vi "Cascade front panel.vi"() -> ()   [LabVIEW 2016]
uses:
  sdi_12/SDI-12/Sonde Vertical Graph.ctl
  controls/Vertical Chart.ctl
  sdi_12/Groundwater header.ctl
  controls/MCC DAQ Setup.ctl
  controls/Aux Sensor.ctl
  KPRO_2016 subvis/Control 2.ctl
  KPRO_2016 subvis/Graph Controls 2.ctl
  KPRO_2016 subvis/Ik control.ctl
  controls/MCC DAQ Readings.ctl
  controls/Kpro pressure measurement cluster.ctl
  controls/Kpro hydraulic measurement cluster.ctl
  activeXtest/activeXtest 2015 Folder/sonde cluster from excel.ctl
  sdi_12/Sonde Value Percent Tol.ctl
  activeXtest/activeXtest 2015 Folder/sample data row cluster.ctl
  activeXtest/activeXtest 2015 Folder/sonde cluster.ctl
  KPRO_2016 subvis/Sensor Physical Measurements.ctl
  KPRO_2016 subvis/SS Control 7.ctl
  controls/Action Control 1.ctl
  <extravilib>/ChannelInstances/One Element Stream-t'Action Control 1.ctl'/Instantiate.vi
  <extravilib>/ChannelInstances/One Element Stream-t'Action Control 1.ctl'/Endpoint.vi
  KPRO_lv2015/Kpro Globals.vi
  C/Program Files (x86)/National Instruments/LabVIEW 2016/user.lib/_OpenG.lib/file/file.llb/Strip Path - Traditional__ogtk.vi
  C/Program Files (x86)/National Instruments/LabVIEW 2016/user.lib/_OpenG.lib/file/file.llb/Build Path - Traditional__ogtk.vi
  <vilib>/Utility/file.llb/Write Delimited Spreadsheet (DBL).vi
  C/Program Files (x86)/National Instruments/LabVIEW 2016/user.lib/_OpenG.lib/file/file.llb/Strip Path Extension - Path__ogtk.vi
  C/Program Files (x86)/National Instruments/LabVIEW 2016/user.lib/_OpenG.lib/file/file.llb/Convert File Extension (String)__ogtk.vi
  <vilib>/Utility/file.llb/Write Delimited Spreadsheet (string).vi
  <vilib>/ULx/Create Channel.llb/ULx Create Channel (AI-Voltage-Basic).vi
  KPRO_lv2015/ad interface/Global_SIM_switch.vi
  C:/Program Files (x86)/National Instruments/LabVIEW 2016/vi.lib/ULx/ULx_LV.dll
  <vilib>/Utility/NIReport.llb/NI_report.lvclass
  <vilib>/Utility/config.llb/NI_LVConfig.lvlib
  <extravilib>/ChannelInstances/One Element Stream-t'Action Control 1.ctl'.lvlib
panel:
  out "Serial Number/MISC":string
  in  "Depth mode":bool caption="Use \nIncrement"
  in  "Sample Sheet Data Row Cluster 2":T1={"Head\nPressure"=0.0, "Depth"=0.0, "comment string"="", "Sonde Data Cluster"={"Cumulative\nVolume"=100.0, "Specific\nConductance"=2.0, "Dissolved\nOxygen"=3.0, "pH"=4.0, "ORP"=5.0, "Temp"=26.0, "Salinity"=7.0}} {"Sonde Data Cluster"."Salinity" format="%_3g"; "Sonde Data Cluster"."Temp" format="%_2g"; "Sonde Data Cluster"."ORP" format="%_4g"; "Sonde Data Cluster"."pH" format="%_4g"; "Sonde Data Cluster"."Dissolved\nOxygen" format="%_4g"; "Sonde Data Cluster"."Specific\nConductance" format="%_4g"; "Sonde Data Cluster"."Cumulative\nVolume" format="%#_4g"; "Depth" format="%#.3g"; "Head\nPressure" format="%#.4g"}
  in  "Sonde Parameters \nInitial Values":T3 {"Salinity Initial" format="%_2f"; "Temp Initial" format="%_2f"; "ORP  Initial" format="%_2f"; "pH Initial" format="%_2f"; "DO Initial" format="%_2f"; "SC Initial" format="%_2f"}
  in  "Sonde Parameters \nTolerance Limits":T4 {"Salinity %" format="%_2f%%"; "Temp %" format="%_2f%%"; "ORP %" format="%_2f%%"; "pH %" format="%_2f%%"; "DO %" format="%_2f%%"; "SC %" format="%_2f%%"}
  out "subarray":string[][](array[string])
  out "Initialization":i32
  in  "Increment Depth":bool
  in  "Finish Tests":bool
  in  "Start KPRO":bool
  in  "Record Continuous Samples":bool
  out "Current Time (s)":dbl
  in  "stop":bool
  in  "Write Data to Spreadsheet":bool
  in  "Sample Not Collected":bool
  in  "Record Single Sample":bool
  in  "Tab Control":T5(tab)
  out "KPRO Output File Path":path=path "C:/KPRO_2010/Output_files/Static Ik.txt"
  out "Output File Path":path=path "C:/KPRO_2010/Output_files/Static Ik.txt"
  in  "Slopes File Path":path=path "D:/Cascade/Data/Output Files/slopes.csv"
  out "12V Voltage Monitor":dbl format="%_3f"
  out "Found Quanta Sonde Com Port":refnum<visa-resource-name>
  in  "Temporary Data Files Directory":path=path "D:/Cascade/Data"
  in  "Data File Directory":path=path "D:/Cascade/Data/Excel Reports"
  out "Quanta Sonde found?":bool
  in  "template file path":path=path "D:/Cascade/templates/Groundwater Profiling Log_empty_labview_template.xlsx"
  in  "Config File Path":path=path "D:/Cascade/Data/config files/DAQ Setup Config.ini"
  in  "Read Configuration File?":bool
  out "H-4191 Adapter found":bool
  in  "Save Configuration File?":bool
  out "Sonde Communication Error Out":errorcluster
  in  "Search for Comm Ports?":bool=TRUE
  in  "USB Serial Port Manual Entry":refnum<visa-resource-name>="COM13"
  in  "Read String Pot":bool
  in  "Static IK path":path=path "D:/Cascade/Data/Output Files/Static Ik.csv"
  out "DTW path 2":path
  out "IKMGS appended path":path
  out "Sensor  Real Measurements":T6 {"9V Monitor" format="%#.3g"; "Aux 3" format="%#.3g"; "Aux 2" format="%#.3g"; "Aux 1" format="%#.3g"; "String Pot" format="%#.3g"; "Top String Pot" format="%#_4g"; "Downhole Pressure" format="%#_4g"; "Flow" format="%#_4g"; "Uphole Pressure" format="%#_4g"}
  in  "MCC USB-DAQ Setup":T7={"Device Name in InstaCal"="Dev0", "Omega Pressure Sensor"={"DAQ Channel"=2.0, "Output Voltage Range"=1, "Enabled"=TRUE, "Description"="Uphole Pressure"}, "McMillian 102 Flowmeter"={"DAQ Channel"=11.0, "Output Voltage Range"=0, "Enabled"=TRUE, "Description"="Flow"}, "DHT Pressure Sensor"={"DAQ Channel"=3.0, "Output Voltage Range"=1, "Enabled"=TRUE, "Description"="Downhole Pressure"}, "Top String Pot"={"DAQ Channel"=0.0, "Output Voltage Range"=0, "Enabled"=TRUE, "Description"="Top String Pot"}, "String Pot Signal"={"DAQ Channel"=1.0, "Output Voltage Range"=0, "Enabled"=TRUE, "Description"="String Pot"}, "Aux Sensor 1"={"DAQ Channel"=5.0, "Output Voltage Range"=1, "Enabled"=TRUE, "Description"="Aux 1"}, "Aux Sensor 2"={"DAQ Channel"=6.0, "Output Voltage Range"=1, "Enabled"=TRUE, "Description"="Aux 2"}, "Aux Sensor 3"={"DAQ Channel"=7.0, "Output Voltage Range"=1, "Enabled"=TRUE, "Description"="Aux 3"}, "Voltage Monitor"={"DAQ Channel"=8.0, "Output Voltage Range"=0, "Enabled"=TRUE, "Description"="9V Monitor"}} {"Voltage Monitor"."Output Voltage Range" items=["+/-10 V Range", "+/-5 V Range", "+/-2.5V Range", "+/-1.25 V Range", "+/-0.625 V Range", "+/-0.3125 V Range", "+/-0.1562V Range", "+/-0.078125 V Range"]; "Aux Sensor 3"."Output Voltage Range" items=["+/-10 V Range", "+/-5 V Range", "+/-2.5V Range", "+/-1.25 V Range", "+/-0.625 V Range", "+/-0.3125 V Range", "+/-0.1562V Range", "+/-0.078125 V Range"]; "Aux Sensor 2"."Output Voltage Range" items=["+/-10 V Range", "+/-5 V Range", "+/-2.5V Range", "+/-1.25 V Range", "+/-0.625 V Range", "+/-0.3125 V Range", "+/-0.1562V Range", "+/-0.078125 V Range"]; "Aux Sensor 1"."Output Voltage Range" items=["+/-10 V Range", "+/-5 V Range", "+/-2.5V Range", "+/-1.25 V Range", "+/-0.625 V Range", "+/-0.3125 V Range", "+/-0.1562V Range", "+/-0.078125 V Range"]; "String Pot Signal"."Output Voltage Range" items=["+/-10 V Range", "+/-5 V Range", "+/-2.5V Range", "+/-1.25 V Range", "+/-0.625 V Range", "+/-0.3125 V Range", "+/-0.1562V Range", "+/-0.078125 V Range"]; "Top String Pot"."Output Voltage Range" items=["+/-10 V Range", "+/-5 V Range", "+/-2.5V Range", "+/-1.25 V Range", "+/-0.625 V Range", "+/-0.3125 V Range", "+/-0.1562V Range", "+/-0.078125 V Range"]; "DHT Pressure Sensor"."Output Voltage Range" items=["+/-10 V Range", "+/-5 V Range", "+/-2.5V Range", "+/-1.25 V Range", "+/-0.625 V Range", "+/-0.3125 V Range", "+/-0.1562V Range", "+/-0.078125 V Range"]; "McMillian 102 Flowmeter"."Output Voltage Range" items=["+/-10 V Range", "+/-5 V Range", "+/-2.5V Range", "+/-1.25 V Range", "+/-0.625 V Range", "+/-0.3125 V Range", "+/-0.1562V Range", "+/-0.078125 V Range"]; "Omega Pressure Sensor"."Output Voltage Range" items=["+/-10 V Range", "+/-5 V Range", "+/-2.5V Range", "+/-1.25 V Range", "+/-0.625 V Range", "+/-0.3125 V Range", "+/-0.1562V Range", "+/-0.078125 V Range"]}
  out "Rate":dbl=1000.0 caption="Sample Rate (Hz)"
  out "Number \nof Channels":u16
  in  "Channel \nData Rate S/s":dbl=3720.0 format="%#_13g"
  out "Descriptions":string[](array[string])
  out "Raw Voltages":dbl[](array[numeric])
  out "9V Voltage Monitor":dbl format="%#_3g"
  in  "Record DAQ Raw Voltages":bool
  out "Sensor Voltage Cluster":T9 {"9V Monitor" format="%#.3g"; "Aux 3" format="%#_3g"; "Aux 2" format="%#.3g"; "Aux 1" format="%#.3g"; "String Pot" format="%#.3g"; "Top String Pot" format="%#_3g"; "Downhole Pressure" format="%#.3g"; "Flow" format="%#_3g"; "Uphole Pressure" format="%-#1.3g"}
  in  "Clear Groundwater Header Values":bool
  in  "Groundwater Header":T10
  out "Worksheet Names":string[](array[string])
  in  "Current Sheet":i32=1
  out "row max value":i32
  out "last occupied cell's name":string
  out "Current Sample Sheet":string="Sample 1"
  in  "Excel report file path":path=path "D:/Cascade/templates/Groundwater Profiling Log_empty_2.xlsx"
  out "Data Setup Indicator":string
  in  "Start Initialization":bool
  out "Sonde Data Array":T11[](array[typedef]) {"Salinity"."%" format="%_2f%%"; "Salinity"."Value" format="%_4g"; "Temperature"."%" format="%_2f%%"; "Temperature"."Value" format="%_4g"; "ORP"."%" format="%_2f%%"; "ORP"."Value" format="%_4g"; "pH"."%" format="%_2f%%"; "pH"."Value" format="%_4g"; "Dissolved Oxygen"."%" format="%_2f%%"; "Dissolved Oxygen"."Value" format="%_4g"; "Sp. Conductance"."%" format="%_2f%%"; "Sp. Conductance"."Value" format="%_4g"; "Cumulative\nVolume" format="%#_4g"}
  out "Table Label":string="Data from Sample Sheet %d from Excel File"
  out "Sonde Data Display":T13
  out "Temperature":cluster{"Y":dbl[], "Y":dbl[]}[](graph)
  in  "Record Reason":bool
  in  "Select Reasons to Record Data":u16(ring) items=["Per Client Request", "Timed Out", "Sample stopped flowing", "Equipment Issue"]
  out "Sonde Recording Failure Path":path
  out "SC  Reference\nCalibrate Response":bool
  out "DO  Reference\nCalibrate Response":bool
  in  "Salinity \nReference":dbl
  out "Salinity  Reference\nCalibrate Response":bool
  out "ORP  Reference\nCalibrate Response":bool
  in  "SC \nReference":dbl
  in  "DO \nReference":dbl
  in  "ORP Reference":dbl
  in  "pH Reference":dbl
  in  "pH Zero":dbl
  in  "Record  SC Calibration":bool
  in  "Record DO Calibration":bool
  in  "Record Salinity Calibration":bool
  in  "Record ORP Calibration":bool
  in  "Record pH Calibration Reference":bool
  in  "Record pH Calibration Zero":bool
  out "pH Zero \nCalibrate Response":bool
  out "pH  Reference\nCalibrate Response":bool
  out "KPRO Finish\nIndicator":bool
  out "Input Depths \nand Parameters Cluster":T15={"Flow"=0.21081600494384767, "Zeroed \nPressure"=74.74207969932556, "Ik"=0.003788962123473114, "Current Depth"=-100.6, "Feet of Stainless"=40, "Start Depth"=0.0, "Abs Start Depth"=0.0} {"Abs Start Depth" format="%.2f"; "Start Depth" format="%.2f"; "Current Depth" format="%.2f"; "Ik" format="%.2f"; "Zeroed \nPressure" format="%.2f"; "Flow" format="%.2f"}
  out "Zero Pressure\nIndicator":bool
  in  "Zero\nPressure":bool caption="Zero Pressure"
  in  "enable_IKMGS_file":bool
  in  "enable_slug_file":bool
  in  "enable_kpro_file":bool=TRUE
  in  "Simulate AD6B":bool
  out "KPRO Test\nIndicator":bool
  in  "Input Variables and Slopes":T16={"Total Volume"=0.0, "String Pot Slope"=1.6619999408721924, "Flow Slope"=39.040000915527344, "Up Hole Pressure Slope"=48.27000045776367, "Depth to Water Table"=-0.0, "Atmospheric Pressure"=32.22022530555725, "Reservoir Pressure"=-0.004827000045779073, "Height of Sample Box"=0.0, "DH Pressure Trans Slope"=42.0, "DH Pressure Offset"=0.0, "Up Hole  Pressure Offset"=0.0, "Aux 1 Slope"=1.0, "Aux 2 Slope"=1.0, "Aux 3 Slope"=1.0} {"Aux 3 Slope" format="%.2f"; "Aux 2 Slope" format="%.2f"; "Aux 1 Slope" format="%.2f"; "Up Hole  Pressure Offset" format="%.2f"; "DH Pressure Offset" format="%.2f"; "DH Pressure Trans Slope" format="%.2f"; "Height of Sample Box" format="%.2f"; "Reservoir Pressure" format="%.2f"; "Atmospheric Pressure" format="%.2f"; "Depth to Water Table" format="%.2f"; "Up Hole Pressure Slope" format="%.2f"; "Flow Slope" format="%.2f"; "String Pot Slope" format="%.2f"; "Total Volume" format="%.2f"}
  in  "Record DTW File":bool
  in  "Zero In-Line Pressure\n(F = leave as is)":bool=TRUE
  in  "Depth Cluster":T17
  out "Cumulative_data_ready":bool
  out "Cumulative_data_from_file":sgl[][](array[numeric]) format="%.2f"
  in  "KPRO test report header":string[](array[string])=["Time(msecs)", "Uncorrected Depth", "Corrected Depth", "Drive_Rate", "Flow", "Feet_of Stainless", "Up Hole Pressure", "IK", "Corrected Pressure", "Atm Pressure", "Depth to water", "Height of box", "Res_Pressure", "Secs_since_1_JAN_1904", "Depth jumps more than 1_foot", "Down hole Pressure"]
  out "Depth Rate\nft/min":dbl format="%#.2g"
  out "Ik":dbl=0.003788962123473114 caption="Real Time - Depth vs. lk" format="%.2f"
  out "Zeroed Pressure":dbl format="%.2f"
  in  "New Depth":dbl
  in  "Update Depth":bool
  in  "Select Entry for Log File":u16(ring) items=["Per Client Request", "Timed Out", "Sample stopped flowing", "Equipment Issue"]
  out "Large Depth IK Graph Cluster":T18={[0.003788962123473114, 0.0037174584307500765, 0.0037174584307500765, 0.0037174584307500765, 0.0037174584307500765, 0.003788962123473114], [-100.1, -100.2, -100.3, -100.4, -100.5, -100.6]}
  in  "Culmulative Graph Cluster":T19={"Cumulative - Depth vs. Ik"={[], []}, "Real Time - Depth vs. lk "={[0.003788962123473114, 0.0037174584307500765, 0.0037174584307500765, 0.0037174584307500765, 0.0037174584307500765, 0.003788962123473114], [-100.1, -100.2, -100.3, -100.4, -100.5, -100.6]}, "Cumulative - Depth vs. Drive Rate"={[], []}, "Real Time - Depth vs. Drive Rate"={[0.02036245163917736, 0.125, 0.16666666666666674, 0.16666666666666663, 0.16666666666666663, 0.16666666666666663], [-100.1, -100.2, -100.3, -100.4, -100.5, -100.6]}}
  out "Down hole Pressure":dbl format="%.2f"
  in  "Record Reason 2":bool
  in  "Corrected Pressure Cluster":T20
  out "Flow":dbl format="%#.2g"
  out "Current Depth":sgl=-100.6 format="%.2f"
  out "Current \nDepth (m)":sgl=-30.661383 format="%.2f"
  out "Large Depth IK Graph":dbl(graph)
  out "DAQ Error":errorcluster
  out "Initialization Finished":bool=TRUE
  out "Stop":bool
  out "error out":errorcluster
  in  "error in (no error)":errorcluster
  out "producer loop":i32
  out "consumer loop":i32
  out "Active Channel Array":string[](array[string])
  out "delimited string":string
  out "Voltage Range":dbl[](array[numeric])
  out "Stop 2":bool
  # "ft. water"
  # "mL/min."
  # "ft. water"
  # "ft."
  # "ft."
  # "Instructions for Sonde Calibration:\n1.  Use the Record Single Point to Record the Data prior to start of\ncalibration procedure to record the initial points to the excel worksheet.\n2.  pH Calibration is a 2 step process:  A pH standard between 6.8 and 7.2 is treated as the “zero”\nand all other values are treated as the “slope”. First calibrate “zero”, then  add a second to calibrate “slope”. \n3.  Specific Conductance:  Wait for the specific conductance readings to stabilize in the calibration solution, which may\nrequire one or two minutes."
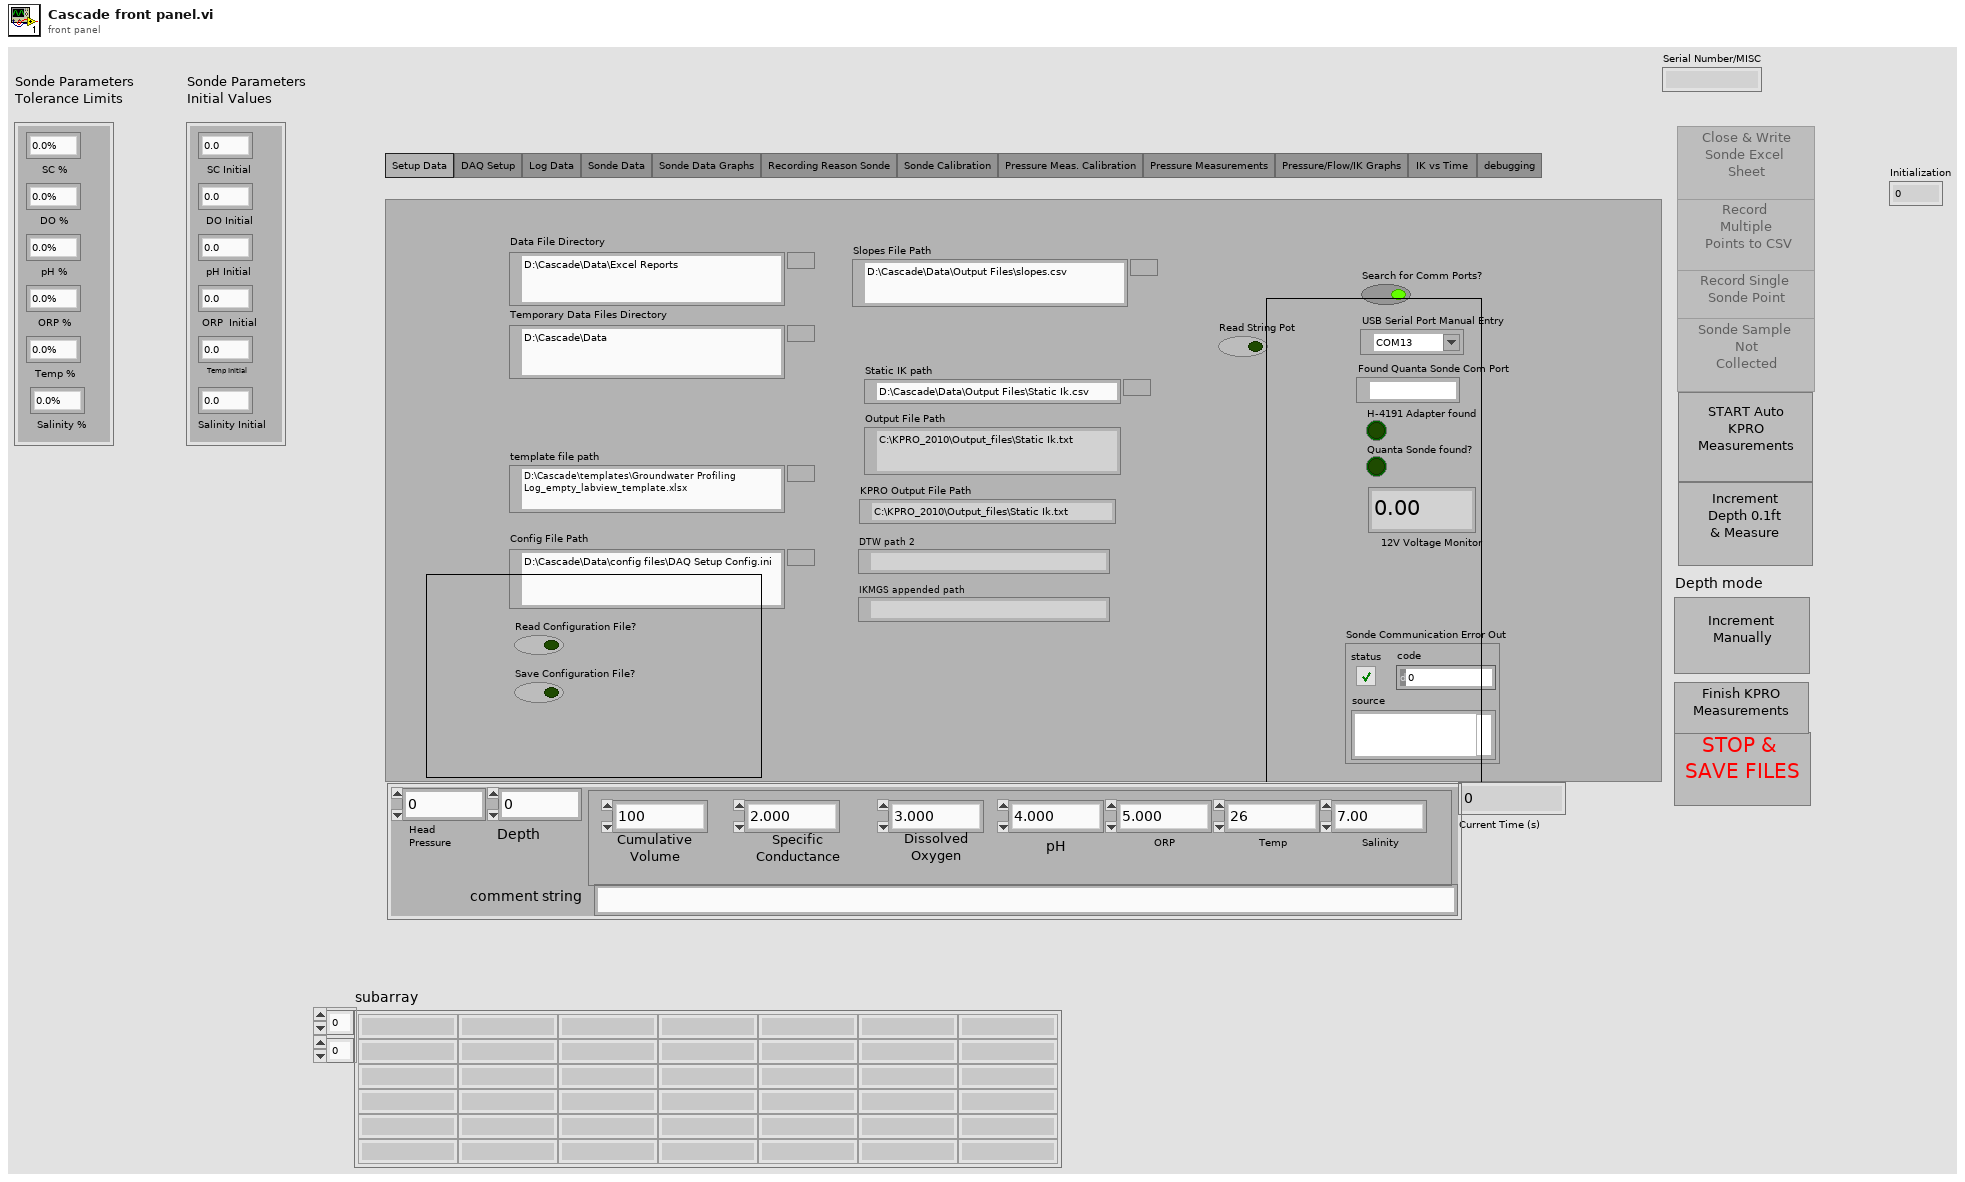
[diagram p1: front panel]
types:
  T1 = typedef "sample data row cluster.ctl" = cluster{"Head\nPressure":dbl, "Depth":dbl, "comment string":string, "Sonde Data Cluster":T2}
  T2 = typedef "sonde cluster.ctl" = cluster{"Cumulative\nVolume":dbl, "Specific\nConductance":dbl, "Dissolved\nOxygen":dbl, "pH":dbl, "ORP":dbl, "Temp":dbl, "Salinity":dbl}
  T3 = cluster{"SC Initial ":dbl, "DO Initial ":dbl, "pH Initial  ":dbl, "ORP  Initial":dbl, "Temp Initial":dbl, "Salinity Initial ":dbl}
  T4 = cluster{"SC %":dbl, "DO %":dbl, "pH % ":dbl, "ORP % ":dbl, "Temp % ":dbl, "Salinity %":dbl}
  T5 = enum32{"Setup Data", "DAQ Setup", "Log Data", "Sonde Data", "Sonde Data Graphs", "Recording Reason Sonde", "Sonde Calibration", "Pressure Meas. Calibration", "Pressure Measurements", "Pressure/Flow/IK Graphs", "IK vs Time ", "debugging"}
  T6 = typedef "Sensor Physical Measurements.ctl" = cluster{"Uphole Pressure":dbl, "Flow":dbl, "Downhole Pressure":dbl, "Top String Pot":dbl, "String Pot":dbl, "Aux 1":dbl, "Aux 2":dbl, "Aux 3":dbl, "9V Monitor":dbl}
  T7 = typedef "MCC DAQ Setup.ctl" = cluster{"Device Name in InstaCal":string, "Omega Pressure Sensor":T8, "McMillian 102 Flowmeter":T8, "DHT Pressure Sensor":T8, "Top String Pot":T8, "String Pot Signal":T8, "Aux Sensor 1":T8, "Aux Sensor 2":T8, "Aux Sensor 3":T8, "Voltage Monitor":T8}
  T8 = typedef "Aux Sensor.ctl" = cluster{"DAQ Channel":dbl, "Output Voltage Range":u16, "Enabled":bool, "Description":string}
  T9 = typedef "MCC DAQ Readings.ctl" = cluster{"Uphole Pressure":dbl, "Flow":dbl, "Downhole Pressure":dbl, "Top String Pot":dbl, "String Pot":dbl, "Aux 1":dbl, "Aux 2":dbl, "Aux 3":dbl, "9V Monitor":dbl}
  T10 = typedef "Groundwater header.ctl" = cluster{"Location":string, "Date Finished":string, "CTS":string, "sampler":string, "Kpro box Serial ":string, "Sonde Serial":string, "Drilling Contractor":string, "Ave Depth to Water":string, "Gas/Peri Pump":string, "Atmospheric Pressure":string, "KPRO N2 Pressure":string, "Gas Drive N2 Pressure":string, "Profile ID":string}
  T11 = typedef "sonde cluster from excel.ctl" = cluster{"Head":dbl, "Depth":dbl, "Time":string, "Cumulative\nVolume":dbl, "Sp. Conductance":T12, "Dissolved Oxygen":T12, "pH":T12, "ORP":T12, "Temperature":T12, "Salinity":T12, "Final Tol.":bool, "Final":bool}
  T12 = typedef "Sonde Value Percent Tol.ctl" = cluster{"Value":dbl, "%":dbl, "Tol.":bool}
  T13 = typedef "Sonde Vertical Graph.ctl" = cluster{"pH":T14, "Conductance":T14, "Salinity":T14, "DO % Saturation":T14, "DO mg/L":T14, "ORP":T14}
  T14 = typedef "Vertical Chart.ctl" = cluster{"Y":dbl[], "Y":dbl[]}[]
  T15 = typedef "SS Control 7.ctl" = cluster{"Flow":dbl, "Zeroed \nPressure":dbl, "Ik":dbl, "Current Depth":sgl, "Feet of Stainless":i32, "Start Depth":sgl, "Abs Start Depth":sgl}
  T16 = typedef "Control 2.ctl" = cluster{"Total Volume":dbl, "String Pot Slope":dbl, "Flow Slope":dbl, "Up Hole Pressure Slope":dbl, "Depth to Water Table":dbl, "Atmospheric Pressure":dbl, "Reservoir Pressure":dbl, "Height of Sample Box":dbl, "DH Pressure Trans Slope":dbl, "DH Pressure Offset":dbl, "Up Hole  Pressure Offset":dbl, "Aux 1 Slope":dbl, "Aux 2 Slope":dbl, "Aux 3 Slope":dbl}
  T17 = typedef "Kpro hydraulic measurement cluster.ctl" = cluster{"Absolute Depth In":dbl, "Current Absolute Depth":dbl, "First Absolute Depth":dbl, "Previous Relative Depth":dbl, "Current Relative Depth":dbl, "First Relative Depth":dbl, "Last Filed Depth":dbl, "Total Volume In":dbl, "Total Volume Out":dbl, "Current Measurement Time":dbl, "Previous Measurement Time":dbl}
  T18 = typedef "Ik control.ctl" = cluster{dbl[], dbl[]}
  T19 = typedef "Graph Controls 2.ctl" = cluster{"Cumulative - Depth vs. Ik":cluster{dbl[], dbl[]}, "Real Time - Depth vs. lk ":cluster{dbl[], dbl[]}, "Cumulative - Depth vs. Drive Rate":cluster{dbl[], dbl[]}, "Real Time - Depth vs. Drive Rate":cluster{dbl[], dbl[]}}
  T20 = typedef "Kpro pressure measurement cluster.ctl" = cluster{"Up hole Corrected Pressure":dbl, "Down hole Corrected Pressure":dbl}
  T21 = typedef "NI_LVConfig.lvlib/Config Data RefNum.ctl" = refnum<k1>
  T22 = enum8{"Enabled", "Disabled", "Disabled and Grayed Out"}
  T23 = typedef "Action Control 1.ctl" = enum16{"TimeOut", "Continuous  Sonde Data", "Init", "Exit", "Acq. Single Sonde Point", "Write Sonde Sample Sheet", "Acq. DAQ data", "Sample Not Collected", "Record Reason", "pH Calibration Zero", "pH Calibration Standard", "ORP Calibration Standard", "Salinity Calibration Standard", "DO Calibration Standard", "SC Calibration Standard", "Increment Depth Manually", "Start KPRO Measurements", "Finish KPRO Measurements", "Update Depth", "IK vs Time"}
  T24 = typedef "One Element Stream-t'Action Control 1.ctl'.lvlib/)Channel.ctl" = refnum<queue>
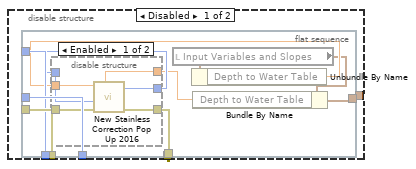
[diagram p15: hidden frame]
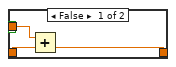
[diagram p18: hidden frame]
diagram:
  # "For calibrate command (XC) on SDI-12 address ‘a’, P is pH, C is specific conductance, S is\nsalinity or TDS, % is DO %Saturation, O is DO mg/L, R is ORP, D is depth, B is\nbarometric pressure, and t is TDS scale factor."
  n1 = flat-sequence {
    tunnel: [w22] -> w5
    tunnel: [w54] -> w9
    tunnel: w5 -> [w54]
    tunnel: [w50] -> w3
    tunnel: [w59] -> w16
    tunnel: w9 -> [w68]
    tunnel: [w68] -> w6
    tunnel: w16 -> [w94]
    tunnel: [w99] -> w14
    tunnel: [w101] -> w13
    tunnel: [w103] -> w10
    tunnel: [w96] -> w11
    tunnel: [w102] -> w12
    tunnel: [w100] -> _
    tunnel: [w95] -> w15
    tunnel: [w97] -> w2
    tunnel: [w98] -> w1
    frame #0 {
      n2 = invoke on="error out" class="Clust (strict)" method="Reinit To Default"(error in="error in (no error)") -> (error out=w20:errorcluster)  [unwired: 2 in, 2 out]
      n3 = flat-sequence {
        tunnel: [w26] -> w22
        tunnel: w20 -> [w25]
        frame #0 {
          n4 = case shown="True" "Read Configuration File?" {
            selector: "Read Configuration File?" -> [_ w33]
            tunnel: [w27 w38] -> w26
            tunnel: w25 -> [w27 w35]
            tunnel: "Config File Path" -> [_ w34]
            frame False {
            }
            frame True {
              n5 = call <vilib>:"Check if File or Folder Exists.vi"("error in (no error)"=w35, "path"=w34) -> ("error out"=w30:errorcluster, "file or folder exists?"=w31:bool, "dup path"=w29:path)  [unwired: 7 in]
              n6 = And(x=w33, y=w31) -> (x .and. y?=w32:bool)
              n7 = control-ref of="This VI"() -> (w36:refnum<vi>)
              n8 = case shown="True" w32 {
                selector: w32 -> [w39 _]
                tunnel: w29 -> [_ w44]
                tunnel: w30 -> [w40 w48]
                tunnel: [w40 w41] -> w37
                tunnel: w36 -> [_ w49]
                frame False {
                  n9 = local write "Read Configuration File?"(w39) -> ()
                }
                frame True {
                  n10 = call <vilib>:"Open Config Data.vi"("error in (no error)"=w48, "create file if necessary (T)"=FALSE, "configuration file path"=w44) -> ("error out"=w46:errorcluster, "refnum"=w47:T21)  [unwired: 6 in, 1 out]
                  n11 = call "Read Panel from INI__ogtk.vi"("error in (no error)"=w46, "VI ref"=w49, "refnum"=w47) -> ("error out"=w42:errorcluster, "refnum out"=w43:T21)  [unwired: 7 in]
                  n12 = call <vilib>:"Close Config Data.vi"("error in (no error)"=w42, "refnum"=w43) -> ("error out"=w41:errorcluster)  [unwired: 8 in, 1 out]
                }
              }
              n13 = call <vilib>:"Clear Errors.vi"("error in (no error)"=w37) -> ("error out"=w28:errorcluster)  [unwired: 5 in, 1 out]
              n14 = Merge Errors(w28) -> (w38:errorcluster)
            }
          }
        }
      }
    }
    frame #1 {
      n15 = Get Date/Time In Seconds() -> (seconds since 1Jan1904=w50:timestamp)
      n16 = local write "Current Sheet"(1 ("Current Sheet")) -> ()
      n17 = Get Date/Time In Seconds() -> (seconds since 1Jan1904=w51:timestamp)
      n18 = Subtract(x=w50, y=w51) -> (x-y=w52:dbl)
      n19 = To Double Precision Float(number=w52) -> (double precision float=→"Current Time (s)":dbl)
    }
    frame #2 {
      w79 = T22."Disabled and Grayed Out" ("Disabled")
      n20 = invoke on="Current Sheet" class="DigNum (strict)" method="Reinit To Default"() -> (error out=w72:errorcluster)  [unwired: 3 in, 2 out]
      n21 = local write "Initialization Finished"(FALSE ("Initialization Finished")) -> ()
      n22 = invoke on="Sample Not Collected" class="Bool" method="Reinit To Default"(error in=w72) -> (error out=w76:errorcluster)  [unwired: 2 in, 2 out]
      n23 = control-ref of="Sonde Data Display"() -> ()  [unwired: 1 out]
      n24 = invoke on="Record Continuous Samples" class="Bool" method="Reinit To Default"(error in=w76) -> (error out=w75:errorcluster)  [unwired: 2 in, 2 out]
      n25 = property on="Record Continuous Samples" class="Bool"("DisabledEnum"=w79) -> (error out=w80:errorcluster)  [unwired: 2 in, 1 out]
      n26 = call "search for Quanta Sonde devices.vi"("VISA resource name"="USB Serial Port Manual Entry", "Search for Comm Ports?"="Search for Comm Ports?", "error in (no error)"=w68) -> ("12V monitor"=→"12V Voltage Monitor":dbl, "Com Port with Quanta Sonde devices"=w85:refnum<visa-resource-name>[], "Number of Quanta Sonde devices"=w84:i32, "Serial Number/MISC"=w57:string, "Number of Quanta Sonde devices > 0?"=→"Quanta Sonde found?":bool, "H-4191 Adapter found"=→"H-4191 Adapter found":bool, "Error Out"=w65:errorcluster)  [unwired: 4 in, 2 out]
      "Sonde Communication Error Out" <- w65
      "Serial Number/MISC" <- w57
      n27 = case shown="1" w84 {
        tunnel: w85 -> [_ w92]
        tunnel: [refnum<visa-resource-name> refnum ("RS232 Port Out") w90] -> w83
        frame 0, Default {
        }
        frame 1 {
          n28 = Index Array(array=w92, index=0) -> (element=w90:refnum<visa-resource-name>)
        }
      }
      "Found Quanta Sonde Com Port" <- w83
      n29 = invoke on="Write Data to Spreadsheet" class="Bool" method="Reinit To Default"(error in=w75) -> (error out=w74:errorcluster)  [unwired: 2 in, 2 out]
      n30 = local read "Groundwater Header"() -> (w56:T10)
      n31 = Bundle By Name(cluster=w56, "Sonde Serial"=w57) -> (w58:T10)
      n32 = property on="Record Single Sample" class="Bool"(error in=w80, "DisabledEnum"=w79) -> (error out=w81:errorcluster)  [unwired: 1 in, 1 out]
      n33 = invoke on="Record Single Sample" class="Bool" method="Reinit To Default"(error in=w74) -> (error out=w73:errorcluster)  [unwired: 2 in, 2 out]
      n34 = local write "Groundwater Header"(w58) -> ()
      n35 = call <vilib>:"Clear Errors.vi"("error in (no error)"=w65) -> ("error out"=w64:errorcluster)  [unwired: 5 in, 1 out]
      n36 = invoke on="stop" class="Bool" method="Reinit To Default"(error in=w73) -> (error out=w78:errorcluster)  [unwired: 2 in, 2 out]
      n37 = flat-sequence {
        tunnel: [w88] -> w60
        tunnel: w61 -> [w88]
        frame #0 {
          n38 = local write "Tab Control"(T5."Log Data" ("Tab Control")) -> ()
        }
      }
      n39 = invoke on="Stop" class="Bool (strict)" method="Reinit To Default"() -> (error out=w67:errorcluster)  [unwired: 3 in, 2 out]
      n40 = property on="Write Data to Spreadsheet" class="Bool"(error in=w78, "DisabledEnum"=w79) -> (error out=w70:errorcluster)  [unwired: 1 in, 1 out]
      n41 = property on="Sample Not Collected" class="Bool"(error in=w81, "DisabledEnum"=w79) -> (error out=w77:errorcluster)  [unwired: 1 in, 1 out]
      n42 = invoke on="Stop 2" class="Bool (strict)" method="Reinit To Default"(error in=w67) -> (error out=w66:errorcluster)  [unwired: 2 in, 2 out]
      n43 = Merge Errors(w64, w66, w70, w77) -> (w61:errorcluster)
      n44 = invoke on="Data Setup Indicator" class="Str" method="Reinit To Default"(error in=w60) -> (error out=w59:errorcluster)  [unwired: 2 in, 2 out]
      n45 = invoke on="Cumulative_data_from_file" class="Arr (strict)" method="Reinit To Default"() -> ()  [unwired: 3 in, 3 out]
    }
    frame #3 {
      n46 = while {
        tunnel: w94 -> [w109]
        tunnel: [w106] -> w93
        tunnel: [w108] -> _
        i -> [w108]
        stop <- w111 stop-if-true
        n47 = Quotient & Remainder(x=w108, y=1000) -> (floor(x/y)=w104:i32)  [unwired: 1 out]
        n48 = call "Wait (ms)__ogtk.vi"("error in (no error)"=w109, "milliseconds to wait"=u32 100) -> ("error out"=w106:errorcluster)  [unwired: 8 in, 1 out]
        n49 = event shown="[2] \"Clear Groundwater Header Values\": Value Change" {
          selector: _ -> [_ _ _]
          dyn-events: _ -> [_ _ _]
          timeout: 100 -> [_ _ _]
          tunnel: [FALSE w119 _] -> w111
          event Timeout {
            n50 = event-data() -> ()  [unwired: 1 in, 3 out]
          }
          event "Start Initialization": Value Change {
            n51 = event-data() -> ()  [unwired: 1 in, 3 out]
            n52 = case shown="True" "Start Initialization" {
              tunnel: [FALSE ("Stop") TRUE ("Stop")] -> w119
              frame False {
              }
              frame True {
                n53 = invoke on="Start Initialization" class="Bool" method="Reinit To Default"() -> ()  [unwired: 3 in, 3 out]
                n54 = invoke on="Data Setup Indicator" class="Str" method="Reinit To Default"() -> ()  [unwired: 3 in, 3 out]
              }
            }
          }
          event "Clear Groundwater Header Values": Value Change {
            n55 = event-data() -> ()  [unwired: 1 in, 6 out]
            n56 = case shown="True" "Clear Groundwater Header Values" {
              frame False {
              }
              frame True {
                n57 = invoke on="Groundwater Header" class="Clust (strict)" method="Reinit To Default"() -> (error out=w123:errorcluster)  [unwired: 3 in, 2 out]
                n58 = flat-sequence {
                  tunnel: w123 -> [_]
                  frame #0 {
                    n59 = local read "Serial Number/MISC"() -> (w125:string)
                    n60 = local read "Groundwater Header"() -> (w124:T10)
                    n61 = Bundle By Name(cluster=w124, "Sonde Serial"=w125) -> (w126:T10)
                    n62 = local write "Groundwater Header"(w126) -> ()
                  }
                }
              }
            }
          }
        }
        n63 = case shown="0" w104 {
          tunnel: w106 -> [w114 w116]
          frame 1, Default {
            n64 = property on="Data Setup Indicator" class="Str"(error in=w114, "Text.TextColor"=u32 0) -> ()  [unwired: 1 in, 2 out]
          }
          frame 0 {
            n65 = property on="Data Setup Indicator" class="Str"(error in=w116, "Text.TextColor"=u32 16716800) -> ()  [unwired: 1 in, 2 out]
          }
        }
        "Data Setup Indicator" <- "Hit the Start Key after Data Entry of Log Parameters and File Names." ("Data Setup Indicator")
      }
      n66 = flat-sequence {
        tunnel: w93 -> [w145]
        tunnel: [w138] -> w103
        tunnel: [w137] -> w102
        tunnel: [w135] -> w101
        tunnel: [w134] -> w100
        tunnel: [w133] -> w99
        tunnel: [w132] -> w95
        tunnel: [w127] -> w96
        frame #0 {
          n67 = call "get sample header columns.vi"("report file path"=path "D:/Cascade/templates/Fields for Excel sheets.xlsx", "error in (no error)"=w145) -> ("Column of Volume"=w127:i32, "Columns"=w137:i32[], "data"=w144:string[][], "error out"=w146:errorcluster)  [unwired: 4 in, 6 out]
          "row max value" <- w127
          n68 = call "format into Sonde Data Array.vi"("data"=w144) -> ()  [unwired: 10 in, 1 out]
          n69 = call "close excel file if open.vi"("error in (no error)"=w146, "report file path in"="Excel report file path") -> ("error out"=w139:errorcluster, "report file path out"=w131:path)  [unwired: 8 in]
          n70 = call "copy excel template.vi"("error in (no error)"=w139, "report file path in"=w131, "template file path in"="template file path") -> ("error out"=w140:errorcluster, "report file path out"=w142:path)  [unwired: 6 in, 1 out]
          n71 = call "open excel get worksheet names.vi"("error in (no error)"=w140, "milliseconds to wait"=u32 5, "report file path"=w142) -> ("error out"=w128:errorcluster, "Number of Sample Sheets"=w138:i32, "NI_report out"=w129:refnum<class "NI_report.lvclass">, "Worksheet Names"=w135:string[])  [unwired: 3 in, 2 out]
          "Worksheet Names" <- w135
          n72 = flat-sequence {
            tunnel: w135 -> [w164]
            tunnel: [w162] -> w134
            tunnel: [w160] -> w133
            tunnel: [w158] -> w132
            tunnel: w129 -> [w157]
            tunnel: w128 -> [w156]
            frame #0 {
              w163 = "Sample 1" ("Worksheet Name in")
              n73 = local write "Current Sample Sheet"(w163) -> ()
              n74 = call "find and open select worksheet.vi"("Worksheet Names"=w164, "error in (no error)"=w156, "milliseconds to wait"=u32 100, "Worksheet Name in"=w163, "NI_report in"=w157) -> ("error out"=w159:errorcluster, "Select Worksheet Index"=w162:i32, "NI_report out"=w161:refnum<class "NI_report.lvclass">)  [unwired: 4 in]
              n75 = local read "Current Sample Sheet"() -> (w149:string)
              n76 = call "get sample sheet data cells.vi"("error in (no error)"=w159, "NI_report in"=w161) -> ("error out"=w152:errorcluster, "data"=w153:string[][], "NI_report out"=w160:refnum<class "NI_report.lvclass">, "left edge output cluster"=w151:cluster{"row":i32, "column":i32})  [unwired: 5 in, 1 out]
              n77 = call "find last occupied cell.vi"("data"=w153, "Active Sheet"=w149, "Header Rows to remove"=3, "sub array start"=w151, "error in (no error)"=w152) -> ("row max value"=w150:i32, "start of last occupied row"=w148:string, "error out"=w158:errorcluster)  [unwired: 4 in, 4 out]
              n78 = Array Subset(array=w153, index (col)=2 ("index")) -> (→"subarray":string[][])  [unwired: 3 in]
              n79 = local write "last occupied cell's name"(w148) -> ()
              n80 = local write "row max value"(w150) -> ()
            }
          }
        }
      }
      n81 = flat-sequence {
        tunnel: [w168] -> w98
        tunnel: [w168] -> w97
        tunnel: [w173] -> _
        tunnel: w95 -> [w172]
        frame #0 {
          n82 = Unbundle By Name("Input Variables and Slopes") -> ("Depth to Water Table"=w178:dbl)
          n83 = local read "Input Depths \nand Parameters Cluster"() -> (w170:T15)
          n84 = Unbundle By Name(w170) -> ("Feet of Stainless"=w168:i32)
          n85 = Bundle By Name(cluster="Input Variables and Slopes", "Depth to Water Table"=w178) -> (w175:T16)
          n86 = Bundle By Name(cluster=w170, "Feet of Stainless"=w168) -> (w169:T15)
          n87 = local write "Input Depths \nand Parameters Cluster"(w169) -> ()
          n88 = call <vilib>:"Check if File or Folder Exists.vi"("error in (no error)"=w172, "path"="Slopes File Path") -> ("error out"=w171:errorcluster, "dup path"=w176:path)  [unwired: 7 in, 1 out]
          n89 = case shown="True" TRUE {
            tunnel: w176 -> [_ w189]
            tunnel: w175 -> [w182 w188]
            tunnel: [w182 w187] -> w174
            tunnel: w171 -> [w181 w183]
            tunnel: [w181 w183] -> w173
            frame False {
              n90 = local write "Data Setup Indicator"("Slope file not found." ("Data Setup Indicator")) -> ()
            }
            frame True {
              n91 = call "Get_SLOPE_data_from_file 2016.vi"("Slopes File Path"=w189) -> ("Last_Pressure_Slope"=w184:dbl, "Last_Flow_Slope"=w185:dbl, "Last_String_Pot_Slope"=w186:dbl)  [unwired: 7 in, 1 out]
              n92 = Bundle By Name(cluster=w188, "String Pot Slope"=w186, "Flow Slope"=w185, "Up Hole Pressure Slope"=w184) -> (w187:T16)
            }
          }
          n93 = local write "Input Variables and Slopes"(w174) -> ()
        }
      }
      n94 = flat-sequence {
        tunnel: w95 -> [_]
        frame #0 {
          n95 = local write "KPRO Finish\nIndicator"(FALSE ("KPRO Finish\nIndicator")) -> ()
        }
      }
    }
  }
  n96 = flat-sequence {
    tunnel: [w193] -> w19
    tunnel: w15 -> [w192]
    tunnel: [w191] -> w4
    frame #0 {
      w190 = Action_Control_1."Init"  # Event
      n97 = while {
        shift-right: [w201] -> w193
        shift-left: w192 -> [w201]
        shift-right: [w196] -> _
        shift-left: w190 -> [w194]
        tunnel: [w202] -> w191
        i -> [w200]
        stop <- w198 stop-if-true
        # "User Interface Producer Loop"
        n98 = First Call?() -> (First Call?: T/F=w195:bool)
        n99 = case shown="False" w195 {
          tunnel: w201 -> [w207 _]
          tunnel: [w205 FALSE ("Boolean")] -> w198
          tunnel: [w204 w379] -> w196
          tunnel: w194 -> [_ w379]
          frame False {
            w203 = Action_Control_1."TimeOut"  # Event
            n100 = event shown="[10] \"Record Single Sample\": Value Change" {
              selector: _ -> [_ _ _ _ _ _ _ _ _ _ _ _ _ _ _ _ _]
              dyn-events: _ -> [_ _ _ _ _ _ _ _ _ _ _ _ _ _ _ _ _]
              timeout: 100 -> [_ _ _ _ _ _ _ _ _ _ _ _ _ _ _ _ _]
              tunnel: [w208 w214 w220 w233 w245 w257 w269 w281 w293 w305 w318 w329 w339 w347 w355 w362 w371] -> w204
              tunnel: [FALSE w213 w221 w234 w246 w258 w270 w282 w294 w306 w317 w328 w340 w348 w356 w363 w372] -> w205
              tunnel: w207 -> [_ w211 w223 w236 w248 w260 w272 w284 w296 w308 _ w325 _ _ _ _ _]
              tunnel: [_ w211 w222 w235 w247 w259 w271 w283 w295 w307 _ _ _ _ _ _ _] -> _
              tunnel: w203 -> [w208 w210 w219 w232 w244 w256 w268 w280 w292 w304 w315 w323 w337 w345 w354 w361 w370]
              event Timeout {
                n101 = event-data() -> ()  [unwired: 1 in, 3 out]
              }
              event "stop": Value Change {
                n102 = event-data() -> ()  [unwired: 1 in, 6 out]
                n103 = case shown="False" "stop" {
                  tunnel: [w215 w217] -> w214
                  tunnel: [FALSE TRUE] -> w213
                  tunnel: w210 -> [w215 _]
                  frame False {
                  }
                  frame True {
                    w217 = Action_Control_1."Exit"  # Event
                  }
                }
              }
              event "Record DAQ Raw Voltages": Value Change {
                n104 = event-data() -> ()  [unwired: 1 in, 6 out]
                n105 = case shown="False" "Record DAQ Raw Voltages" {
                  tunnel: [w225 w228] -> w220
                  tunnel: [FALSE FALSE ("Boolean")] -> w221
                  tunnel: [w226 w229] -> w222
                  tunnel: w223 -> [w226 w229]
                  tunnel: w219 -> [w225 _]
                  frame False {
                  }
                  frame True {
                    w228 = Action_Control_1."Acq. DAQ data"  # Event
                  }
                }
              }
              event "Record pH Calibration Zero": Value Change {
                n106 = event-data() -> ()  [unwired: 1 in, 6 out]
                n107 = case shown="True" "Record pH Calibration Zero" {
                  tunnel: [w237 w240] -> w233
                  tunnel: [FALSE FALSE ("Boolean")] -> w234
                  tunnel: [w238 w241] -> w235
                  tunnel: w236 -> [w238 w241]
                  tunnel: w232 -> [w237 _]
                  frame False {
                  }
                  frame True {
                    w240 = Action_Control_1."pH Calibration Zero"  # Event
                  }
                }
              }
              event "Record pH Calibration Reference": Value Change {
                n108 = event-data() -> ()  [unwired: 1 in, 6 out]
                n109 = case shown="True" "Record pH Calibration Reference" {
                  tunnel: [w249 w252] -> w245
                  tunnel: [FALSE FALSE ("Boolean")] -> w246
                  tunnel: [w250 w253] -> w247
                  tunnel: w248 -> [w250 w253]
                  tunnel: w244 -> [w249 _]
                  frame False {
                  }
                  frame True {
                    w252 = Action_Control_1."pH Calibration Standard"  # Event
                  }
                }
              }
              event "Record ORP Calibration": Value Change {
                n110 = event-data() -> ()  [unwired: 1 in, 6 out]
                n111 = case shown="True" "Record ORP Calibration" {
                  tunnel: [w261 w264] -> w257
                  tunnel: [FALSE FALSE ("Boolean")] -> w258
                  tunnel: [w262 w265] -> w259
                  tunnel: w260 -> [w262 w265]
                  tunnel: w256 -> [w261 _]
                  frame False {
                  }
                  frame True {
                    w264 = Action_Control_1."ORP Calibration Standard"  # Event
                  }
                }
              }
              event "Record Salinity Calibration": Value Change {
                n112 = event-data() -> ()  [unwired: 1 in, 6 out]
                n113 = case shown="True" "Record Salinity Calibration" {
                  tunnel: [w273 w276] -> w269
                  tunnel: [FALSE FALSE ("Boolean")] -> w270
                  tunnel: [w274 w277] -> w271
                  tunnel: w272 -> [w274 w277]
                  tunnel: w268 -> [w273 _]
                  frame False {
                  }
                  frame True {
                    w276 = Action_Control_1."Salinity Calibration Standard"  # Event
                  }
                }
              }
              event "Record DO Calibration": Value Change {
                n114 = event-data() -> ()  [unwired: 1 in, 6 out]
                n115 = case shown="True" "Record DO Calibration" {
                  tunnel: [w285 w288] -> w281
                  tunnel: [FALSE FALSE ("Boolean")] -> w282
                  tunnel: [w286 w289] -> w283
                  tunnel: w284 -> [w286 w289]
                  tunnel: w280 -> [w285 _]
                  frame False {
                  }
                  frame True {
                    w288 = Action_Control_1."DO Calibration Standard"  # Event
                  }
                }
              }
              event "Record  SC Calibration": Value Change {
                n116 = event-data() -> ()  [unwired: 1 in, 6 out]
                n117 = case shown="True" "Record  SC Calibration" {
                  tunnel: [w297 w300] -> w293
                  tunnel: [FALSE FALSE ("Boolean")] -> w294
                  tunnel: [w298 w301] -> w295
                  tunnel: w296 -> [w298 w301]
                  tunnel: w292 -> [w297 _]
                  frame False {
                  }
                  frame True {
                    w300 = Action_Control_1."SC Calibration Standard"  # Event
                  }
                }
              }
              event "Increment Depth": Value Change {
                n118 = event-data() -> ()  [unwired: 1 in, 6 out]
                n119 = case shown="True" "Increment Depth" {
                  tunnel: [w309 w312] -> w305
                  tunnel: [FALSE FALSE ("Boolean")] -> w306
                  tunnel: [w310 w313] -> w307
                  tunnel: w308 -> [w310 w313]
                  tunnel: w304 -> [w309 _]
                  frame False {
                  }
                  frame True {
                    w312 = Action_Control_1."Increment Depth Manually"  # Event
                  }
                }
              }
              event "Record Single Sample": Value Change {
                n120 = event-data() -> ("NewVal"=w316:bool)  [unwired: 1 in, 5 out]
                n121 = case shown="False" w316 {
                  tunnel: [w319 w321] -> w318
                  tunnel: [FALSE FALSE] -> w317
                  tunnel: w315 -> [w319 _]
                  frame False {
                  }
                  frame True {
                    w321 = Action_Control_1."Acq. Single Sonde Point"  # Event
                  }
                }
              }
              event "Write Data to Spreadsheet": Value Change {
                n122 = event-data() -> ("OldVal"=w327:bool, "NewVal"=w330:bool)  [unwired: 1 in, 4 out]
                n123 = Not(x=w327) -> (.not. x?=w326:bool)
                n124 = And(x=w326, y=w330) -> (x .and. y?=w324:bool)
                n125 = case shown="True" w324 {
                  tunnel: [w331 w334] -> w329
                  tunnel: [FALSE FALSE ("Boolean")] -> w328
                  tunnel: [w332 w335] -> _
                  tunnel: w325 -> [w332 w335]
                  tunnel: w323 -> [w331 _]
                  frame False {
                  }
                  frame True {
                    w334 = Action_Control_1."Write Sonde Sample Sheet"  # Event
                  }
                }
              }
              event "Sample Not Collected": Value Change {
                n126 = event-data() -> ("NewVal"=w338:bool)  [unwired: 1 in, 5 out]
                n127 = case shown="True" w338 {
                  tunnel: [FALSE FALSE] -> w340
                  tunnel: [w341 w343] -> w339
                  tunnel: w337 -> [_ w343]
                  frame True {
                    w341 = Action_Control_1."Sample Not Collected"  # Event
                  }
                  frame False {
                  }
                }
              }
              event "Record Reason": Value Change {
                n128 = event-data() -> ("NewVal"=w346:bool)  [unwired: 1 in, 5 out]
                n129 = case shown="True" w346 {
                  tunnel: [FALSE FALSE] -> w348
                  tunnel: [w349 w351] -> w347
                  tunnel: w345 -> [_ w351]
                  frame True {
                    w349 = Action_Control_1."Record Reason"  # Event
                  }
                  frame False {
                  }
                }
              }
              event "Start KPRO": Value Change {
                n130 = event-data() -> ()  [unwired: 1 in, 6 out]
                n131 = case shown="True" "Start KPRO" {
                  tunnel: [FALSE FALSE] -> w356
                  tunnel: [w357 w359] -> w355
                  tunnel: w354 -> [_ w359]
                  frame True {
                    w357 = Action_Control_1."Start KPRO Measurements"  # Event
                  }
                  frame False {
                  }
                }
              }
              event "Update Depth": Value Change {
                n132 = event-data() -> ()  [unwired: 1 in, 6 out]
                n133 = case shown="False" "Update Depth" {
                  tunnel: [FALSE FALSE] -> w363
                  tunnel: [w365 w367] -> w362
                  tunnel: w361 -> [_ w367]
                  frame True {
                    w365 = Action_Control_1."Update Depth"  # Event
                  }
                  frame False {
                  }
                }
              }
              event "Finish Tests": Value Change {
                n134 = event-data() -> ()  [unwired: 1 in, 6 out]
                n135 = case shown="True" "Finish Tests" {
                  tunnel: [FALSE FALSE] -> w372
                  tunnel: [w374 w376] -> w371
                  tunnel: w370 -> [_ w376]
                  frame True {
                    w374 = Action_Control_1."Finish KPRO Measurements"  # Event
                    "KPRO Finish\nIndicator" <- TRUE ("KPRO Finish\nIndicator")
                  }
                  frame False {
                  }
                }
              }
            }
          }
          frame True {
          }
        }
        "Stop" <- w198
        n136 = local read "Stop"() -> (w199:bool)
        n137 = Or(x=w199, y=w198) -> ()  [unwired: 1 out]
        n138 = call <extravilib>:"Write With Abort.vi"("abort"=FALSE, "last element? (F)"=w198, "element"=w196) -> ("channel"=w202:T24)  [unwired: 6 in, 2 out]
        "producer loop" <- w200
      }
    }
  }
  n139 = flat-sequence {
    tunnel: [w402] -> w18
    tunnel: w15 -> [w401]
    tunnel: w14 -> [w400]
    tunnel: w13 -> [w398]
    tunnel: w12 -> [w396]
    tunnel: w11 -> [w395]
    tunnel: w10 -> [w393]
    tunnel: w7 -> [w392]
    tunnel: w6 -> [w391]
    tunnel: w4 -> [w390]
    tunnel: w3 -> [w388]
    tunnel: w2 -> [w387]
    tunnel: w1 -> [w386]
    frame #0 {
      w380 = T3 {"SC Initial "=0.0, "DO Initial "=0.0, "pH Initial  "=0.0, "ORP  Initial"=0.0, "Temp Initial"=0.0, "Salinity Initial "=0.0}  # Sonde Parameters  Initial Values
      w381 = FALSE  # Read String Pot
      w382 = T15 {"Flow"=0.21081600494384767, "Zeroed \nPressure"=74.74207969932556, "Ik"=0.003788962123473114, "Current Depth"=-100.6, "Feet of Stainless"=40, "Start Depth"=0.0, "Abs Start Depth"=0.0}  # Input Depths  and Parameters Cluster
      w383 = T17 {"Absolute Depth In"=0.0, "Current Absolute Depth"=0.0, "First Absolute Depth"=0.0, "Previous Relative Depth"=0.0, "Current Relative Depth"=0.0, "First Relative Depth"=0.0, "Last Filed Depth"=0.0, "Total Volume In"=0.0, "Total Volume Out"=0.0, "Current Measurement Time"=0.0, "Previous Measurement Time"=0.0}  # Depth Cluster
      w384 = dbl[][] []  # Cumulative Data From File
      n140 = while {
        tunnel: w401 -> [w450]
        tunnel: [w451] -> w402
        tunnel: w390 -> [w424]
        tunnel: w400 -> [w449]
        shift-right: [w437] -> _
        shift-left: "Current Sheet" -> [w443]
        tunnel: w398 -> [w439]
        tunnel: w396 -> [w447]
        tunnel: w395 -> [w446]
        shift-right: [w438] -> _
        shift-left: 0 ("row index") -> [w445]
        tunnel: [w444] -> _
        shift-right: [w442] -> _
        shift-left: cluster{"row":i32, "column":i32} {"row"=0, "column"=0} ("start of last occupied row") -> [w441]
        tunnel: w393 -> [w436]
        shift-right: [w430] -> _
        shift-left: dbl[] [] ("Time Array") -> [w431]
        shift-right: [w429] -> _
        shift-left: w384 -> [w428]
        tunnel: w392 -> [w427]
        tunnel: [w426] -> _
        tunnel: w391 -> [w410]
        shift-right: [w422] -> _
        shift-left: refnum<k24>[] [] -> [w409]
        tunnel: w388 -> [w420]
        shift-right: [w403] -> _
        shift-left: w387 -> [w405]
        shift-right: [w419] -> _
        shift-left: w386 -> [w419]
        shift-right: [w416] -> _
        shift-left: w381 -> [w415]
        shift-right: [w414] -> _
        shift-left: w383 -> [w413]
        shift-right: [w412] -> _
        shift-left: w382 -> [w411]
        shift-right: [w406] -> _
        shift-left: w380 -> [_]
        i -> [w407]
        stop <- w425 stop-if-true
        # "Consumer Data Handling Loop"
        n141 = flat-sequence {
          frame #0 {
            n142 = call "boolean debounce 2016.vi"() -> ()  [unwired: 1 in, 1 out]
          }
        }
        n143 = call <extravilib>:"Read With Abort.vi"("abort"=FALSE, "channel"=w424) -> ("last element?"=w423:bool, "element"=w433:T23)  [unwired: 5 in, 3 out]
        n144 = call "Wait (ms)__ogtk.vi"("error in (no error)"=w450, "milliseconds to wait"=u32 50) -> ("error out"=w435:errorcluster)  [unwired: 8 in, 1 out]
        n145 = feedback-in #1(w433) -> ()
        n146 = feedback #1() -> (w432:T23)  [unwired: 1 in]
        n147 = call "open select sample sheet.vi"("Number of Sample Sheets"=w436, "error in (no error)"=w435, "Worksheet Names"=w439, "Active Sample Sheet"=w443, "NI_report in"=w449) -> ("error out"=w418:errorcluster, "Current Sample Sheet"=w421:string, "NI_report out"=w448:refnum<class "NI_report.lvclass">)  [unwired: 3 in, 1 out]
        n148 = flat-sequence {
          tunnel: w421 -> [w472]
          tunnel: w420 -> [w467]
          tunnel: w418 -> [w466]
          tunnel: [w464] -> w417
          frame #0 {
            n149 = Get Date/Time In Seconds() -> (seconds since 1Jan1904=w468:timestamp)
            n150 = Subtract(x=w468, y=w467) -> (x-y=w469:dbl)
            n151 = local write "Current Time (s)"(w469) -> ()
            n152 = Scan From String(format string="Sample %d", input string=w472, error in=w466) -> (error out=w465:errorcluster, output 1=w470:i32)  [unwired: 2 in, 2 out]
            n153 = Format Into String(format string="Data from Sample Sheet %d from Excel File", error in=w465, w470) -> (resulting string=→"Table Label":string, error out=w464:errorcluster)  [unwired: 1 in]
            "Current Sample Sheet" <- w472
          }
        }
        n154 = disable-structure shown="Enabled" {
          disable-tunnel: w410 -> [w455 _]
          disable-tunnel: w409 -> [w454 w463]
          disable-tunnel: [w453 w463] -> w408
          disable-tunnel: w407 -> [w452 _]
          frame Enabled {
            n155 = case shown="1, Default" w452 {
              tunnel: w454 -> [w456 w462]
              tunnel: w455 -> [_ w461]
              tunnel: [w456 w459] -> w453
              frame 0 {
              }
              frame 1, Default {
                n156 = local read "Descriptions"() -> (w460:string[])
                n157 = call "Measure DAQ Voltages.vi"("error in (no error)"=w461, "Descriptions"=w460, "Array in"=w462) -> ("Raw Voltages"=w458:dbl[], "Array out"=w459:refnum<k24>[], "Sensor Cluster"=w457:T9)  [unwired: 6 in]
                n158 = local write "Sensor Voltage Cluster"(w457) -> ()
                n159 = local write "Raw Voltages"(w458) -> ()
              }
            }
          }
          frame Disabled {
          }
        }
        n160 = case shown="\"Record Reason\"" w433 {
          selector: w433 -> [_ _ _ _ _ _ _ _ _ _ _ _ _ _ _ _ w1774 _ _ _]
          tunnel: w417 -> [w495 w597 w628 w645 w662 w796 w978 w992 w1032 w1065 w1162 w1262 w1363 w1464 w1565 w1665 w1783 w1826 w2201 w2215]
          tunnel: [w495 w597 w628 w645 w657 w791 w978 w992 w1031 w1063 w1160 w1260 w1361 w1462 w1563 w1663 w1754 w1826 w2201 w2225] -> w451
          tunnel: w423 -> [_ _ _ _ _ _ _ _ _ _ _ _ _ _ _ _ _ _ _ _]
          tunnel: w448 -> [w494 w596 w627 w644 w680 w816 w977 w991 w1024 w1080 w1180 w1280 w1381 w1482 w1583 w1683 w1784 w1833 w2200 w2216]
          tunnel: [w493 w595 w626 w643 w679 w815 w976 w990 w1023 w1061 w1157 w1257 w1358 w1459 w1560 w1660 w1759 w1832 w2199 w2230] -> w438
          tunnel: w447 -> [_ _ _ _ _ _ _ _ _ w1075 w1175 w1275 w1376 w1477 w1578 w1678 _ _ _ _]
          tunnel: w446 -> [_ _ _ _ _ _ _ _ _ w1074 w1174 w1274 w1375 w1476 w1577 w1677 _ _ _ _]
          tunnel: w445 -> [w493 w595 w626 w643 w679 w815 w976 w990 w1023 w1039 w1158 w1258 w1359 w1460 w1561 w1661 w1747 w1832 w2199 w2230]
          tunnel: [w494 w596 w627 w644 w680 w816 w977 w991 w1024 w1066 w1163 w1263 w1364 w1465 w1566 w1666 w1779 w1833 w2200 w2231] -> w444
          tunnel: w443 -> [w492 w594 w625 w642 w666 w800 w975 w989 w1022 w1036 w1171 w1271 w1372 w1473 w1574 w1674 w1776 w1831 w2198 w2229]
          tunnel: [w492 w594 w625 w642 w666 w800 w975 w989 w1022 w1036 w1171 w1271 w1372 w1473 w1574 w1674 w1775 w1831 w2198 w2229] -> w437
          tunnel: [w491 w593 w624 w641 w678 w814 w974 w988 w1021 w1062 w1159 w1259 w1360 w1461 w1562 w1662 w1770 w1830 w2197 w2228] -> w442
          tunnel: w441 -> [w491 w593 w624 w641 w678 w814 w974 w988 w1021 _ _ _ _ _ _ _ w1771 w1830 w2197 w2228]
          tunnel: w439 -> [_ _ _ _ _ _ _ _ _ _ _ _ _ _ _ _ w1778 _ _ _]
          tunnel: w436 -> [_ _ _ _ _ _ _ _ _ _ _ _ _ _ _ _ w1777 _ _ _]
          tunnel: w432 -> [_ _ _ _ _ _ _ _ _ _ _ _ _ _ _ _ w1773 _ _ _]
          tunnel: w431 -> [w490 w592 w623 w640 w677 w813 w973 w987 w1020 w1060 w1156 w1256 w1357 w1458 w1559 w1659 w1758 w1829 w2196 w2227]
          tunnel: [w490 w592 w623 w640 w677 w813 w973 w987 w1020 w1059 w1155 w1255 w1356 w1457 w1558 w1658 w1758 w1829 w2196 w2227] -> w430
          tunnel: [w476 w582 w622 w639 w664 w798 w972 w986 w1019 w1058 w1154 w1254 w1355 w1456 w1557 w1657 w1757 w1818 w2195 w2226] -> w429
          tunnel: w428 -> [w476 w582 w622 w639 w671 w805 w972 w986 w1019 w1057 w1153 w1253 w1354 w1455 w1556 w1656 w1757 w1819 w2195 w2226]
          tunnel: w427 -> [_ _ _ _ _ _ _ _ _ w1056 w1152 w1252 w1353 w1454 w1555 w1655 _ _ _ _]
          tunnel: w408 -> [w484 w591 w621 w638 w674 w810 w971 w985 w1018 w1054 w1150 w1250 w1351 w1452 w1553 w1653 w1756 _ w2193 w2220]
          tunnel: [w489 w590 w620 w637 w651 w790 w970 w984 w1017 w1055 w1151 w1251 w1352 w1453 w1554 w1654 w1755 w1825 _ w2221] -> w426
          tunnel: w410 -> [w489 w590 w620 w637 w652 w790 w970 w984 w1017 w1055 w1151 w1251 w1352 w1453 w1554 w1654 w1755 w1827 w2192 w2224]
          tunnel: [_ _ _ _ _ _ _ _ _ _ _ _ _ _ _ _ _ FALSE ("aborted?") FALSE ("aborted?") w2223] -> w425
          tunnel: [w480 w591 w621 w638 w674 w810 w971 w985 w1018 w1054 w1150 w1250 w1351 w1452 w1553 w1653 w1756 w1816 w2191 w2220] -> w422
          tunnel: [w488 w589 w619 w636 w676 w812 w969 w983 w1016 w1052 w1148 w1248 w1349 w1450 w1551 w1651 w1753 "Read String Pot" w2190 w2219] -> w416
          tunnel: w415 -> [w488 w589 w619 w636 w676 w812 w969 w983 w1016 w1052 w1148 w1248 w1349 w1450 w1551 w1651 w1753 _ w2190 w2219]
          tunnel: [w478 w584 w614 w632 w668 w802 w968 w982 w1015 w1051 w1147 w1247 w1348 w1449 w1550 w1650 w1752 w1822 w2189 w2218] -> w414
          tunnel: w413 -> [w478 w585 w615 w632 w669 w803 w968 w982 w1015 w1051 w1147 w1247 w1348 w1449 w1550 w1650 w1752 _ w2189 w2218]
          tunnel: [w487 w588 w618 w635 w675 w811 w967 w981 w1014 w1050 w1146 w1246 w1347 w1448 w1549 w1649 w1751 w1821 w2188 w2217] -> w412
          tunnel: w411 -> [w487 w588 w618 w635 w675 w811 w967 w981 w1014 w1050 w1146 w1246 w1347 w1448 w1549 w1649 w1751 _ w2188 w2217]
          tunnel: [w486 w587 w617 w634 w663 w797 w966 w980 w1013 w1044 w1145 w1245 w1346 w1447 w1548 w1648 w1750 w1812 w2187 w2212] -> w406
          tunnel: "Sonde Parameters \nInitial Values" -> [w486 w587 w617 w634 w663 w797 w966 w980 w1013 w1043 w1145 w1245 w1346 w1447 w1548 w1648 w1750 w1812 w2187 w2212]
          tunnel: w405 -> [w485 w586 w616 w633 w661 w795 w965 w979 w1012 w1042 w1144 w1244 w1345 w1446 w1547 w1647 w1749 w1811 w2186 w2211]
          tunnel: [w485 w586 w616 w633 w660 w794 w965 w979 w1012 w1042 w1144 w1244 w1345 w1446 w1547 w1647 w1749 w1811 w2186 w2211] -> w403
          frame "TimeOut", Default {
            n161 = flat-sequence {
              tunnel: [w568] -> _
              tunnel: [w573] -> w475
              tunnel: [w581] -> _
              tunnel: [w580] -> _
              tunnel: w484 -> [w579]
              tunnel: [w578] -> _
              frame #0 {
                n162 = local read "Input Variables and Slopes"() -> (w570:T16)
                n163 = local read "Input Variables and Slopes"() -> (w575:T16)
                n164 = local read "Zero In-Line Pressure\n(F = leave as is)"() -> (w574:bool)
                n165 = Unbundle By Name(w575) -> ("DH Pressure Trans Slope"=w581:dbl, "DH Pressure Offset"=w580:dbl)
                n166 = local read "Sensor Voltage Cluster"() -> (w576:T9)
                n167 = local read "Descriptions"() -> (w577:string[])
                n168 = local read "Sensor  Real Measurements"() -> (w572:T6)
                n169 = global read "Kpro Globals.vi" "Current Depth"() -> (w568:sgl)
                n170 = call "DHT Pressure 2016.vi"("Sensor Cluster"=w576, "DHT Pressure Offset"=w580, "Array in"=w579, "DHT Pressure \nSlope"=w581, "Descriptions"=w577, "Zero Pressure\n(F = leave as is)"=w574) -> ("Array out"=w578:refnum<k24>[], "DHT Pressure"=w573:dbl, "Sensor Cluster 2"=w569:T9)  [unwired: 7 in]
                n171 = local write "Sensor Voltage Cluster"(w569) -> ()
                n172 = call "convert sensor voltage to real measurements.vi"("Input Variables and Slopes"=w570, "Sensor  Real Measurements in"=w572, "Sensor Cluster"=w569) -> ("Sensor  Real Measurements out"=w571:T9)  [unwired: 8 in]
                n173 = local write "Sensor  Real Measurements"(w571) -> ()
                n174 = local write "Down hole Pressure"(w573) -> ()
                n175 = Add(x=w573, y=w568) -> ()  [unwired: 1 out]
              }
            }
            n176 = flat-sequence {
              tunnel: w484 -> [w561]
              tunnel: [w557] -> w483
              tunnel: [w556] -> w482
              frame #0 {
                n177 = local read "Input Variables and Slopes"() -> (w564:T16)
                n178 = Unbundle By Name(w564) -> ("Up Hole Pressure Slope"=w563:dbl, "Up Hole  Pressure Offset"=w560:dbl)
                n179 = local write "Input Variables and Slopes"(w564) -> ()
                n180 = local read "Sensor Voltage Cluster"() -> (w566:T9)
                n181 = local read "Descriptions"() -> (w557:string[])
                n182 = local read "Corrected Pressure Cluster"() -> (w559:T20)
                n183 = call "up hole Pressure 2016.vi"("Sensor Cluster"=w566, "Pressure Offset"=w560, "Array in"=w561, "Pressure \nSlope"=w563, "Descriptions"=w557, "Zero Pressure\n(F = leave as is)"=TRUE) -> ("Array out"=w556:refnum<k24>[], "Uphole Pressure"=w565:dbl, "Sensor Cluster 2"=w562:T9)  [unwired: 7 in]
                n184 = Bundle By Name(cluster=w559, "Up hole Corrected Pressure"=w565) -> (w558:T20)
                n185 = local write "Sensor Voltage Cluster"(w562) -> ()
                n186 = local write "Corrected Pressure Cluster"(w558) -> ()
              }
            }
            n187 = flat-sequence {
              tunnel: w483 -> [w549]
              tunnel: w482 -> [w552]
              tunnel: [w548] -> w479
              tunnel: [w549] -> w481
              tunnel: [w545] -> w477
              tunnel: [w547] -> w480
              frame #0 {
                w553 = 0.0  # Offset
                n188 = local read "Input Variables and Slopes"() -> (w551:T16)
                n189 = local read "Input Depths \nand Parameters Cluster"() -> (w544:T15)
                n190 = Unbundle By Name(w551) -> ("Flow Slope"=w550:dbl)
                n191 = local read "Input Depths \nand Parameters Cluster"() -> (w555:T15)
                n192 = Unbundle By Name(w544) -> ("Feet of Stainless"=w543:i32)
                n193 = call "Flow 2016.vi"("Descriptions"=w549, "Array in"=w552, "Flow Slope"=w550, "Offset"=w553) -> ("Sensor Cluster"=w548:T9, "Flow (ml/min)"=w545:dbl, "Array out"=w547:refnum<k24>[])  [unwired: 4 in]
                n194 = local write "Sensor Voltage Cluster"(w548) -> ()
                n195 = call "pressure and IK2 2016.vi"("Ft. of SS"=w543, "flow"=w545) -> ("IK"=→"Large Depth IK Graph":dbl)  [unwired: 1 in, 1 out]
                n196 = Bundle By Name(cluster=w555, "Flow"=w545) -> (w554:T15)
                n197 = local write "Input Depths \nand Parameters Cluster"(w554) -> ()
              }
            }
            n198 = flat-sequence {
              tunnel: w481 -> [w531]
              tunnel: w476 -> [w501]
              tunnel: w479 -> [w530]
              tunnel: w478 -> [w507]
              tunnel: [w529] -> _
              tunnel: w477 -> [w528]
              tunnel: w480 -> [w519]
              tunnel: [w518] -> _
              tunnel: [w496] -> _
              tunnel: [w510] -> _
              tunnel: w475 -> [w498]
              frame #0 {
                n199 = Unbundle By Name(w507) -> ("Current Relative Depth"=w506:dbl)
                n200 = local read "Input Depths \nand Parameters Cluster"() -> (w523:T15)
                n201 = local read "Culmulative Graph Cluster"() -> (w517:T19)
                n202 = local read "Depth mode"() -> (w504:bool)
                n203 = local read "Input Variables and Slopes"() -> (w527:T16)
                n204 = local read "KPRO Finish\nIndicator"() -> (w500:bool)
                n205 = local read "KPRO Output File Path"() -> (w510:path)
                n206 = Unbundle By Name(w523) -> ("Feet of Stainless"=w525:i32, "Zeroed \nPressure"=w524:dbl)
                n207 = Unbundle By Name(w527) -> ("String Pot Slope"=w526:dbl)
                n208 = call "Kpro Read String Pot 2016.vi"("Read String Pot"=w504, "Feet of\nStainless to be\nUsed (Count) in"=w525, "Corrected Array in"=w501, "Flow"=w528, "Manual Depth In"=w506, "Finished In"=w500, "Depth Cluster in"=w507, "String Pot \nSlope in"=w526, "Sensor Cluster In in"=w530, "Descriptions"=w531, "Zeroed Pressure in"=w524, "Array in"=w519, "Downhole Pressure Sensor"=w498) -> ("Sensor Cluster 2"=w520:T9, "IK"=w497:dbl, "Array out"=w518:refnum<k24>[], "Generate Array Calc IK"=w503:bool, "Feet of\nStainless to be\nUsed (Count) out"=w521:i32, "Depth Cluster out"=w529:T17, "Corrected Array out"=w508:dbl[][])  [unwired: 6 in, 2 out]
                n209 = local write "Ik"(w497) -> ()
                n210 = local write "Sensor Voltage Cluster"(w520) -> ()
                n211 = Unbundle By Name(w529) -> ("Current Absolute Depth"=w505:dbl)
                n212 = And(x=w503, y=w504) -> (x .and. y?=w502:bool)
                n213 = Bundle By Name(cluster=w523, "Feet of Stainless"=w521) -> (w522:T15)
                n214 = local write "Input Depths \nand Parameters Cluster"(w522) -> ()
                n215 = flat-sequence {
                  tunnel: w505 -> [w536]
                  frame #0 {
                    n216 = global write "Kpro Globals.vi" "Current Depth"(w536) -> ()
                    n217 = local write "Current Depth"(w536) -> ()
                    n218 = Divide(x=w536, y=3.281) -> (x/y=w537:dbl)
                    n219 = local read "Sample Sheet Data Row Cluster 2"() -> (w541:T1)
                    n220 = local read "Corrected Pressure Cluster"() -> (w539:T20)
                    n221 = Unbundle By Name(w539) -> ("Up hole Corrected Pressure"=w538:dbl)
                    n222 = Bundle By Name(cluster=w541, "Depth"=w536, "Head\nPressure"=w538) -> (w540:T1)
                    n223 = local write "Sample Sheet Data Row Cluster 2"(w540) -> ()
                    n224 = local write "Current \nDepth (m)"(w537) -> ()
                  }
                }
                n225 = case shown="True" w502 {
                  tunnel: w501 -> [w532 w535]
                  tunnel: w508 -> [_ w533]
                  tunnel: [w532 w534] -> w496
                  frame False {
                  }
                  frame True {
                    n226 = Build Array (concatenate)(w535, w533) -> (w534:dbl[][])
                  }
                }
                n227 = call "Array to Plot 2016.vi"("Input Cumulative Array"=w496, "Input Real Time Array"=w508) -> ("Cumulative - Depth vs.Drive Rate"=w513:cluster{dbl[], dbl[]}, "Cumulative - Depth vs. Ik"=w515:cluster{dbl[], dbl[]}, "Real Time - Depth vs. Drive Rate"=w514:cluster{dbl[], dbl[]}, "Real Time - Depth vs. Ik"=w499:cluster{dbl[], dbl[]})  [unwired: 2 in, 2 out]
                n228 = Bundle By Name(cluster=w517, "Cumulative - Depth vs. Ik"=w515, "Real Time - Depth vs. lk"=w499, "Cumulative - Depth vs. Drive Rate"=w514, "Real Time - Depth vs. Drive Rate"=w513) -> (w516:T19)
                n229 = local write "Large Depth IK Graph Cluster"(w499) -> ()
                n230 = local write "Culmulative Graph Cluster"(w516) -> ()
                n231 = local read "Input Depths \nand Parameters Cluster"() -> (w512:T15)
                n232 = local write "Cumulative_data_from_file"(w496) -> ()
                n233 = Unbundle By Name(w512) -> ("Flow"=→"Flow":dbl, "Zeroed \nPressure"=→"Zeroed Pressure":dbl)
              }
            }
          }
          frame "Finish KPRO Measurements" {
            n234 = flat-sequence {
              tunnel: w585 -> [w613]
              tunnel: [w611] -> w583
              tunnel: [w607] -> w584
              tunnel: w582 -> [w604]
              frame #0 {
                n235 = local read "Input Depths \nand Parameters Cluster"() -> (w610:T15)
                n236 = Unbundle By Name(w610) -> ("Feet of Stainless"=w612:i32)
                n237 = local read "KPRO Output File Path"() -> (w605:path)
                n238 = call "Finished Collection Write File.vi"("Cluster in"=w613, "Corrected Array in"=w604, "Feet of\nStainless to be\nUsed (Count) in"=w612, "Output KPRO"=w605) -> ("Corrected Array out"=w611:dbl[][], "Depth to \nbe Used \n(Feet)"=w606:sgl, "Feet of\nStainless to be\nUsed (Count) out"=w608:i32)  [unwired: 5 in]
                n239 = Bundle By Name(cluster=w613, "Absolute Depth In"=w606) -> (w607:T17)
                n240 = Bundle By Name(cluster=w610, "Feet of Stainless"=w608) -> (w609:T15)
                n241 = local write "Input Depths \nand Parameters Cluster"(w609) -> ()
              }
            }
            n242 = flat-sequence {
              tunnel: w583 -> [w602]
              frame #0 {
                n243 = control-ref of="KPRO Output File Path"() -> (w600:refnum<vi>)
                n244 = call "write KPRO file.vi"("Corrected Array in"=w602, "Generate Array Calc IK"=TRUE, "Path in"=w600) -> ("paths ok"=w599:bool, "appended path"=w598:path)  [unwired: 7 in]
                n245 = case shown="True" w599 {
                  tunnel: w598 -> [_ w603]
                  frame False {
                  }
                  frame True {
                    n246 = local write "KPRO Output File Path"(w603) -> ()
                  }
                }
              }
            }
          }
          frame "Update Depth" {
            n247 = flat-sequence {
              tunnel: w615 -> [w631]
              tunnel: [w630] -> w614
              frame #0 {
                n248 = Bundle By Name(cluster=w631, "Current Absolute Depth"="New Depth") -> (w630:T17)
                n249 = local write "Current Depth"("New Depth") -> ()
                n250 = local write "Depth Cluster"(w630) -> ()
              }
            }
          }
          frame "IK vs Time" {
          }
          frame "Start KPRO Measurements" {
            n251 = flat-sequence {
              tunnel: w674 -> [w707]
              tunnel: [w706] -> w673
              tunnel: w659 -> [w705]
              tunnel: w658 -> [w704]
              tunnel: [w703] -> w657
              tunnel: [w693] -> w656
              frame #0 {
                n252 = control-ref of="Input Variables and Slopes"() -> (w699:refnum<vi>)
                n253 = control-ref of="Sensor Voltage Cluster"() -> (w697:refnum<vi>)
                n254 = control-ref of="Zero In-Line Pressure\n(F = leave as is)"() -> (w696:refnum<vi>)
                n255 = control-ref of="Output File Path"() -> (w700:refnum<vi>)
                n256 = control-ref of="Descriptions"() -> (w698:refnum<vi>)
                n257 = call "measure down hole pressure and save to csv file.vi"("Path in"=w700, "reference 3"=w698, "reference in"=w699, "reference 4"=w697, "reference 5"=w696, "Record DTW File"="Record DTW File", "error in (no error)"=w704, "Array in"=w707, "Input Variables and Slopes"=w705) -> ("DTW path 2"=→"DTW path 2":path, "Array out"=w706:refnum<k24>[], "In-Line Pressure"=w693:dbl, "error out"=w703:errorcluster)  [unwired: 3 in]
                "Down hole Pressure" <- w693
                n258 = local read "Corrected Pressure Cluster"() -> (w695:T20)
                n259 = Bundle By Name(cluster=w695, "Down hole Corrected Pressure"=w693) -> (w694:T20)
                n260 = local write "Corrected Pressure Cluster"(w694) -> ()
                n261 = property on="Large Depth IK Graph" class="WFChart (strict)"("History Data"=dbl[] []) -> ()  [unwired: 2 in, 2 out]
              }
            }
            n262 = flat-sequence {
              tunnel: w662 -> [w715]
              tunnel: [w714] -> w658
              tunnel: w661 -> [w713]
              tunnel: [w712] -> w660
              tunnel: [w708] -> w659
              frame #0 {
                n263 = local read "Input Variables and Slopes"() -> (w710:T16)
                n264 = Unbundle By Name(w710) -> ("Depth to Water Table"=w711:dbl)
                n265 = disable-structure shown="Enabled" {
                  disable-tunnel: w711 -> [w721 w722]
                  disable-tunnel: [w720 w722] -> w709
                  disable-tunnel: w715 -> [w719 w724]
                  disable-tunnel: [w718 w724] -> w714
                  disable-tunnel: w713 -> [w717 w723]
                  disable-tunnel: [w716 w723] -> w712
                  frame Enabled {
                    n266 = call "New Stainless Correction Pop Up 2016.vi"("error in (no error)"=w719, "New Feet\n of Stainless\n(Count)"=w717, "Depth to \nWater Table\nInput"=w721) -> ("error in (no error) 2"=w718:errorcluster, "Feet of\nStainless to be\nUsed (Count)"=w716:i32, "Depth to \nWater Table\nOutput"=w720:dbl)  [unwired: 6 in]
                  }
                  frame Disabled {
                  }
                }
                n267 = Bundle By Name(cluster=w710, "Depth to Water Table"=w709) -> (w708:T16)
              }
            }
            n268 = flat-sequence {
              tunnel: w673 -> [w782]
              tunnel: [w778] -> w655
              tunnel: [w777] -> w654
              frame #0 {
                n269 = local read "Input Variables and Slopes"() -> (w785:T16)
                n270 = Unbundle By Name(w785) -> ("Up Hole Pressure Slope"=w784:dbl, "Up Hole  Pressure Offset"=w781:dbl)
                n271 = local write "Input Variables and Slopes"(w785) -> ()
                n272 = local read "Sensor Voltage Cluster"() -> (w787:T9)
                n273 = local read "Descriptions"() -> (w778:string[])
                n274 = local read "Corrected Pressure Cluster"() -> (w780:T20)
                n275 = call "up hole Pressure 2016.vi"("Sensor Cluster"=w787, "Pressure Offset"=w781, "Array in"=w782, "Pressure \nSlope"=w784, "Descriptions"=w778, "Zero Pressure\n(F = leave as is)"=TRUE) -> ("Array out"=w777:refnum<k24>[], "Uphole Pressure"=w786:dbl, "Sensor Cluster 2"=w783:T9)  [unwired: 7 in]
                n276 = Bundle By Name(cluster=w780, "Up hole Corrected Pressure"=w786) -> (w779:T20)
                n277 = local write "Sensor Voltage Cluster"(w783) -> ()
                n278 = local write "Corrected Pressure Cluster"(w779) -> ()
              }
            }
            n279 = local read "Input Variables and Slopes"() -> (w650:T16)
            n280 = Unbundle By Name(w650) -> ("String Pot Slope"=w649:dbl)
            n281 = call "depth read from string pot 2016.vi"("Descriptions"=w655, "error in (no error)"=w652, "String Pot \nSlope"=w649, "Array in"=w654) -> ("Array out"=w653:refnum<k24>[], "Depth"=w647:dbl, "error out"=w651:errorcluster)  [unwired: 12 in, 1 out]
            n282 = flat-sequence {
              tunnel: w647 -> [w682]
              tunnel: [w681] -> w646
              frame #0 {
                w683 = 15  # Filter Size
                # "Functional Global in \nBoxcar Integrator\nInitialize filter array to \ncurrent string pot value"
                n283 = call "Boxcar filter2016.vi"("Initialize"=TRUE, "Filter Size"=w683, "Filter Input"=w682) -> ("Filter Output"=w681:dbl)
              }
            }
            n284 = flat-sequence {
              tunnel: [w685] -> w648
              frame #0 {
                n285 = Tick Count (ms)() -> (millisecond timer value=w687:u32)
                n286 = Divide(x=w687, y=u32 1000) -> (x/y=w685:dbl)
              }
            }
            n287 = flat-sequence {
              tunnel: [w689] -> _
              tunnel: w646 -> [w690]
              tunnel: w648 -> [w688]
              frame #0 {
                n288 = local read "Depth Cluster"() -> (w691:T17)
                n289 = Bundle By Name(cluster=w691, "Previous Relative Depth"=w690, "Current Relative Depth"=w690, "First Relative Depth"=w690, "Current Measurement Time"=w688, "Previous Measurement Time"=w688) -> (w689:T17)
                n290 = local write "Depth Cluster"(w689) -> ()
              }
            }
            n291 = flat-sequence {
              tunnel: w655 -> [w770]
              tunnel: w653 -> [w773]
              tunnel: [w768] -> w670
              tunnel: [w770] -> w672
              tunnel: [w769] -> w667
              tunnel: [w767] -> w665
              frame #0 {
                w774 = 0.0  # Offset
                n292 = local read "Input Variables and Slopes"() -> (w772:T16)
                n293 = Unbundle By Name(w772) -> ("Flow Slope"=w771:dbl)
                n294 = local read "Input Depths \nand Parameters Cluster"() -> (w776:T15)
                n295 = call "Flow 2016.vi"("Descriptions"=w770, "Array in"=w773, "Flow Slope"=w771, "Offset"=w774) -> ("Sensor Cluster"=w768:T9, "Flow (ml/min)"=w769:dbl, "Array out"=w767:refnum<k24>[])  [unwired: 4 in]
                n296 = local write "Sensor Voltage Cluster"(w768) -> ()
                n297 = Bundle By Name(cluster=w776, "Flow"=w769) -> (w775:T15)
                n298 = local write "Input Depths \nand Parameters Cluster"(w775) -> ()
              }
            }
            n299 = flat-sequence {
              tunnel: w672 -> [w756]
              tunnel: w671 -> [w731]
              tunnel: w670 -> [w755]
              tunnel: w669 -> [w754]
              tunnel: [w753] -> w668
              tunnel: w667 -> [w752]
              tunnel: w665 -> [w744]
              tunnel: [w743] -> _
              tunnel: [w735] -> w664
              tunnel: w656 -> [w729]
              frame #0 {
                n300 = local read "Culmulative Graph Cluster"() -> (w742:T19)
                n301 = local read "Input Depths \nand Parameters Cluster"() -> (w748:T15)
                n302 = local read "Input Variables and Slopes"() -> (w751:T16)
                n303 = local read "KPRO Finish\nIndicator"() -> (w730:bool)
                n304 = local read "Depth mode"() -> (w733:bool)
                n305 = Not(x=w733) -> ()  [unwired: 1 out]
                n306 = Unbundle By Name(w748) -> ("Feet of Stainless"=w732:i32, "Zeroed \nPressure"=w749:dbl)
                n307 = Unbundle By Name(w751) -> ("String Pot Slope"=w750:dbl)
                n308 = call "Kpro Read String Pot 2016.vi"("Read String Pot"=w733, "Feet of\nStainless to be\nUsed (Count) in"=w732, "Corrected Array in"=w731, "Flow"=w752, "Finished In"=w730, "Depth Cluster in"=w754, "String Pot \nSlope in"=w750, "Sensor Cluster In in"=w755, "Descriptions"=w756, "Zeroed Pressure in"=w749, "Array in"=w744, "Downhole Pressure Sensor"=w729) -> ("Sensor Cluster 2"=w745:T9, "Array out"=w743:refnum<k24>[], "Generate Array Calc IK"=w734:bool, "Feet of\nStainless to be\nUsed (Count) out"=w746:i32, "Depth Cluster out"=w753:T17, "Corrected Array out"=w736:dbl[][])  [unwired: 7 in, 3 out]
                n309 = local write "Sensor Voltage Cluster"(w745) -> ()
                n310 = Unbundle By Name(w753) -> ("Current Absolute Depth"=w739:dbl)
                n311 = Bundle By Name(cluster=w748, "Feet of Stainless"=w746) -> (w747:T15)
                n312 = call "Array to Plot 2016.vi"("Input Cumulative Array"=w736) -> ("Cumulative - Depth vs.Drive Rate"=w737:cluster{dbl[], dbl[]}, "Cumulative - Depth vs. Ik"=w740:cluster{dbl[], dbl[]}, "Real Time - Depth vs. Drive Rate"=w738:cluster{dbl[], dbl[]}, "Real Time - Depth vs. Ik"=w725:cluster{dbl[], dbl[]})  [unwired: 3 in, 2 out]
                n313 = Bundle By Name(cluster=w742, "Cumulative - Depth vs. Ik"=w740, "Real Time - Depth vs. lk"=w725, "Cumulative - Depth vs. Drive Rate"=w738, "Real Time - Depth vs. Drive Rate"=w737) -> (w741:T19)
                n314 = local write "Culmulative Graph Cluster"(w741) -> ()
                n315 = local write "Large Depth IK Graph Cluster"(w725) -> ()
                n316 = local write "Input Depths \nand Parameters Cluster"(w747) -> ()
                n317 = flat-sequence {
                  tunnel: w739 -> [w760]
                  frame #0 {
                    n318 = global write "Kpro Globals.vi" "Current Depth"(w760) -> ()
                    n319 = local write "Current Depth"(w760) -> ()
                    n320 = Divide(x=w760, y=3.281) -> (x/y=w761:dbl)
                    n321 = local read "Sample Sheet Data Row Cluster 2"() -> (w765:T1)
                    n322 = local read "Corrected Pressure Cluster"() -> (w763:T20)
                    n323 = Unbundle By Name(w763) -> ("Up hole Corrected Pressure"=w762:dbl)
                    n324 = Bundle By Name(cluster=w765, "Depth"=w760, "Head\nPressure"=w762) -> (w764:T1)
                    n325 = local write "Sample Sheet Data Row Cluster 2"(w764) -> ()
                    n326 = local write "Current \nDepth (m)"(w761) -> ()
                  }
                }
                n327 = case shown="False" w734 {
                  tunnel: w736 -> [w758 w759]
                  tunnel: [w758 w759] -> w735
                  frame False {
                  }
                  frame True {
                  }
                }
                n328 = control-ref of="KPRO Output File Path"() -> (w728:refnum<vi>)
                n329 = call "write KPRO file.vi"("Corrected Array in"=w736, "Generate Array Calc IK"=w734, "Path in"=w728) -> ("paths ok"=w726:bool, "appended path"=w727:path)  [unwired: 7 in]
                n330 = case shown="True" w726 {
                  tunnel: w727 -> [_ w757]
                  frame False {
                  }
                  frame True {
                    "IKMGS appended path" <- w757
                  }
                }
              }
            }
          }
          frame "Increment Depth Manually" {
            n331 = disable-structure shown="Enabled" {
              disable-tunnel: w796 -> [w821 w839]
              disable-tunnel: w795 -> [w820 _]
              disable-tunnel: [w819 _] -> w794
              disable-tunnel: [w818 w840] -> w793
              disable-tunnel: [w817 w839] -> w792
              frame Disabled {
                n332 = flat-sequence {
                  tunnel: w821 -> [w829]
                  tunnel: [w828] -> w817
                  tunnel: w820 -> [w827]
                  tunnel: [w826] -> w819
                  tunnel: [w822] -> w818
                  frame #0 {
                    n333 = local read "Input Variables and Slopes"() -> (w824:T16)
                    n334 = Unbundle By Name(w824) -> ("Depth to Water Table"=w825:dbl)
                    n335 = disable-structure shown="Enabled" {
                      disable-tunnel: w825 -> [w835 w836]
                      disable-tunnel: [w834 w836] -> w823
                      disable-tunnel: w829 -> [w833 w838]
                      disable-tunnel: [w832 w838] -> w828
                      disable-tunnel: w827 -> [w831 w837]
                      disable-tunnel: [w830 w837] -> w826
                      frame Enabled {
                        n336 = call "New Stainless Correction Pop Up 2016.vi"("error in (no error)"=w833, "New Feet\n of Stainless\n(Count)"=w831, "Depth to \nWater Table\nInput"=w835) -> ("error in (no error) 2"=w832:errorcluster, "Feet of\nStainless to be\nUsed (Count)"=w830:i32, "Depth to \nWater Table\nOutput"=w834:dbl)  [unwired: 6 in]
                      }
                      frame Disabled {
                      }
                    }
                    n337 = Bundle By Name(cluster=w824, "Depth to Water Table"=w823) -> (w822:T16)
                  }
                }
              }
              frame Enabled {
                n338 = local read "Input Variables and Slopes"() -> (w840:T16)
              }
            }
            n339 = flat-sequence {
              tunnel: w810 -> [w928]
              tunnel: [w927] -> w809
              tunnel: w793 -> [w926]
              tunnel: w792 -> [w925]
              tunnel: [w924] -> w791
              tunnel: [w920] -> w789
              frame #0 {
                n340 = flat-sequence {
                  tunnel: [w945] -> w933
                  tunnel: [w934] -> w932
                  tunnel: [w944] -> w931
                  tunnel: [w943] -> w930
                  tunnel: [w942] -> w929
                  tunnel: w928 -> [w941]
                  tunnel: [w940] -> w927
                  tunnel: w926 -> [w936]
                  tunnel: [w934] -> w920
                  frame #0 {
                    n341 = local read "Zero In-Line Pressure\n(F = leave as is)"() -> (w935:bool)
                    n342 = Unbundle By Name(w936) -> ("DH Pressure Trans Slope"=w943:dbl, "DH Pressure Offset"=w942:dbl)
                    n343 = local read "Sensor Voltage Cluster"() -> (w938:T9)
                    n344 = local write "Input Variables and Slopes"(w936) -> ()
                    n345 = local read "Descriptions"() -> (w939:string[])
                    n346 = global read "Kpro Globals.vi" "Current Depth"() -> (w945:sgl)
                    n347 = call "DHT Pressure 2016.vi"("Sensor Cluster"=w938, "DHT Pressure Offset"=w942, "Array in"=w941, "DHT Pressure \nSlope"=w943, "Descriptions"=w939, "Zero Pressure\n(F = leave as is)"=w935) -> ("Array out"=w940:refnum<k24>[], "DHT Pressure"=w944:dbl, "Sensor Cluster 2"=w937:T9)  [unwired: 7 in]
                    n348 = local write "Sensor Voltage Cluster"(w937) -> ()
                    n349 = Add(x=w944, y=w945) -> (x+y=w934:dbl)
                    n350 = local write "Down hole Pressure"(w934) -> ()
                  }
                }
                n351 = local read "Record DTW File"() -> (w923:bool)
                n352 = case shown="True" w923 {
                  selector: w923 -> [w947 _]
                  tunnel: [w947 FALSE ("Boolean")] -> _
                  tunnel: w932 -> [_ w959]
                  tunnel: w933 -> [_ w960]
                  tunnel: w929 -> [_ w957]
                  tunnel: w931 -> [_ w958]
                  tunnel: w930 -> [_ w956]
                  tunnel: w925 -> [w946 w951]
                  tunnel: [w946 w950] -> w924
                  frame False {
                  }
                  frame True {
                    n353 = Build Array(w960, w959, w958, w957, w956) -> (w963:dbl[])
                    n354 = local read "Output File Path"() -> (w955:path)
                    n355 = call-poly "Strip Path__ogtk.vi"("path"=w955) -> ("stripped path"=w954:path)  [unwired: 1 out]
                    n356 = call-poly "Strip Path__ogtk.vi"("path"=path "DTW.csv") -> ("name"=w952:string)  [unwired: 1 out]
                    n357 = call-poly "Build Path__ogtk.vi"("name or relative path"=w952, "base path"=w954) -> ("appended path"=w948:path)
                    n358 = local write "DTW path 2"(w948) -> ()
                    n359 = call-poly <vilib>:"Write Delimited Spreadsheet.vi"("file path (dialog if empty)"=w948, "1D data"=w963, "append to file? (new file:F)"=TRUE, "error in (no error)"=w951, "delimiter (\\t)"="," ("delimiter (\\t)")) -> ("error out"=w950:errorcluster)  [unwired: 9 in, 1 out]
                  }
                }
                n360 = local read "Corrected Pressure Cluster"() -> (w921:T20)
                n361 = Bundle By Name(cluster=w921, "Down hole Corrected Pressure"=w920) -> (w922:T20)
                n362 = local write "Corrected Pressure Cluster"(w922) -> ()
              }
            }
            n363 = flat-sequence {
              tunnel: w809 -> [w913]
              tunnel: [w909] -> w808
              tunnel: [w908] -> w807
              frame #0 {
                n364 = local read "Input Variables and Slopes"() -> (w916:T16)
                n365 = Unbundle By Name(w916) -> ("Up Hole Pressure Slope"=w915:dbl, "Up Hole  Pressure Offset"=w912:dbl)
                n366 = local write "Input Variables and Slopes"(w916) -> ()
                n367 = local read "Sensor Voltage Cluster"() -> (w918:T9)
                n368 = local read "Descriptions"() -> (w909:string[])
                n369 = local read "Corrected Pressure Cluster"() -> (w911:T20)
                n370 = call "up hole Pressure 2016.vi"("Sensor Cluster"=w918, "Pressure Offset"=w912, "Array in"=w913, "Pressure \nSlope"=w915, "Descriptions"=w909, "Zero Pressure\n(F = leave as is)"=TRUE) -> ("Array out"=w908:refnum<k24>[], "Uphole Pressure"=w917:dbl, "Sensor Cluster 2"=w914:T9)  [unwired: 7 in]
                n371 = Bundle By Name(cluster=w911, "Up hole Corrected Pressure"=w917) -> (w910:T20)
                n372 = local write "Sensor Voltage Cluster"(w914) -> ()
                n373 = local write "Corrected Pressure Cluster"(w910) -> ()
              }
            }
            n374 = flat-sequence {
              tunnel: w808 -> [w901]
              tunnel: w807 -> [w904]
              tunnel: [w899] -> w804
              tunnel: [w901] -> w806
              tunnel: [w900] -> w801
              tunnel: [w898] -> w799
              frame #0 {
                w905 = 0.0  # Offset
                n375 = local read "Input Variables and Slopes"() -> (w903:T16)
                n376 = Unbundle By Name(w903) -> ("Flow Slope"=w902:dbl)
                n377 = local read "Input Depths \nand Parameters Cluster"() -> (w907:T15)
                n378 = call "Flow 2016.vi"("Descriptions"=w901, "Array in"=w904, "Flow Slope"=w902, "Offset"=w905) -> ("Sensor Cluster"=w899:T9, "Flow (ml/min)"=w900:dbl, "Array out"=w898:refnum<k24>[])  [unwired: 4 in]
                n379 = local write "Sensor Voltage Cluster"(w899) -> ()
                n380 = Bundle By Name(cluster=w907, "Flow"=w900) -> (w906:T15)
                n381 = local write "Input Depths \nand Parameters Cluster"(w906) -> ()
              }
            }
            n382 = flat-sequence {
              tunnel: w806 -> [w883]
              tunnel: w805 -> [w859]
              tunnel: w804 -> [w882]
              tunnel: w803 -> [w857]
              tunnel: [w881] -> w802
              tunnel: w801 -> [w880]
              tunnel: w799 -> [w871]
              tunnel: [w870] -> _
              tunnel: [w845] -> w798
              tunnel: w790 -> [w862]
              tunnel: w789 -> [w853]
              frame #0 {
                n383 = Unbundle By Name(w857) -> ("Current Relative Depth"=w854:dbl)
                n384 = local read "Input Depths \nand Parameters Cluster"() -> (w856:T15)
                n385 = Unbundle By Name(w856) -> ("Start Depth"=w855:sgl)
                n386 = global read "Kpro Globals.vi" "increment_amount"() -> (w860:dbl)
                n387 = local read "Culmulative Graph Cluster"() -> (w869:T19)
                n388 = local read "Input Depths \nand Parameters Cluster"() -> (w875:T15)
                n389 = Equal?(x=w854, y=w855) -> (x = y?=w846:bool)
                n390 = First Call?() -> (First Call?: T/F=w848:bool)
                n391 = And(x=w846, y=w848) -> (x .and. y?=w847:bool)
                n392 = local read "Input Variables and Slopes"() -> (w879:T16)
                n393 = local read "KPRO Finish\nIndicator"() -> (w858:bool)
                n394 = local read "Depth mode"() -> (w863:bool)
                n395 = case shown="True" w847 {
                  tunnel: w854 -> [w887 w888]
                  tunnel: [w886 w888] -> w861
                  tunnel: w860 -> [w885 _]
                  frame False {
                    n396 = Add(x=w885, y=w887) -> (x+y=w886:dbl)
                  }
                  frame True {
                  }
                }
                n397 = Unbundle By Name(w875) -> ("Feet of Stainless"=w877:i32, "Zeroed \nPressure"=w876:dbl)
                n398 = Unbundle By Name(w879) -> ("String Pot Slope"=w878:dbl)
                n399 = call "Kpro Read String Pot 2016.vi"("Read String Pot"=w863, "Feet of\nStainless to be\nUsed (Count) in"=w877, "Corrected Array in"=w859, "Flow"=w880, "Manual Depth In"=w861, "Finished In"=w858, "Depth Cluster in"=w857, "error in (no error)"=w862, "String Pot \nSlope in"=w878, "Sensor Cluster In in"=w882, "Descriptions"=w883, "Zeroed Pressure in"=w876, "Array in"=w871, "Downhole Pressure Sensor"=w853) -> ("Sensor Cluster 2"=w872:T9, "IK"=w842:dbl, "Array out"=w870:refnum<k24>[], "Generate Array Calc IK"=w851:bool, "Depth Rate"=→"Depth Rate\nft/min":dbl, "Feet of\nStainless to be\nUsed (Count) out"=w873:i32, "Depth Cluster out"=w881:T17, "Corrected Array out"=w852:dbl[][])  [unwired: 5 in, 1 out]
                n400 = local write "Sensor Voltage Cluster"(w872) -> ()
                n401 = Unbundle By Name(w881) -> ("Current Absolute Depth"=w866:dbl)
                n402 = Bundle By Name(cluster=w875, "Feet of Stainless"=w873) -> (w874:T15)
                n403 = call "Array to Plot 2016.vi"("Input Real Time Array"=w852) -> ("Cumulative - Depth vs.Drive Rate"=w864:cluster{dbl[], dbl[]}, "Cumulative - Depth vs. Ik"=w867:cluster{dbl[], dbl[]}, "Real Time - Depth vs. Drive Rate"=w865:cluster{dbl[], dbl[]}, "Real Time - Depth vs. Ik"=w843:cluster{dbl[], dbl[]})  [unwired: 3 in, 2 out]
                n404 = Bundle By Name(cluster=w869, "Cumulative - Depth vs. Ik"=w867, "Real Time - Depth vs. lk"=w843, "Cumulative - Depth vs. Drive Rate"=w865, "Real Time - Depth vs. Drive Rate"=w864) -> (w868:T19)
                n405 = local write "Culmulative Graph Cluster"(w868) -> ()
                n406 = local write "Large Depth IK Graph Cluster"(w843) -> ()
                n407 = local write "Ik"(w842) -> ()
                n408 = local write "Input Depths \nand Parameters Cluster"(w874) -> ()
                n409 = flat-sequence {
                  tunnel: w866 -> [w891]
                  frame #0 {
                    n410 = local read "Corrected Pressure Cluster"() -> (w894:T20)
                    n411 = global write "Kpro Globals.vi" "Current Depth"(w891) -> ()
                    n412 = local write "Current Depth"(w891) -> ()
                    n413 = Divide(x=w891, y=3.281) -> (x/y=w892:dbl)
                    n414 = local read "Sample Sheet Data Row Cluster 2"() -> (w896:T1)
                    n415 = local write "Current \nDepth (m)"(w892) -> ()
                    n416 = Unbundle By Name(w894) -> ("Up hole Corrected Pressure"=w893:dbl)
                    n417 = Bundle By Name(cluster=w896, "Depth"=w891, "Head\nPressure"=w893) -> (w895:T1)
                    n418 = local write "Sample Sheet Data Row Cluster 2"(w895) -> ()
                  }
                }
                n419 = case shown="False" w851 {
                  tunnel: w852 -> [w889 w890]
                  tunnel: [w889 w890] -> w845
                  frame False {
                  }
                  frame True {
                  }
                }
                n420 = control-ref of="KPRO Output File Path"() -> (w850:refnum<vi>)
                n421 = call "write KPRO file.vi"("Corrected Array in"=w852, "Generate Array Calc IK"=w851, "Path in"=w850) -> ("paths ok"=w844:bool, "appended path"=w849:path)  [unwired: 7 in]
                n422 = case shown="True" w844 {
                  tunnel: w849 -> [_ w884]
                  frame False {
                  }
                  frame True {
                    n423 = local write "KPRO Output File Path"(w884) -> ()
                  }
                }
                n424 = local write "Cumulative_data_from_file"(w845) -> ()
              }
            }
          }
          frame "Sample Not Collected" {
            n425 = local write "Tab Control"(T5."Recording Reason Sonde" ("Tab Control")) -> ()
          }
          frame "Record Reason" {
            n426 = flat-sequence {
              frame #0 {
                n427 = local read "Sample Sheet Data Row Cluster 2"() -> (w1011:T1)
                n428 = local write "Tab Control"(T5."Recording Reason Sonde" ("Tab Control")) -> ()
                n429 = local read "KPRO Output File Path"() -> (w1007:path)
                n430 = property on="Select Reasons to Record Data" class="Ring (strict)"() -> ("Strings []"=w998:string[])  [unwired: 2 in, 2 out]
                n431 = Get Date/Time In Seconds() -> (seconds since 1Jan1904=w1010:timestamp)
                n432 = Unbundle By Name(w1011) -> ("Head\nPressure"=w1009:dbl, "Depth"=w1008:dbl)
                n433 = call-poly "Strip Path Extension__ogtk.vi"("path"=w1007) -> ("root"=w1006:string)  [unwired: 1 out]
                n434 = call-poly "Convert File Extension__ogtk.vi"("new ending (none)"="_Sample failure.csv", "file name"=w1006) -> ("new filename"=w1004:string)  [unwired: 1 out]
                n435 = Index Array(array=w998, index="Select Reasons to Record Data") -> (element=w996:string)
                n436 = Format Date/Time String(seconds (now)=w1010) -> (date/time string=w1002:string)  [unwired: 2 in]
                n437 = Format Into String(w1009) -> (resulting string=w1001:string)  [unwired: 3 in, 1 out]
                n438 = Format Into String(w1008) -> (resulting string=w1000:string)  [unwired: 3 in, 1 out]
                n439 = Format Into String("Select Reasons to Record Data") -> (resulting string=w999:string)  [unwired: 3 in, 1 out]
                n440 = Build Array(w1002, w1001, w1000, w999, w996) -> (w995:string[])
                n441 = String To Path(string=w1004) -> (path=w1005:path)
                "Sonde Recording Failure Path" <- w1005
                n442 = call-poly <vilib>:"Write Delimited Spreadsheet.vi"("file path (dialog if empty)"=w1005, "1D data"=w995, "append to file? (new file:F)"=TRUE) -> ()  [unwired: 11 in, 2 out]
              }
            }
          }
          frame "Continuous  Sonde Data" {
            n443 = local read "Found Quanta Sonde Com Port"() -> (w1029:refnum<visa-resource-name>)
            n444 = control-ref of="Sonde Data Display"() -> (w1033:refnum<vi>)
            n445 = local read "Sample Sheet Data Row Cluster 2"() -> (w1025:T1)
            n446 = call "SDI-12 Continuous Operations.vi"("RS232 Port In"=w1029, "Sensor Address In"="0", "Sonde Data Ctl Refnum"=w1033, "Error In (No Error)"=w1032) -> ("output cluster"=w1030:T2, "Temperature"=w1027:cluster{"Y":dbl[], "Y":dbl[]}[], "Sonde Data Display"=w1026:T13, "Error Out"=w1031:errorcluster)  [unwired: 8 in, 4 out]
            n447 = Bundle By Name(cluster=w1025, "Sonde Data Cluster"=w1030) -> (w1028:T1)
            n448 = local write "Temperature"(w1027) -> ()
            n449 = local write "Sonde Data Display"(w1026) -> ()
            n450 = local write "Sample Sheet Data Row Cluster 2"(w1028) -> ()
          }
          frame "Acq. Single Sonde Point" {
            n451 = invoke on="Record Single Sample" class="Bool" method="Reinit To Default"(error in=w1065) -> (error out=w1064:errorcluster)  [unwired: 2 in, 2 out]
            n452 = call <vilib>:"Clear Errors.vi"("error in (no error)"=w1064) -> ("error out"=w1053:errorcluster)  [unwired: 5 in, 1 out]
            n453 = call "get sample sheet data cells.vi"("error in (no error)"=w1053, "NI_report in"=w1080) -> ("error out"=w1077:errorcluster, "data"=w1079:string[][], "NI_report out"=w1072:refnum<class "NI_report.lvclass">, "left edge output cluster"=w1078:cluster{"row":i32, "column":i32})  [unwired: 5 in, 1 out]
            n454 = flat-sequence {
              tunnel: w1077 -> [w1143]
              tunnel: [w1136] -> _
              tunnel: w1078 -> [w1141]
              tunnel: [w1140] -> w1076
              tunnel: [w1139] -> _
              tunnel: [w1138] -> w1071
              tunnel: w1079 -> [w1136]
              frame #0 {
                n455 = Array Subset(array=w1136, index (col)=2 ("index")) -> (w1132:string[][])  [unwired: 3 in]
                n456 = local write "subarray"(w1132) -> ()
                n457 = local read "Current Sample Sheet"() -> (w1135:string)
                n458 = call "find last occupied cell.vi"("data"=w1136, "Active Sheet"=w1135, "Header Rows to remove"=3, "sub array start"=w1141, "error in (no error)"=w1143) -> ("row max value"=w1139:i32, "column max value"=w1134:i32, 13:"start of last occupied row"=w1138:cluster{"row":i32, "column":i32}, 14:"start of last occupied row"=w1133:string, "error out"=w1140:errorcluster)  [unwired: 4 in, 2 out]
                n459 = local write "last occupied cell's name"(w1133) -> ()
                n460 = local write "row max value"(w1134) -> ()
              }
            }
            n461 = local read "Found Quanta Sonde Com Port"() -> (w1068:refnum<visa-resource-name>)
            n462 = Equal?(x=w1068, y=refnum<visa-resource-name> refnum ("RS232 Port Out")) -> (x = y?=w1070:bool)
            n463 = case shown="True" w1070 {
              tunnel: w1068 -> [w1111 _]
              tunnel: [w1102 w1128] -> w1049
              tunnel: w1076 -> [w1106 w1131]
              tunnel: [w1105 w1131] -> w1073
              tunnel: w1060 -> [w1101 w1130]
              tunnel: [w1100 w1119] -> w1059
              tunnel: [w1099 w1118] -> w1058
              tunnel: w1057 -> [w1098 w1129]
              tunnel: w1056 -> [_ w1115]
              tunnel: [w1096 w1112] -> w1038
              frame False {
                n464 = control-ref of="Sonde Data Display"() -> (w1107:refnum<vi>)
                n465 = local read "Sample Sheet Data Row Cluster 2"() -> (w1103:T1)
                n466 = call "SDI-12 Single Operation with output cluster.vi"("RS232 Port In"=w1111, "Sensor Address In"="0", "Sonde Data Ctl Refnum"=w1107, "Error In (No Error)"=w1106, "Time Array In"=w1101, "Measurement Array In"=w1098) -> ("time array out"=w1100:dbl[], "Time Array"=w1097:timestamp[], "Measurement  array Out"=w1099:dbl[][], "output cluster"=w1104:T2, "Temperature"=w1109:cluster{"Y":dbl[], "Y":dbl[]}[], "Sonde Data Display"=w1108:T13, "Error Out"=w1105:errorcluster)  [unwired: 12 in, 3 out]
                n467 = local write "Temperature"(w1109) -> ()
                n468 = local write "Sonde Data Display"(w1108) -> ()
                n469 = Bundle By Name(cluster=w1103, "Sonde Data Cluster"=w1104) -> (w1102:T1)
                n470 = Index Array(array=w1097) -> (element=w1096:timestamp)  [unwired: 1 in]
              }
              frame True {
                n471 = Get Date/Time In Seconds() -> (seconds since 1Jan1904=w1112:timestamp)
                n472 = To Double Precision Float(number=w1112) -> (double precision float=w1120:dbl)
                n473 = local read "Sample Sheet Data Row Cluster 2"() -> (w1128:T1)
                n474 = Subtract(x=w1120, y=w1115) -> (x-y=w1113:dbl)
                n475 = local write "Current Time (s)"(w1113) -> ()
                n476 = Unbundle By Name(w1128) -> ("Sonde Data Cluster.Temp"=w1114:dbl, "Sonde Data Cluster.pH"=w1127:dbl, "Sonde Data Cluster.Specific\nConductance"=w1126:dbl, "Sonde Data Cluster.Salinity"=w1125:dbl, "Sonde Data Cluster.Dissolved\nOxygen"=w1124:dbl, "Sonde Data Cluster.ORP"=w1123:dbl)  [unwired: 1 out]
                n477 = Build Array(w1114, w1127, w1126, w1125, w1124, 0.0 ("element"), w1123) -> (w1121:dbl[])
                n478 = Build Array (concatenate)(w1129, w1121) -> (w1118:dbl[][])
                n479 = Build Array (concatenate)(w1130, w1113) -> (w1119:dbl[])
                n480 = call "format into Sonde Vertical Graph Data Input.vi"("Sonde Measurement Array"=w1118, "Time Array"=w1119) -> ("Sonde Data Display"=w1117:T13, "Temperature"=w1116:cluster{"X":dbl[], "Y":dbl[]}[])  [unwired: 8 in]
                n481 = local write "Temperature"(w1116) -> ()
                n482 = local write "Sonde Data Display"(w1117) -> ()
              }
            }
            n483 = local write "Sample Sheet Data Row Cluster 2"(w1049) -> ()
            n484 = call "write out sonde row.vi"("NI_report in"=w1072, "Columns"=w1075, "Column of Volume"=w1074, "Sample Sheet Data Row Cluster"=w1049, "row index"=w1039, "error in (no error)"=w1073, "start of last occupied row"=w1071) -> ("NI_report out"=w1067:refnum<class "NI_report.lvclass">, "row index out"=w1061:i32, "error out"=w1048:errorcluster)  [unwired: 6 in]
            n485 = To Double Precision Float(number=w1038) -> (double precision float=w1037:dbl)
            n486 = call "populate sonde row cluster from sonde data cluster.vi"("Time Value"=w1037, "Initialize \nInitial Value \nCluster"=TRUE ("Initialize \nInitial Value \nCluster"), "error in (no error)"=w1048, "Sonde Parameters \nInitial Values"=w1043, "Sample Sheet Data Row Cluster"=w1049, "Sonde Parameters \nTolerance Limits"="Sonde Parameters \nTolerance Limits") -> ("error out"=w1047:errorcluster, "Cluster"=w1035:T11, "Sonde Parameters \nInitial Values Out"=w1044:T3)  [unwired: 3 in]
            n487 = local read "Sonde Data Array"() -> (w1041:T11[])
            n488 = Insert Into Array(array=w1041, index=w1039, new element=w1035) -> (w1040:T11[])
            n489 = local write "Sonde Data Array"(w1040) -> ()
            n490 = flat-sequence {
              tunnel: w1047 -> [w1095]
              tunnel: w1067 -> [w1094]
              tunnel: [w1093] -> w1066
              tunnel: [w1088] -> w1063
              tunnel: [w1086] -> w1062
              frame #0 {
                (unwired) 3 ("Header Rows to remove")
                n491 = call <vilib>:"Clear Errors.vi"("error in (no error)"=w1095) -> ("error out"=w1082:errorcluster)  [unwired: 5 in, 1 out]
                n492 = local read "Current Sample Sheet"() -> (w1084:string)
                n493 = call "get sample sheet data cells.vi"("error in (no error)"=w1082, "NI_report in"=w1094) -> ("error out"=w1089:errorcluster, "data"=w1090:string[][], "NI_report out"=w1093:refnum<class "NI_report.lvclass">, "left edge output cluster"=w1087:cluster{"row":i32, "column":i32})  [unwired: 5 in, 1 out]
                n494 = call "find last occupied cell.vi"("data"=w1090, "Active Sheet"=w1084, "Header Rows to remove"=3, "sub array start"=w1087, "error in (no error)"=w1089) -> ("row max value"=w1085:i32, 13:"start of last occupied row"=w1086:cluster{"row":i32, "column":i32}, 14:"start of last occupied row"=w1083:string, "error out"=w1088:errorcluster)  [unwired: 4 in, 3 out]
                n495 = Array Subset(array=w1090, index (col)=2 ("index")) -> (w1081:string[][])  [unwired: 3 in]
                n496 = local write "row max value"(w1085) -> ()
                n497 = local write "last occupied cell's name"(w1083) -> ()
                n498 = local write "subarray"(w1081) -> ()
              }
            }
          }
          frame "pH Calibration Zero" {
            n499 = invoke on="Record Single Sample" class="Bool" method="Reinit To Default"(error in=w1162) -> (error out=w1161:errorcluster)  [unwired: 2 in, 2 out]
            n500 = call <vilib>:"Clear Errors.vi"("error in (no error)"=w1161) -> ("error out"=w1149:errorcluster)  [unwired: 5 in, 1 out]
            n501 = call "get sample sheet data cells.vi"("error in (no error)"=w1149, "NI_report in"=w1180) -> ("error out"=w1177:errorcluster, "data"=w1179:string[][], "NI_report out"=w1172:refnum<class "NI_report.lvclass">, "left edge output cluster"=w1178:cluster{"row":i32, "column":i32})  [unwired: 5 in, 1 out]
            n502 = flat-sequence {
              tunnel: w1177 -> [w1243]
              tunnel: [w1236] -> _
              tunnel: w1178 -> [w1241]
              tunnel: [w1240] -> w1176
              tunnel: [w1239] -> _
              tunnel: [w1238] -> w1170
              tunnel: w1179 -> [w1236]
              frame #0 {
                n503 = Array Subset(array=w1236, index (col)=2 ("index")) -> ()  [unwired: 3 in, 1 out]
                n504 = local read "Current Sample Sheet"() -> (w1235:string)
                n505 = call "find last occupied cell.vi"("data"=w1236, "Active Sheet"=w1235, "Header Rows to remove"=3, "sub array start"=w1241, "error in (no error)"=w1243) -> ("row max value"=w1239:i32, "column max value"=w1234:i32, 13:"start of last occupied row"=w1238:cluster{"row":i32, "column":i32}, 14:"start of last occupied row"=w1233:string, "error out"=w1240:errorcluster)  [unwired: 4 in, 2 out]
                n506 = local write "last occupied cell's name"(w1233) -> ()
                n507 = local write "row max value"(w1234) -> ()
              }
            }
            n508 = local read "Found Quanta Sonde Com Port"() -> (w1166:refnum<visa-resource-name>)
            n509 = Equal?(x=w1166, y=refnum<visa-resource-name> refnum ("RS232 Port Out")) -> (x = y?=w1168:bool)
            n510 = case shown="True" w1168 {
              tunnel: w1166 -> [w1198 _]
              tunnel: [w1206 w1229] -> w1169
              tunnel: w1176 -> [w1200 w1232]
              tunnel: [w1209 w1232] -> w1173
              tunnel: w1156 -> [w1205 w1231]
              tunnel: [w1204 w1219] -> w1155
              tunnel: [w1203 w1218] -> w1154
              tunnel: w1153 -> [w1202 w1230]
              tunnel: w1152 -> [_ w1215]
              frame False {
                w1201 = "0" ("Sensor Address In")
                n511 = control-ref of="Sonde Data Display"() -> (w1210:refnum<vi>)
                n512 = local read "Sample Sheet Data Row Cluster 2"() -> (w1207:T1)
                n513 = call "Calibrate pH Sensor.vi"("Calibration Standard"="pH Zero", "Error In (No Error)"=w1200, "Sensor Address In"=w1201, "RS232 Port In"=w1198) -> ("Error Out"=w1199:errorcluster, "Sensor Calibrate Response"=→"pH Zero \nCalibrate Response":bool, "RS232 Port Out"=w1197:refnum<visa-resource-name>)  [unwired: 4 in, 1 out]
                n514 = call "SDI-12 Single Operation with output cluster.vi"("RS232 Port In"=w1197, "Sensor Address In"=w1201, "Sonde Data Ctl Refnum"=w1210, "Error In (No Error)"=w1199, "Time Array In"=w1205, "Measurement Array In"=w1202) -> ("time array out"=w1204:dbl[], "Measurement  array Out"=w1203:dbl[][], "output cluster"=w1208:T2, "Temperature"=w1212:cluster{"Y":dbl[], "Y":dbl[]}[], "Sonde Data Display"=w1211:T13, "Error Out"=w1209:errorcluster)  [unwired: 12 in, 4 out]
                n515 = local write "Temperature"(w1212) -> ()
                n516 = local write "Sonde Data Display"(w1211) -> ()
                n517 = Bundle By Name(cluster=w1207, "Sonde Data Cluster"=w1208) -> (w1206:T1)
              }
              frame True {
                n518 = Get Date/Time In Seconds() -> (seconds since 1Jan1904=w1221:timestamp)
                n519 = To Double Precision Float(number=w1221) -> (double precision float=w1220:dbl)
                n520 = local read "Sample Sheet Data Row Cluster 2"() -> (w1229:T1)
                n521 = Subtract(x=w1220, y=w1215) -> (x-y=w1213:dbl)
                n522 = local write "Current Time (s)"(w1213) -> ()
                n523 = Unbundle By Name(w1229) -> ("Sonde Data Cluster.Temp"=w1214:dbl, "Sonde Data Cluster.pH"=w1228:dbl, "Sonde Data Cluster.Specific\nConductance"=w1227:dbl, "Sonde Data Cluster.Salinity"=w1226:dbl, "Sonde Data Cluster.Dissolved\nOxygen"=w1225:dbl, "Sonde Data Cluster.ORP"=w1224:dbl)  [unwired: 1 out]
                n524 = Build Array(w1214, w1228, w1227, w1226, w1225, 0.0 ("element"), w1224) -> (w1222:dbl[])
                n525 = Build Array (concatenate)(w1230, w1222) -> (w1218:dbl[][])
                n526 = Build Array (concatenate)(w1231, w1213) -> (w1219:dbl[])
                n527 = call "format into Sonde Vertical Graph Data Input.vi"("Sonde Measurement Array"=w1218, "Time Array"=w1219) -> ("Sonde Data Display"=w1217:T13, "Temperature"=w1216:cluster{"X":dbl[], "Y":dbl[]}[])  [unwired: 8 in]
                n528 = local write "Temperature"(w1216) -> ()
                n529 = local write "Sonde Data Display"(w1217) -> ()
              }
            }
            n530 = local write "Sample Sheet Data Row Cluster 2"(w1169) -> ()
            n531 = call "write out sonde row.vi"("NI_report in"=w1172, "Columns"=w1175, "Column of Volume"=w1174, "Sample Sheet Data Row Cluster"=w1169, "row index"=w1158, "error in (no error)"=w1173, "start of last occupied row"=w1170) -> ("NI_report out"=w1164:refnum<class "NI_report.lvclass">, "row index out"=w1157:i32, "error out"=w1165:errorcluster)  [unwired: 6 in]
            n532 = flat-sequence {
              tunnel: w1165 -> [w1194]
              tunnel: w1164 -> [w1193]
              tunnel: [w1192] -> w1163
              tunnel: [w1187] -> w1160
              tunnel: [w1185] -> w1159
              frame #0 {
                (unwired) 3 ("Header Rows to remove")
                n533 = call <vilib>:"Clear Errors.vi"("error in (no error)"=w1194) -> ("error out"=w1181:errorcluster)  [unwired: 5 in, 1 out]
                n534 = local read "Current Sample Sheet"() -> (w1183:string)
                n535 = call "get sample sheet data cells.vi"("error in (no error)"=w1181, "NI_report in"=w1193) -> ("error out"=w1188:errorcluster, "data"=w1189:string[][], "NI_report out"=w1192:refnum<class "NI_report.lvclass">, "left edge output cluster"=w1186:cluster{"row":i32, "column":i32})  [unwired: 5 in, 1 out]
                n536 = call "find last occupied cell.vi"("data"=w1189, "Active Sheet"=w1183, "Header Rows to remove"=3, "sub array start"=w1186, "error in (no error)"=w1188) -> ("row max value"=w1184:i32, 13:"start of last occupied row"=w1185:cluster{"row":i32, "column":i32}, 14:"start of last occupied row"=w1182:string, "error out"=w1187:errorcluster)  [unwired: 4 in, 3 out]
                n537 = Array Subset(array=w1189, index (col)=2 ("index")) -> ()  [unwired: 3 in, 1 out]
                n538 = local write "row max value"(w1184) -> ()
                n539 = local write "last occupied cell's name"(w1182) -> ()
              }
            }
          }
          frame "pH Calibration Standard" {
            n540 = invoke on="Record Single Sample" class="Bool" method="Reinit To Default"(error in=w1262) -> (error out=w1261:errorcluster)  [unwired: 2 in, 2 out]
            n541 = call <vilib>:"Clear Errors.vi"("error in (no error)"=w1261) -> ("error out"=w1249:errorcluster)  [unwired: 5 in, 1 out]
            n542 = call "get sample sheet data cells.vi"("error in (no error)"=w1249, "NI_report in"=w1280) -> ("error out"=w1277:errorcluster, "data"=w1279:string[][], "NI_report out"=w1272:refnum<class "NI_report.lvclass">, "left edge output cluster"=w1278:cluster{"row":i32, "column":i32})  [unwired: 5 in, 1 out]
            n543 = flat-sequence {
              tunnel: w1277 -> [w1344]
              tunnel: [w1337] -> _
              tunnel: w1278 -> [w1342]
              tunnel: [w1341] -> w1276
              tunnel: [w1340] -> _
              tunnel: [w1339] -> w1270
              tunnel: w1279 -> [w1337]
              frame #0 {
                n544 = Array Subset(array=w1337, index (col)=2 ("index")) -> ()  [unwired: 3 in, 1 out]
                n545 = local read "Current Sample Sheet"() -> (w1336:string)
                n546 = call "find last occupied cell.vi"("data"=w1337, "Active Sheet"=w1336, "Header Rows to remove"=3, "sub array start"=w1342, "error in (no error)"=w1344) -> ("row max value"=w1340:i32, "column max value"=w1335:i32, 13:"start of last occupied row"=w1339:cluster{"row":i32, "column":i32}, 14:"start of last occupied row"=w1334:string, "error out"=w1341:errorcluster)  [unwired: 4 in, 2 out]
                n547 = local write "last occupied cell's name"(w1334) -> ()
                n548 = local write "row max value"(w1335) -> ()
              }
            }
            n549 = local read "Found Quanta Sonde Com Port"() -> (w1266:refnum<visa-resource-name>)
            n550 = Equal?(x=w1266, y=refnum<visa-resource-name> refnum ("RS232 Port Out")) -> (x = y?=w1268:bool)
            n551 = case shown="False" w1268 {
              tunnel: w1266 -> [w1296 _]
              tunnel: [w1306 w1330] -> w1269
              tunnel: w1276 -> [w1299 w1333]
              tunnel: [w1309 w1333] -> w1273
              tunnel: w1256 -> [w1305 w1332]
              tunnel: [w1304 w1320] -> w1255
              tunnel: [w1303 w1319] -> w1254
              tunnel: w1253 -> [w1302 w1331]
              tunnel: w1252 -> [_ w1316]
              frame False {
                n552 = control-ref of="Sonde Data Display"() -> (w1310:refnum<vi>)
                n553 = call "Calibrate pH Sensor.vi"("Calibration Standard"="pH Reference", "Error In (No Error)"=w1299, "Sensor Address In"="0", "RS232 Port In"=w1296) -> ("Error Out"=w1298:errorcluster, "Sensor Calibrate Response"=→"pH  Reference\nCalibrate Response":bool, "RS232 Port Out"=w1295:refnum<visa-resource-name>)  [unwired: 4 in, 1 out]
                n554 = local read "Sample Sheet Data Row Cluster 2"() -> (w1307:T1)
                n555 = call "SDI-12 Single Operation with output cluster.vi"("RS232 Port In"=w1295, "Sensor Address In"="0", "Sonde Data Ctl Refnum"=w1310, "Error In (No Error)"=w1298, "Time Array In"=w1305, "Measurement Array In"=w1302) -> ("time array out"=w1304:dbl[], "Measurement  array Out"=w1303:dbl[][], "output cluster"=w1308:T2, "Temperature"=w1312:cluster{"Y":dbl[], "Y":dbl[]}[], "Sonde Data Display"=w1311:T13, "Error Out"=w1309:errorcluster)  [unwired: 12 in, 4 out]
                n556 = Bundle By Name(cluster=w1307, "Sonde Data Cluster"=w1308) -> (w1306:T1)
                n557 = local write "Temperature"(w1312) -> ()
                n558 = local write "Sonde Data Display"(w1311) -> ()
              }
              frame True {
                n559 = Get Date/Time In Seconds() -> (seconds since 1Jan1904=w1322:timestamp)
                n560 = To Double Precision Float(number=w1322) -> (double precision float=w1321:dbl)
                n561 = local read "Sample Sheet Data Row Cluster 2"() -> (w1330:T1)
                n562 = Subtract(x=w1321, y=w1316) -> (x-y=w1314:dbl)
                n563 = local write "Current Time (s)"(w1314) -> ()
                n564 = Unbundle By Name(w1330) -> ("Sonde Data Cluster.Temp"=w1315:dbl, "Sonde Data Cluster.pH"=w1329:dbl, "Sonde Data Cluster.Specific\nConductance"=w1328:dbl, "Sonde Data Cluster.Salinity"=w1327:dbl, "Sonde Data Cluster.Dissolved\nOxygen"=w1326:dbl, "Sonde Data Cluster.ORP"=w1325:dbl)  [unwired: 1 out]
                n565 = Build Array(w1315, w1329, w1328, w1327, w1326, 0.0 ("element"), w1325) -> (w1323:dbl[])
                n566 = Build Array (concatenate)(w1331, w1323) -> (w1319:dbl[][])
                n567 = Build Array (concatenate)(w1332, w1314) -> (w1320:dbl[])
                n568 = call "format into Sonde Vertical Graph Data Input.vi"("Sonde Measurement Array"=w1319, "Time Array"=w1320) -> ("Sonde Data Display"=w1318:T13, "Temperature"=w1317:cluster{"X":dbl[], "Y":dbl[]}[])  [unwired: 8 in]
                n569 = local write "Temperature"(w1317) -> ()
                n570 = local write "Sonde Data Display"(w1318) -> ()
              }
            }
            n571 = local write "Sample Sheet Data Row Cluster 2"(w1269) -> ()
            n572 = call "write out sonde row.vi"("NI_report in"=w1272, "Columns"=w1275, "Column of Volume"=w1274, "Sample Sheet Data Row Cluster"=w1269, "row index"=w1258, "error in (no error)"=w1273, "start of last occupied row"=w1270) -> ("NI_report out"=w1264:refnum<class "NI_report.lvclass">, "row index out"=w1257:i32, "error out"=w1265:errorcluster)  [unwired: 6 in]
            n573 = flat-sequence {
              tunnel: w1265 -> [w1294]
              tunnel: w1264 -> [w1293]
              tunnel: [w1292] -> w1263
              tunnel: [w1287] -> w1260
              tunnel: [w1285] -> w1259
              frame #0 {
                (unwired) 3 ("Header Rows to remove")
                n574 = call <vilib>:"Clear Errors.vi"("error in (no error)"=w1294) -> ("error out"=w1281:errorcluster)  [unwired: 5 in, 1 out]
                n575 = local read "Current Sample Sheet"() -> (w1283:string)
                n576 = call "get sample sheet data cells.vi"("error in (no error)"=w1281, "NI_report in"=w1293) -> ("error out"=w1288:errorcluster, "data"=w1289:string[][], "NI_report out"=w1292:refnum<class "NI_report.lvclass">, "left edge output cluster"=w1286:cluster{"row":i32, "column":i32})  [unwired: 5 in, 1 out]
                n577 = call "find last occupied cell.vi"("data"=w1289, "Active Sheet"=w1283, "Header Rows to remove"=3, "sub array start"=w1286, "error in (no error)"=w1288) -> ("row max value"=w1284:i32, 13:"start of last occupied row"=w1285:cluster{"row":i32, "column":i32}, 14:"start of last occupied row"=w1282:string, "error out"=w1287:errorcluster)  [unwired: 4 in, 3 out]
                n578 = Array Subset(array=w1289, index (col)=2 ("index")) -> ()  [unwired: 3 in, 1 out]
                n579 = local write "row max value"(w1284) -> ()
                n580 = local write "last occupied cell's name"(w1282) -> ()
              }
            }
          }
          frame "ORP Calibration Standard" {
            n581 = invoke on="Record Single Sample" class="Bool" method="Reinit To Default"(error in=w1363) -> (error out=w1362:errorcluster)  [unwired: 2 in, 2 out]
            n582 = call <vilib>:"Clear Errors.vi"("error in (no error)"=w1362) -> ("error out"=w1350:errorcluster)  [unwired: 5 in, 1 out]
            n583 = call "get sample sheet data cells.vi"("error in (no error)"=w1350, "NI_report in"=w1381) -> ("error out"=w1378:errorcluster, "data"=w1380:string[][], "NI_report out"=w1373:refnum<class "NI_report.lvclass">, "left edge output cluster"=w1379:cluster{"row":i32, "column":i32})  [unwired: 5 in, 1 out]
            n584 = flat-sequence {
              tunnel: w1378 -> [w1445]
              tunnel: [w1438] -> _
              tunnel: w1379 -> [w1443]
              tunnel: [w1442] -> w1377
              tunnel: [w1441] -> _
              tunnel: [w1440] -> w1371
              tunnel: w1380 -> [w1438]
              frame #0 {
                n585 = Array Subset(array=w1438, index (col)=2 ("index")) -> ()  [unwired: 3 in, 1 out]
                n586 = local read "Current Sample Sheet"() -> (w1437:string)
                n587 = call "find last occupied cell.vi"("data"=w1438, "Active Sheet"=w1437, "Header Rows to remove"=3, "sub array start"=w1443, "error in (no error)"=w1445) -> ("row max value"=w1441:i32, "column max value"=w1436:i32, 13:"start of last occupied row"=w1440:cluster{"row":i32, "column":i32}, 14:"start of last occupied row"=w1435:string, "error out"=w1442:errorcluster)  [unwired: 4 in, 2 out]
                n588 = local write "last occupied cell's name"(w1435) -> ()
                n589 = local write "row max value"(w1436) -> ()
              }
            }
            n590 = local read "Found Quanta Sonde Com Port"() -> (w1367:refnum<visa-resource-name>)
            n591 = Equal?(x=w1367, y=refnum<visa-resource-name> refnum ("RS232 Port Out")) -> (x = y?=w1369:bool)
            n592 = case shown="False" w1369 {
              tunnel: w1367 -> [w1397 _]
              tunnel: [w1407 w1431] -> w1370
              tunnel: w1377 -> [w1399 w1434]
              tunnel: [w1410 w1434] -> w1374
              tunnel: w1357 -> [w1406 w1433]
              tunnel: [w1405 w1421] -> w1356
              tunnel: [w1404 w1420] -> w1355
              tunnel: w1354 -> [w1403 w1432]
              tunnel: w1353 -> [_ w1417]
              frame False {
                n593 = control-ref of="Sonde Data Display"() -> (w1411:refnum<vi>)
                n594 = call "Calibrate ORP Sensor.vi"("Calibration Standard"="ORP Reference", "Error In (No Error)"=w1399, "Sensor Address In"="0", "RS232 Port In"=w1397) -> ("Error Out"=w1398:errorcluster, "Sensor Calibrate Response"=→"ORP  Reference\nCalibrate Response":bool, "RS232 Port Out"=w1396:refnum<visa-resource-name>)  [unwired: 4 in, 1 out]
                n595 = local read "Sample Sheet Data Row Cluster 2"() -> (w1408:T1)
                n596 = call "SDI-12 Single Operation with output cluster.vi"("RS232 Port In"=w1396, "Sensor Address In"="0", "Sonde Data Ctl Refnum"=w1411, "Error In (No Error)"=w1398, "Time Array In"=w1406, "Measurement Array In"=w1403) -> ("time array out"=w1405:dbl[], "Measurement  array Out"=w1404:dbl[][], "output cluster"=w1409:T2, "Temperature"=w1413:cluster{"Y":dbl[], "Y":dbl[]}[], "Sonde Data Display"=w1412:T13, "Error Out"=w1410:errorcluster)  [unwired: 12 in, 4 out]
                n597 = Bundle By Name(cluster=w1408, "Sonde Data Cluster"=w1409) -> (w1407:T1)
                n598 = local write "Temperature"(w1413) -> ()
                n599 = local write "Sonde Data Display"(w1412) -> ()
              }
              frame True {
                n600 = Get Date/Time In Seconds() -> (seconds since 1Jan1904=w1423:timestamp)
                n601 = To Double Precision Float(number=w1423) -> (double precision float=w1422:dbl)
                n602 = local read "Sample Sheet Data Row Cluster 2"() -> (w1431:T1)
                n603 = Subtract(x=w1422, y=w1417) -> (x-y=w1415:dbl)
                n604 = local write "Current Time (s)"(w1415) -> ()
                n605 = Unbundle By Name(w1431) -> ("Sonde Data Cluster.Temp"=w1416:dbl, "Sonde Data Cluster.pH"=w1430:dbl, "Sonde Data Cluster.Specific\nConductance"=w1429:dbl, "Sonde Data Cluster.Salinity"=w1428:dbl, "Sonde Data Cluster.Dissolved\nOxygen"=w1427:dbl, "Sonde Data Cluster.ORP"=w1426:dbl)  [unwired: 1 out]
                n606 = Build Array(w1416, w1430, w1429, w1428, w1427, 0.0 ("element"), w1426) -> (w1424:dbl[])
                n607 = Build Array (concatenate)(w1432, w1424) -> (w1420:dbl[][])
                n608 = Build Array (concatenate)(w1433, w1415) -> (w1421:dbl[])
                n609 = call "format into Sonde Vertical Graph Data Input.vi"("Sonde Measurement Array"=w1420, "Time Array"=w1421) -> ("Sonde Data Display"=w1419:T13, "Temperature"=w1418:cluster{"X":dbl[], "Y":dbl[]}[])  [unwired: 8 in]
                n610 = local write "Temperature"(w1418) -> ()
                n611 = local write "Sonde Data Display"(w1419) -> ()
              }
            }
            n612 = local write "Sample Sheet Data Row Cluster 2"(w1370) -> ()
            n613 = call "write out sonde row.vi"("NI_report in"=w1373, "Columns"=w1376, "Column of Volume"=w1375, "Sample Sheet Data Row Cluster"=w1370, "row index"=w1359, "error in (no error)"=w1374, "start of last occupied row"=w1371) -> ("NI_report out"=w1365:refnum<class "NI_report.lvclass">, "row index out"=w1358:i32, "error out"=w1366:errorcluster)  [unwired: 6 in]
            n614 = flat-sequence {
              tunnel: w1366 -> [w1395]
              tunnel: w1365 -> [w1394]
              tunnel: [w1393] -> w1364
              tunnel: [w1388] -> w1361
              tunnel: [w1386] -> w1360
              frame #0 {
                (unwired) 3 ("Header Rows to remove")
                n615 = call <vilib>:"Clear Errors.vi"("error in (no error)"=w1395) -> ("error out"=w1382:errorcluster)  [unwired: 5 in, 1 out]
                n616 = local read "Current Sample Sheet"() -> (w1384:string)
                n617 = call "get sample sheet data cells.vi"("error in (no error)"=w1382, "NI_report in"=w1394) -> ("error out"=w1389:errorcluster, "data"=w1390:string[][], "NI_report out"=w1393:refnum<class "NI_report.lvclass">, "left edge output cluster"=w1387:cluster{"row":i32, "column":i32})  [unwired: 5 in, 1 out]
                n618 = call "find last occupied cell.vi"("data"=w1390, "Active Sheet"=w1384, "Header Rows to remove"=3, "sub array start"=w1387, "error in (no error)"=w1389) -> ("row max value"=w1385:i32, 13:"start of last occupied row"=w1386:cluster{"row":i32, "column":i32}, 14:"start of last occupied row"=w1383:string, "error out"=w1388:errorcluster)  [unwired: 4 in, 3 out]
                n619 = Array Subset(array=w1390, index (col)=2 ("index")) -> ()  [unwired: 3 in, 1 out]
                n620 = local write "row max value"(w1385) -> ()
                n621 = local write "last occupied cell's name"(w1383) -> ()
              }
            }
          }
          frame "Salinity Calibration Standard" {
            n622 = invoke on="Record Single Sample" class="Bool" method="Reinit To Default"(error in=w1464) -> (error out=w1463:errorcluster)  [unwired: 2 in, 2 out]
            n623 = call <vilib>:"Clear Errors.vi"("error in (no error)"=w1463) -> ("error out"=w1451:errorcluster)  [unwired: 5 in, 1 out]
            n624 = call "get sample sheet data cells.vi"("error in (no error)"=w1451, "NI_report in"=w1482) -> ("error out"=w1479:errorcluster, "data"=w1481:string[][], "NI_report out"=w1474:refnum<class "NI_report.lvclass">, "left edge output cluster"=w1480:cluster{"row":i32, "column":i32})  [unwired: 5 in, 1 out]
            n625 = flat-sequence {
              tunnel: w1479 -> [w1546]
              tunnel: [w1539] -> _
              tunnel: w1480 -> [w1544]
              tunnel: [w1543] -> w1478
              tunnel: [w1542] -> _
              tunnel: [w1541] -> w1472
              tunnel: w1481 -> [w1539]
              frame #0 {
                n626 = Array Subset(array=w1539, index (col)=2 ("index")) -> ()  [unwired: 3 in, 1 out]
                n627 = local read "Current Sample Sheet"() -> (w1538:string)
                n628 = call "find last occupied cell.vi"("data"=w1539, "Active Sheet"=w1538, "Header Rows to remove"=3, "sub array start"=w1544, "error in (no error)"=w1546) -> ("row max value"=w1542:i32, "column max value"=w1537:i32, 13:"start of last occupied row"=w1541:cluster{"row":i32, "column":i32}, 14:"start of last occupied row"=w1536:string, "error out"=w1543:errorcluster)  [unwired: 4 in, 2 out]
                n629 = local write "last occupied cell's name"(w1536) -> ()
                n630 = local write "row max value"(w1537) -> ()
              }
            }
            n631 = local read "Found Quanta Sonde Com Port"() -> (w1468:refnum<visa-resource-name>)
            n632 = Equal?(x=w1468, y=refnum<visa-resource-name> refnum ("RS232 Port Out")) -> (x = y?=w1470:bool)
            n633 = case shown="False" w1470 {
              tunnel: w1468 -> [w1501 _]
              tunnel: [w1508 w1532] -> w1471
              tunnel: w1478 -> [w1499 w1535]
              tunnel: [w1511 w1535] -> w1475
              tunnel: w1458 -> [w1507 w1534]
              tunnel: [w1506 w1522] -> w1457
              tunnel: [w1505 w1521] -> w1456
              tunnel: w1455 -> [w1504 w1533]
              tunnel: w1454 -> [_ w1518]
              frame False {
                n634 = call "Calibrate Salinity Sensor.vi"("Calibration Standard"="Salinity \nReference", "Error In (No Error)"=w1499, "Sensor Address In"="0", "RS232 Port In"=w1501) -> ("Error Out"=w1498:errorcluster, "Sensor Calibrate Response"=→"Salinity  Reference\nCalibrate Response":bool, "RS232 Port Out"=w1500:refnum<visa-resource-name>)  [unwired: 4 in, 1 out]
                n635 = control-ref of="Sonde Data Display"() -> (w1512:refnum<vi>)
                n636 = local read "Sample Sheet Data Row Cluster 2"() -> (w1509:T1)
                n637 = call "SDI-12 Single Operation with output cluster.vi"("RS232 Port In"=w1500, "Sensor Address In"="0", "Sonde Data Ctl Refnum"=w1512, "Error In (No Error)"=w1498, "Time Array In"=w1507, "Measurement Array In"=w1504) -> ("time array out"=w1506:dbl[], "Measurement  array Out"=w1505:dbl[][], "output cluster"=w1510:T2, "Temperature"=w1514:cluster{"Y":dbl[], "Y":dbl[]}[], "Sonde Data Display"=w1513:T13, "Error Out"=w1511:errorcluster)  [unwired: 12 in, 4 out]
                n638 = local write "Temperature"(w1514) -> ()
                n639 = local write "Sonde Data Display"(w1513) -> ()
                n640 = Bundle By Name(cluster=w1509, "Sonde Data Cluster"=w1510) -> (w1508:T1)
              }
              frame True {
                n641 = Get Date/Time In Seconds() -> (seconds since 1Jan1904=w1524:timestamp)
                n642 = To Double Precision Float(number=w1524) -> (double precision float=w1523:dbl)
                n643 = local read "Sample Sheet Data Row Cluster 2"() -> (w1532:T1)
                n644 = Subtract(x=w1523, y=w1518) -> (x-y=w1516:dbl)
                n645 = local write "Current Time (s)"(w1516) -> ()
                n646 = Unbundle By Name(w1532) -> ("Sonde Data Cluster.Temp"=w1517:dbl, "Sonde Data Cluster.pH"=w1531:dbl, "Sonde Data Cluster.Specific\nConductance"=w1530:dbl, "Sonde Data Cluster.Salinity"=w1529:dbl, "Sonde Data Cluster.Dissolved\nOxygen"=w1528:dbl, "Sonde Data Cluster.ORP"=w1527:dbl)  [unwired: 1 out]
                n647 = Build Array(w1517, w1531, w1530, w1529, w1528, 0.0 ("element"), w1527) -> (w1525:dbl[])
                n648 = Build Array (concatenate)(w1533, w1525) -> (w1521:dbl[][])
                n649 = Build Array (concatenate)(w1534, w1516) -> (w1522:dbl[])
                n650 = call "format into Sonde Vertical Graph Data Input.vi"("Sonde Measurement Array"=w1521, "Time Array"=w1522) -> ("Sonde Data Display"=w1520:T13, "Temperature"=w1519:cluster{"X":dbl[], "Y":dbl[]}[])  [unwired: 8 in]
                n651 = local write "Temperature"(w1519) -> ()
                n652 = local write "Sonde Data Display"(w1520) -> ()
              }
            }
            n653 = local write "Sample Sheet Data Row Cluster 2"(w1471) -> ()
            n654 = call "write out sonde row.vi"("NI_report in"=w1474, "Columns"=w1477, "Column of Volume"=w1476, "Sample Sheet Data Row Cluster"=w1471, "row index"=w1460, "error in (no error)"=w1475, "start of last occupied row"=w1472) -> ("NI_report out"=w1466:refnum<class "NI_report.lvclass">, "row index out"=w1459:i32, "error out"=w1467:errorcluster)  [unwired: 6 in]
            n655 = flat-sequence {
              tunnel: w1467 -> [w1496]
              tunnel: w1466 -> [w1495]
              tunnel: [w1494] -> w1465
              tunnel: [w1489] -> w1462
              tunnel: [w1487] -> w1461
              frame #0 {
                (unwired) 3 ("Header Rows to remove")
                n656 = call <vilib>:"Clear Errors.vi"("error in (no error)"=w1496) -> ("error out"=w1483:errorcluster)  [unwired: 5 in, 1 out]
                n657 = local read "Current Sample Sheet"() -> (w1485:string)
                n658 = call "get sample sheet data cells.vi"("error in (no error)"=w1483, "NI_report in"=w1495) -> ("error out"=w1490:errorcluster, "data"=w1491:string[][], "NI_report out"=w1494:refnum<class "NI_report.lvclass">, "left edge output cluster"=w1488:cluster{"row":i32, "column":i32})  [unwired: 5 in, 1 out]
                n659 = call "find last occupied cell.vi"("data"=w1491, "Active Sheet"=w1485, "Header Rows to remove"=3, "sub array start"=w1488, "error in (no error)"=w1490) -> ("row max value"=w1486:i32, 13:"start of last occupied row"=w1487:cluster{"row":i32, "column":i32}, 14:"start of last occupied row"=w1484:string, "error out"=w1489:errorcluster)  [unwired: 4 in, 3 out]
                n660 = Array Subset(array=w1491, index (col)=2 ("index")) -> ()  [unwired: 3 in, 1 out]
                n661 = local write "row max value"(w1486) -> ()
                n662 = local write "last occupied cell's name"(w1484) -> ()
              }
            }
          }
          frame "DO Calibration Standard" {
            n663 = invoke on="Record Single Sample" class="Bool" method="Reinit To Default"(error in=w1565) -> (error out=w1564:errorcluster)  [unwired: 2 in, 2 out]
            n664 = call <vilib>:"Clear Errors.vi"("error in (no error)"=w1564) -> ("error out"=w1552:errorcluster)  [unwired: 5 in, 1 out]
            n665 = call "get sample sheet data cells.vi"("error in (no error)"=w1552, "NI_report in"=w1583) -> ("error out"=w1580:errorcluster, "data"=w1582:string[][], "NI_report out"=w1575:refnum<class "NI_report.lvclass">, "left edge output cluster"=w1581:cluster{"row":i32, "column":i32})  [unwired: 5 in, 1 out]
            n666 = flat-sequence {
              tunnel: w1580 -> [w1646]
              tunnel: [w1639] -> _
              tunnel: w1581 -> [w1644]
              tunnel: [w1643] -> w1579
              tunnel: [w1642] -> _
              tunnel: [w1641] -> w1573
              tunnel: w1582 -> [w1639]
              frame #0 {
                n667 = Array Subset(array=w1639, index (col)=2 ("index")) -> ()  [unwired: 3 in, 1 out]
                n668 = local read "Current Sample Sheet"() -> (w1638:string)
                n669 = call "find last occupied cell.vi"("data"=w1639, "Active Sheet"=w1638, "Header Rows to remove"=3, "sub array start"=w1644, "error in (no error)"=w1646) -> ("row max value"=w1642:i32, "column max value"=w1637:i32, 13:"start of last occupied row"=w1641:cluster{"row":i32, "column":i32}, 14:"start of last occupied row"=w1636:string, "error out"=w1643:errorcluster)  [unwired: 4 in, 2 out]
                n670 = local write "last occupied cell's name"(w1636) -> ()
                n671 = local write "row max value"(w1637) -> ()
              }
            }
            n672 = local read "Found Quanta Sonde Com Port"() -> (w1569:refnum<visa-resource-name>)
            n673 = Equal?(x=w1569, y=refnum<visa-resource-name> refnum ("RS232 Port Out")) -> (x = y?=w1571:bool)
            n674 = case shown="False" w1571 {
              tunnel: w1569 -> [w1601 _]
              tunnel: [w1608 w1632] -> w1572
              tunnel: w1579 -> [w1603 w1635]
              tunnel: [w1611 w1635] -> w1576
              tunnel: w1559 -> [w1607 w1634]
              tunnel: [w1606 w1622] -> w1558
              tunnel: [w1605 w1621] -> w1557
              tunnel: w1556 -> [w1604 w1633]
              tunnel: w1555 -> [_ w1618]
              frame False {
                n675 = call "Calibrate DO Sensor.vi"("Calibration Standard"="DO \nReference", "Error In (No Error)"=w1603, "Sensor Address In"="0", "RS232 Port In"=w1601) -> ("Error Out"=w1602:errorcluster, "Sensor Calibrate Response"=→"DO  Reference\nCalibrate Response":bool, "RS232 Port Out"=w1600:refnum<visa-resource-name>)  [unwired: 4 in, 1 out]
                n676 = control-ref of="Sonde Data Display"() -> (w1612:refnum<vi>)
                n677 = local read "Sample Sheet Data Row Cluster 2"() -> (w1609:T1)
                n678 = call "SDI-12 Single Operation with output cluster.vi"("RS232 Port In"=w1600, "Sensor Address In"="0", "Sonde Data Ctl Refnum"=w1612, "Error In (No Error)"=w1602, "Time Array In"=w1607, "Measurement Array In"=w1604) -> ("time array out"=w1606:dbl[], "Measurement  array Out"=w1605:dbl[][], "output cluster"=w1610:T2, "Temperature"=w1614:cluster{"Y":dbl[], "Y":dbl[]}[], "Sonde Data Display"=w1613:T13, "Error Out"=w1611:errorcluster)  [unwired: 12 in, 4 out]
                n679 = local write "Temperature"(w1614) -> ()
                n680 = local write "Sonde Data Display"(w1613) -> ()
                n681 = Bundle By Name(cluster=w1609, "Sonde Data Cluster"=w1610) -> (w1608:T1)
              }
              frame True {
                n682 = Get Date/Time In Seconds() -> (seconds since 1Jan1904=w1624:timestamp)
                n683 = To Double Precision Float(number=w1624) -> (double precision float=w1623:dbl)
                n684 = local read "Sample Sheet Data Row Cluster 2"() -> (w1632:T1)
                n685 = Subtract(x=w1623, y=w1618) -> (x-y=w1616:dbl)
                n686 = local write "Current Time (s)"(w1616) -> ()
                n687 = Unbundle By Name(w1632) -> ("Sonde Data Cluster.Temp"=w1617:dbl, "Sonde Data Cluster.pH"=w1631:dbl, "Sonde Data Cluster.Specific\nConductance"=w1630:dbl, "Sonde Data Cluster.Salinity"=w1629:dbl, "Sonde Data Cluster.Dissolved\nOxygen"=w1628:dbl, "Sonde Data Cluster.ORP"=w1627:dbl)  [unwired: 1 out]
                n688 = Build Array(w1617, w1631, w1630, w1629, w1628, 0.0 ("element"), w1627) -> (w1625:dbl[])
                n689 = Build Array (concatenate)(w1633, w1625) -> (w1621:dbl[][])
                n690 = Build Array (concatenate)(w1634, w1616) -> (w1622:dbl[])
                n691 = call "format into Sonde Vertical Graph Data Input.vi"("Sonde Measurement Array"=w1621, "Time Array"=w1622) -> ("Sonde Data Display"=w1620:T13, "Temperature"=w1619:cluster{"X":dbl[], "Y":dbl[]}[])  [unwired: 8 in]
                n692 = local write "Temperature"(w1619) -> ()
                n693 = local write "Sonde Data Display"(w1620) -> ()
              }
            }
            n694 = local write "Sample Sheet Data Row Cluster 2"(w1572) -> ()
            n695 = call "write out sonde row.vi"("NI_report in"=w1575, "Columns"=w1578, "Column of Volume"=w1577, "Sample Sheet Data Row Cluster"=w1572, "row index"=w1561, "error in (no error)"=w1576, "start of last occupied row"=w1573) -> ("NI_report out"=w1567:refnum<class "NI_report.lvclass">, "row index out"=w1560:i32, "error out"=w1568:errorcluster)  [unwired: 6 in]
            n696 = flat-sequence {
              tunnel: w1568 -> [w1596]
              tunnel: w1567 -> [w1595]
              tunnel: [w1594] -> w1566
              tunnel: [w1590] -> w1563
              tunnel: [w1588] -> w1562
              frame #0 {
                (unwired) 3 ("Header Rows to remove")
                n697 = call <vilib>:"Clear Errors.vi"("error in (no error)"=w1596) -> ("error out"=w1584:errorcluster)  [unwired: 5 in, 1 out]
                n698 = local read "Current Sample Sheet"() -> (w1586:string)
                n699 = call "get sample sheet data cells.vi"("error in (no error)"=w1584, "NI_report in"=w1595) -> ("error out"=w1591:errorcluster, "data"=w1592:string[][], "NI_report out"=w1594:refnum<class "NI_report.lvclass">, "left edge output cluster"=w1589:cluster{"row":i32, "column":i32})  [unwired: 5 in, 1 out]
                n700 = call "find last occupied cell.vi"("data"=w1592, "Active Sheet"=w1586, "Header Rows to remove"=3, "sub array start"=w1589, "error in (no error)"=w1591) -> ("row max value"=w1587:i32, 13:"start of last occupied row"=w1588:cluster{"row":i32, "column":i32}, 14:"start of last occupied row"=w1585:string, "error out"=w1590:errorcluster)  [unwired: 4 in, 3 out]
                n701 = local write "row max value"(w1587) -> ()
                n702 = local write "last occupied cell's name"(w1585) -> ()
              }
            }
          }
          frame "SC Calibration Standard" {
            n703 = invoke on="Record Single Sample" class="Bool" method="Reinit To Default"(error in=w1665) -> (error out=w1664:errorcluster)  [unwired: 2 in, 2 out]
            n704 = call <vilib>:"Clear Errors.vi"("error in (no error)"=w1664) -> ("error out"=w1652:errorcluster)  [unwired: 5 in, 1 out]
            n705 = call "get sample sheet data cells.vi"("error in (no error)"=w1652, "NI_report in"=w1683) -> ("error out"=w1680:errorcluster, "data"=w1682:string[][], "NI_report out"=w1675:refnum<class "NI_report.lvclass">, "left edge output cluster"=w1681:cluster{"row":i32, "column":i32})  [unwired: 5 in, 1 out]
            n706 = flat-sequence {
              tunnel: w1680 -> [w1746]
              tunnel: [w1740] -> _
              tunnel: w1681 -> [w1744]
              tunnel: [w1743] -> w1679
              tunnel: [w1742] -> _
              tunnel: [w1741] -> w1673
              tunnel: w1682 -> [w1740]
              frame #0 {
                n707 = local read "Current Sample Sheet"() -> (w1739:string)
                n708 = call "find last occupied cell.vi"("data"=w1740, "Active Sheet"=w1739, "Header Rows to remove"=3, "sub array start"=w1744, "error in (no error)"=w1746) -> ("row max value"=w1742:i32, "column max value"=w1738:i32, 13:"start of last occupied row"=w1741:cluster{"row":i32, "column":i32}, 14:"start of last occupied row"=w1737:string, "error out"=w1743:errorcluster)  [unwired: 4 in, 2 out]
                n709 = local write "last occupied cell's name"(w1737) -> ()
                n710 = local write "row max value"(w1738) -> ()
              }
            }
            n711 = local read "Found Quanta Sonde Com Port"() -> (w1669:refnum<visa-resource-name>)
            n712 = Equal?(x=w1669, y=refnum<visa-resource-name> refnum ("RS232 Port Out")) -> (x = y?=w1671:bool)
            n713 = case shown="False" w1671 {
              tunnel: w1669 -> [w1703 _]
              tunnel: [w1709 w1733] -> w1672
              tunnel: w1679 -> [w1701 w1736]
              tunnel: [w1712 w1736] -> w1676
              tunnel: w1659 -> [w1708 w1735]
              tunnel: [w1707 w1723] -> w1658
              tunnel: [w1706 w1722] -> w1657
              tunnel: w1656 -> [w1705 w1734]
              tunnel: w1655 -> [_ w1719]
              frame False {
                n714 = call "Calibrate SC Sensor.vi"("Calibration Standard"="SC \nReference", "Error In (No Error)"=w1701, "Sensor Address In"="0", "RS232 Port In"=w1703) -> ("Error Out"=w1700:errorcluster, "Sensor Calibrate Response"=→"SC  Reference\nCalibrate Response":bool, "RS232 Port Out"=w1702:refnum<visa-resource-name>)  [unwired: 4 in, 1 out]
                n715 = control-ref of="Sonde Data Display"() -> (w1713:refnum<vi>)
                n716 = local read "Sample Sheet Data Row Cluster 2"() -> (w1710:T1)
                n717 = call <vilib>:"Clear Errors.vi"("error in (no error)"=w1700) -> ("error out"=w1697:errorcluster)  [unwired: 5 in, 1 out]
                n718 = call "SDI-12 Single Operation with output cluster.vi"("RS232 Port In"=w1702, "Sensor Address In"="0", "Sonde Data Ctl Refnum"=w1713, "Error In (No Error)"=w1697, "Time Array In"=w1708, "Measurement Array In"=w1705) -> ("time array out"=w1707:dbl[], "Measurement  array Out"=w1706:dbl[][], "output cluster"=w1711:T2, "Temperature"=w1715:cluster{"Y":dbl[], "Y":dbl[]}[], "Sonde Data Display"=w1714:T13, "Error Out"=w1712:errorcluster)  [unwired: 12 in, 4 out]
                n719 = local write "Temperature"(w1715) -> ()
                n720 = local write "Sonde Data Display"(w1714) -> ()
                n721 = Bundle By Name(cluster=w1710, "Sonde Data Cluster"=w1711) -> (w1709:T1)
              }
              frame True {
                n722 = Get Date/Time In Seconds() -> (seconds since 1Jan1904=w1725:timestamp)
                n723 = To Double Precision Float(number=w1725) -> (double precision float=w1724:dbl)
                n724 = local read "Sample Sheet Data Row Cluster 2"() -> (w1733:T1)
                n725 = Subtract(x=w1724, y=w1719) -> (x-y=w1717:dbl)
                n726 = local write "Current Time (s)"(w1717) -> ()
                n727 = Unbundle By Name(w1733) -> ("Sonde Data Cluster.Temp"=w1718:dbl, "Sonde Data Cluster.pH"=w1732:dbl, "Sonde Data Cluster.Specific\nConductance"=w1731:dbl, "Sonde Data Cluster.Salinity"=w1730:dbl, "Sonde Data Cluster.Dissolved\nOxygen"=w1729:dbl, "Sonde Data Cluster.ORP"=w1728:dbl)  [unwired: 1 out]
                n728 = Build Array(w1718, w1732, w1731, w1730, w1729, 0.0 ("element"), w1728) -> (w1726:dbl[])
                n729 = Build Array (concatenate)(w1734, w1726) -> (w1722:dbl[][])
                n730 = Build Array (concatenate)(w1735, w1717) -> (w1723:dbl[])
                n731 = call "format into Sonde Vertical Graph Data Input.vi"("Sonde Measurement Array"=w1722, "Time Array"=w1723) -> ("Sonde Data Display"=w1721:T13, "Temperature"=w1720:cluster{"X":dbl[], "Y":dbl[]}[])  [unwired: 8 in]
                n732 = local write "Temperature"(w1720) -> ()
                n733 = local write "Sonde Data Display"(w1721) -> ()
              }
            }
            n734 = local write "Sample Sheet Data Row Cluster 2"(w1672) -> ()
            n735 = call "write out sonde row.vi"("NI_report in"=w1675, "Columns"=w1678, "Column of Volume"=w1677, "Sample Sheet Data Row Cluster"=w1672, "row index"=w1661, "error in (no error)"=w1676, "start of last occupied row"=w1673) -> ("NI_report out"=w1667:refnum<class "NI_report.lvclass">, "row index out"=w1660:i32, "error out"=w1668:errorcluster)  [unwired: 6 in]
            n736 = flat-sequence {
              tunnel: w1668 -> [w1696]
              tunnel: w1667 -> [w1695]
              tunnel: [w1694] -> w1666
              tunnel: [w1690] -> w1663
              tunnel: [w1688] -> w1662
              frame #0 {
                (unwired) 3 ("Header Rows to remove")
                (unwired) 2 ("index")
                n737 = call <vilib>:"Clear Errors.vi"("error in (no error)"=w1696) -> ("error out"=w1684:errorcluster)  [unwired: 5 in, 1 out]
                n738 = local read "Current Sample Sheet"() -> (w1686:string)
                n739 = call "get sample sheet data cells.vi"("error in (no error)"=w1684, "NI_report in"=w1695) -> ("error out"=w1691:errorcluster, "data"=w1692:string[][], "NI_report out"=w1694:refnum<class "NI_report.lvclass">, "left edge output cluster"=w1689:cluster{"row":i32, "column":i32})  [unwired: 5 in, 1 out]
                n740 = call "find last occupied cell.vi"("data"=w1692, "Active Sheet"=w1686, "Header Rows to remove"=3, "sub array start"=w1689, "error in (no error)"=w1691) -> ("row max value"=w1687:i32, 13:"start of last occupied row"=w1688:cluster{"row":i32, "column":i32}, 14:"start of last occupied row"=w1685:string, "error out"=w1690:errorcluster)  [unwired: 4 in, 3 out]
                n741 = local write "row max value"(w1687) -> ()
                n742 = local write "last occupied cell's name"(w1685) -> ()
              }
            }
          }
          frame "Write Sonde Sample Sheet" {
            n743 = flat-sequence {
              tunnel: w1747 -> [w1785]
              frame #0 {
                n744 = local read "Sonde Data Array"() -> (w1788:T11[])
                n745 = Index Array(array=w1788, index=w1785) -> (element=w1790:T11)
                n746 = Bundle By Name(cluster=w1790, "Final"=TRUE) -> (w1786:T11)
                n747 = Replace Array Subset(array=w1788, new element=w1786, index=w1785) -> (w1787:T11[])
                n748 = local write "Sonde Data Array"(w1787) -> ()
              }
            }
            n749 = Not Equal?(x=w1774, y=w1773) -> (x != y?=w1772:bool)
            n750 = Decrement(x=w1747) -> (x-1=w1759:i32)
            n751 = case shown="True" w1772 {
              tunnel: w1784 -> [w1793 w1800]
              tunnel: w1771 -> [_ w1799]
              tunnel: w1783 -> [w1792 w1798]
              tunnel: [w1792 w1797] -> w1782
              tunnel: [w1793 w1796] -> w1781
              tunnel: w1776 -> [w1791 w1795]
              tunnel: [w1791 w1794] -> w1775
              frame False {
              }
              frame True {
                n752 = flat-sequence {
                  tunnel: [w1809] -> w1796
                  tunnel: w1800 -> [w1808]
                  tunnel: w1799 -> [w1805]
                  tunnel: w1798 -> [w1804]
                  tunnel: [w1803] -> w1797
                  tunnel: w1795 -> [w1802]
                  tunnel: [w1801] -> w1794
                  frame #0 {
                    n753 = Increment(x=w1802) -> (x+1=w1801:i32)
                    n754 = call "write comment cell with column offset.vi"("Column Relative?"=TRUE, "comment string"="done", "error in (no error)"=w1804, "start of last occupied row"=w1805, "NI_report in"=w1808) -> ("error out"=w1803:errorcluster, "NI_report out"=w1809:refnum<class "NI_report.lvclass">)  [unwired: 5 in]
                  }
                }
              }
            }
            n755 = call "open select sample sheet.vi"("Number of Sample Sheets"=w1777, "error in (no error)"=w1782, "Worksheet Names"=w1778, "Active Sample Sheet"=w1775, "NI_report in"=w1781) -> ("error out"=w1768:errorcluster, "Current Sample Sheet"=w1769:string, "NI_report out"=w1767:refnum<class "NI_report.lvclass">)  [unwired: 3 in, 1 out]
            n756 = local write "Current Sample Sheet"(w1769) -> ()
            n757 = local read "Current Sample Sheet"() -> (w1761:string)
            n758 = call "get sample sheet data cells.vi"("error in (no error)"=w1768, "NI_report in"=w1767) -> ("error out"=w1780:errorcluster, "data"=w1765:string[][], "NI_report out"=w1779:refnum<class "NI_report.lvclass">, "left edge output cluster"=w1763:cluster{"row":i32, "column":i32})  [unwired: 5 in, 1 out]
            n759 = Array Subset(array=w1765, index (col)=2 ("index")) -> ()  [unwired: 3 in, 1 out]
            n760 = call "find last occupied cell.vi"("Active Sheet"=w1761, "Header Rows to remove"=3, "sub array start"=w1763, "error in (no error)"=w1780) -> ("row max value"=w1762:i32, 13:"start of last occupied row"=w1770:cluster{"row":i32, "column":i32}, 14:"start of last occupied row"=w1760:string, "error out"=w1754:errorcluster)  [unwired: 5 in, 3 out]
            n761 = local write "row max value"(w1762) -> ()
            n762 = local write "last occupied cell's name"(w1760) -> ()
            n763 = local write "Sonde Data Array"(T11[] [{"Head"=0.0, "Depth"=0.0, "Time"="19:00", "Cumulative\nVolume"=0.0, "Sp. Conductance"={"Value"=0.506, "%"=0.0, "Tol."=TRUE}, "Dissolved Oxygen"={"Value"=35.14, "%"=0.0, "Tol."=TRUE}, "pH"={"Value"=4.81, "%"=0.0, "Tol."=TRUE}, "ORP"={"Value"=390.0, "%"=0.0, "Tol."=TRUE}, "Temperature"={"Value"=23.86, "%"=0.0, "Tol."=TRUE}, "Salinity"={"Value"=0.24, "%"=0.0, "Tol."=TRUE}, "Final Tol."=TRUE, "Final"=FALSE}, {"Head"=0.0, "Depth"=0.0, "Time"="19:00", "Cumulative\nVolume"=0.0, "Sp. Conductance"={"Value"=0.506, "%"=0.0, "Tol."=TRUE}, "Dissolved Oxygen"={"Value"=35.12, "%"=0.0, "Tol."=TRUE}, "pH"={"Value"=4.81, "%"=0.0, "Tol."=TRUE}, "ORP"={"Value"=390.0, "%"=0.0, "Tol."=TRUE}, "Temperature"={"Value"=23.89, "%"=0.0, "Tol."=TRUE}, "Salinity"={"Value"=0.24, "%"=0.0, "Tol."=TRUE}, "Final Tol."=TRUE, "Final"=FALSE}, {"Head"=0.0, "Depth"=0.0, "Time"="19:00", "Cumulative\nVolume"=0.0, "Sp. Conductance"={"Value"=0.506, "%"=0.0, "Tol."=TRUE}, "Dissolved Oxygen"={"Value"=35.14, "%"=0.0, "Tol."=TRUE}, "pH"={"Value"=4.81, "%"=0.0, "Tol."=TRUE}, "ORP"={"Value"=390.0, "%"=0.0, "Tol."=TRUE}, "Temperature"={"Value"=23.86, "%"=0.0, "Tol."=TRUE}, "Salinity"={"Value"=0.24, "%"=0.0, "Tol."=TRUE}, "Final Tol."=TRUE, "Final"=FALSE}, {"Head"=0.0, "Depth"=0.0, "Time"="", "Cumulative\nVolume"=0.0, "Sp. Conductance"={"Value"=0.0, "%"=0.0, "Tol."=FALSE}, "Dissolved Oxygen"={"Value"=0.0, "%"=0.0, "Tol."=FALSE}, "pH"={"Value"=0.0, "%"=0.0, "Tol."=FALSE}, "ORP"={"Value"=0.0, "%"=0.0, "Tol."=FALSE}, "Temperature"={"Value"=0.0, "%"=0.0, "Tol."=FALSE}, "Salinity"={"Value"=0.0, "%"=0.0, "Tol."=FALSE}, "Final Tol."=FALSE, "Final"=FALSE}, {"Head"=0.0, "Depth"=0.0, "Time"="", "Cumulative\nVolume"=0.0, "Sp. Conductance"={"Value"=0.0, "%"=0.0, "Tol."=FALSE}, "Dissolved Oxygen"={"Value"=0.0, "%"=0.0, "Tol."=FALSE}, "pH"={"Value"=0.0, "%"=0.0, "Tol."=FALSE}, "ORP"={"Value"=0.0, "%"=0.0, "Tol."=FALSE}, "Temperature"={"Value"=0.0, "%"=0.0, "Tol."=FALSE}, "Salinity"={"Value"=0.0, "%"=0.0, "Tol."=FALSE}, "Final Tol."=FALSE, "Final"=FALSE}, {"Head"=0.0, "Depth"=0.0, "Time"="", "Cumulative\nVolume"=0.0, "Sp. Conductance"={"Value"=0.0, "%"=0.0, "Tol."=FALSE}, "Dissolved Oxygen"={"Value"=0.0, "%"=0.0, "Tol."=FALSE}, "pH"={"Value"=0.0, "%"=0.0, "Tol."=FALSE}, "ORP"={"Value"=0.0, "%"=0.0, "Tol."=FALSE}, "Temperature"={"Value"=0.0, "%"=0.0, "Tol."=FALSE}, "Salinity"={"Value"=0.0, "%"=0.0, "Tol."=FALSE}, "Final Tol."=FALSE, "Final"=FALSE}, {"Head"=0.0, "Depth"=0.0, "Time"="", "Cumulative\nVolume"=0.0, "Sp. Conductance"={"Value"=0.0, "%"=0.0, "Tol."=FALSE}, "Dissolved Oxygen"={"Value"=0.0, "%"=0.0, "Tol."=FALSE}, "pH"={"Value"=0.0, "%"=0.0, "Tol."=FALSE}, "ORP"={"Value"=0.0, "%"=0.0, "Tol."=FALSE}, "Temperature"={"Value"=0.0, "%"=0.0, "Tol."=FALSE}, "Salinity"={"Value"=0.0, "%"=0.0, "Tol."=FALSE}, "Final Tol."=FALSE, "Final"=FALSE}, {"Head"=0.0, "Depth"=0.0, "Time"="", "Cumulative\nVolume"=0.0, "Sp. Conductance"={"Value"=0.0, "%"=0.0, "Tol."=FALSE}, "Dissolved Oxygen"={"Value"=0.0, "%"=0.0, "Tol."=FALSE}, "pH"={"Value"=0.0, "%"=0.0, "Tol."=FALSE}, "ORP"={"Value"=0.0, "%"=0.0, "Tol."=FALSE}, "Temperature"={"Value"=0.0, "%"=0.0, "Tol."=FALSE}, "Salinity"={"Value"=0.0, "%"=0.0, "Tol."=FALSE}, "Final Tol."=FALSE, "Final"=FALSE}, {"Head"=0.0, "Depth"=0.0, "Time"="", "Cumulative\nVolume"=0.0, "Sp. Conductance"={"Value"=0.0, "%"=0.0, "Tol."=FALSE}, "Dissolved Oxygen"={"Value"=0.0, "%"=0.0, "Tol."=FALSE}, "pH"={"Value"=0.0, "%"=0.0, "Tol."=FALSE}, "ORP"={"Value"=0.0, "%"=0.0, "Tol."=FALSE}, "Temperature"={"Value"=0.0, "%"=0.0, "Tol."=FALSE}, "Salinity"={"Value"=0.0, "%"=0.0, "Tol."=FALSE}, "Final Tol."=FALSE, "Final"=FALSE}] ("Sonde Data Array")) -> ()
          }
          frame "Init" {
            n764 = flat-sequence {
              tunnel: w1827 -> [w2172]
              tunnel: [w2158] -> w1817
              tunnel: [w2157] -> w1816
              frame #0 {
                n765 = call "create DAQ strings.vi"("error in (no error)"=w2172, "MCC USB-DAQ Setup"="MCC USB-DAQ Setup") -> ("error IO"=w2165:errorcluster, "Descriptions"=w2163:string[], "delimited string"=w2166:string, "Array"=w2164:string[], "Voltage Range"=w2171:dbl[])  [unwired: 5 in]
                "delimited string" <- w2166
                "Active Channel Array" <- w2164
                "Voltage Range" <- w2171
                "Descriptions" <- w2163
                n766 = call "Physical Channels to Number of channels.vi"("error in (no error)"=w2165, "Physical Channel in"=w2166) -> ("error out"=w2167:errorcluster, "Number of Channels"=w2169:i32)  [unwired: 7 in, 1 out]
                "Number \nof Channels" <- w2169
                n767 = call "Calculate Rate from Num Channels and Max Rate.vi"("error in (no error)"=w2167, "Channel Data Rate S/s"="Channel \nData Rate S/s", "Number of Channels"=w2169) -> ("error out"=w2161:errorcluster, "Rate"=→"Rate":dbl)  [unwired: 7 in]
                n768 = for {
                  tunnel: w2164 -> [w2185] mode=indexing
                  tunnel: w2171 -> [w2184] mode=indexing
                  tunnel: [w2181] -> w2160 mode=indexing
                  shift-right: [w2182] -> w2159
                  shift-left: w2161 -> [w2180]
                  n769 = Negate(x=w2184) -> (-x=w2183:dbl)
                  n770 = call-poly <vilib>:"ULx Create Virtual Channel.vi"("maximum value"=w2184, "minimum value"=w2183, "physical channels"=w2185, "error in"=w2180) -> ("task out"=w2181:refnum<k24>, "error out"=w2182:errorcluster)  [unwired: 10 in]
                }
                n771 = call "get 9V monitor voltage.vi"("error in (no error)"=w2159, "Descriptions"=w2163, "Array"=w2164, "Array 2"=w2160) -> ("error out"=w2158:errorcluster, "9V Voltage Monitor"=→"9V Voltage Monitor":dbl)  [unwired: 6 in]
                "DAQ Error" <- w2158
                n772 = flat-sequence {
                  tunnel: [w2178] -> w2157
                  tunnel: w2160 -> [w2176]
                  tunnel: w2158 -> [w2175]
                  frame #0 {
                    n773 = local read "Descriptions"() -> (w2179:string[])
                    n774 = call "Measure DAQ Voltages.vi"("error in (no error)"=w2175, "Descriptions"=w2179, "Array in"=w2176) -> ("Raw Voltages"=w2177:dbl[], "Array out"=w2178:refnum<k24>[], "Sensor Cluster"=w2174:T9)  [unwired: 6 in]
                    n775 = local write "Sensor Voltage Cluster"(w2174) -> ()
                    n776 = local write "Raw Voltages"(w2177) -> ()
                  }
                }
              }
            }
            n777 = local write "Initialization"(-1 ("Initialization")) -> ()
            n778 = flat-sequence {
              tunnel: w1817 -> [w2150]
              tunnel: [w2150] -> w1825
              frame #0 {
                w2151 = T22."Enabled" ("Disabled")
                n779 = property on="Write Data to Spreadsheet" class="Bool"("DisabledEnum"=w2151) -> (error out=w2154:errorcluster)  [unwired: 2 in, 1 out]
                n780 = property on="Record Continuous Samples" class="Bool"(error in=w2154, "DisabledEnum"=T22."Disabled and Grayed Out" ("Disabled")) -> (error out=w2153:errorcluster)  [unwired: 1 in, 1 out]
                n781 = property on="Record Single Sample" class="Bool"(error in=w2153, "DisabledEnum"=w2151) -> (error out=w2152:errorcluster)  [unwired: 1 in, 1 out]
                n782 = property on="Sample Not Collected" class="Bool"(error in=w2152, "DisabledEnum"=w2151) -> (error out=w2149:errorcluster)  [unwired: 1 in, 1 out]
                n783 = invoke on="Sonde Data Array" class="Arr (strict)" method="Reinit To Default"(error in=w2149) -> ()  [unwired: 2 in, 3 out]
                "Initialization Finished" <- TRUE
              }
            }
            n784 = disable-structure shown="Enabled" {
              disable-tunnel: [w1834 _] -> w1820
              disable-tunnel: w1819 -> [w1839 w2105]
              disable-tunnel: [w1838 w2105] -> w1818
              disable-tunnel: w1817 -> [w1837 _]
              disable-tunnel: w1816 -> [w1835 _]
              frame Enabled {
                n785 = local read "Descriptions"() -> (w1836:string[])
                n786 = stacked-sequence {
                  seq-local: [w1840 _ _ _ _ _ _ _ _ _ _] -> [_ w1868 _ _ _ _ _ _ _ _ _]
                  seq-local: [_ w1869 _ _ _ _ _ _ _ _ _] -> [_ _ w1893 _ _ _ _ _ _ _ _]
                  seq-local: [_ _ w1892 _ _ _ _ _ _ _ _] -> [_ _ _ _ _ _ _ _ _ _ w2096]
                  tunnel: [_ _ w1897 _ _ _ _ _ _ _ _] -> _
                  tunnel: [_ _ _ _ _ _ errorcluster {"status"=FALSE, "code"=0, "source"=""} ("error out") _ _ _ _] -> _
                  tunnel: w1839 -> [_ _ _ _ _ _ _ _ _ _ w2100]
                  tunnel: [_ _ _ _ _ _ _ _ _ _ w2099] -> w1838
                  tunnel: w1837 -> [w1842 _ _ _ _ _ _ _ _ _ _]
                  tunnel: w1835 -> [_ _ w1895 w1977 w2005 w2031 _ _ _ w2070 _]
                  tunnel: w1836 -> [_ _ w1894 w1978 w2004 w2030 _ _ _ w2068 _]
                  tunnel: [_ _ _ w1979 _ _ _ _ _ _ _] -> _
                  tunnel: [_ _ _ _ _ _ _ _ _ _ w2096] -> w1834
                  frame #0 {
                    n787 = flat-sequence {
                      tunnel: [w1847] -> w1840
                      tunnel: w1842 -> [w1848]
                      frame #0 {
                        n788 = local read "Groundwater Header"() -> (w1854:T10)
                        n789 = Unbundle By Name(w1854) -> ("Kpro box Serial"=w1844:string)
                        n790 = Scan From String(format string="%d", input string=w1844, error in=w1848, default 1=800.0 ("default value 1")) -> (error out=w1849:errorcluster, output 1=w1853:dbl)  [unwired: 1 in, 2 out]
                        n791 = Equal?(x=w1844, y="") -> (x = y?=w1845:bool)
                        n792 = case shown="False" w1845 {
                          tunnel: "KPRO Box Number\n\nEnter the number of the KPRO box you are using." ("prompt") -> [_ w1867]
                          tunnel: w1854 -> [w1858 w1866]
                          tunnel: w1853 -> [w1856 w1865]
                          tunnel: [w1856 w1864] -> w1852
                          tunnel: [w1858 w1862] -> w1850
                          tunnel: w1849 -> [w1857 w1860]
                          tunnel: [w1857 w1859] -> w1847
                          frame False {
                          }
                          frame True {
                            n793 = call "prompt_and_enter_value2.vi"("prompt_IN"=w1867, "Enter value"=w1865) -> ("Numeric"=w1864:dbl)  [unwired: 9 in]
                            n794 = Format Into String(format string="%d", error in=w1860, w1864) -> (resulting string=w1861:string, error out=w1859:errorcluster)  [unwired: 1 in]
                            n795 = Bundle By Name(cluster=w1866, "Kpro box Serial"=w1861) -> (w1862:T10)
                          }
                        }
                        n796 = global write "Kpro Globals.vi" "KPRO Box Number"(w1852) -> ()
                        n797 = local write "Groundwater Header"(w1850) -> ()
                      }
                    }
                    "Initialization" <- 0
                  }
                  frame #1 {
                    n798 = local write "Initialization"(1 ("Initialization")) -> ()
                    n799 = flat-sequence {
                      tunnel: w1868 -> [w1876]
                      tunnel: [w1875] -> w1869
                      frame #0 {
                        n800 = local read "Groundwater Header"() -> (w1877:T10)
                        n801 = Build Array("Profile ID   " ("string"), "Depth    " ("string"), "Flow " ("string"), "Ik    " ("string")) -> (w1880:string[])
                        n802 = Unbundle By Name(w1877) -> ("Profile ID"=w1872:string)
                        n803 = call-poly <vilib>:"Write Delimited Spreadsheet.vi"("file path (dialog if empty)"="Static IK path", "1D data"=w1880, "append to file? (new file:F)"=TRUE, "error in (no error)"=w1876, "delimiter (\\t)"="," ("delimiter (\\t)")) -> ("error out"=w1875:errorcluster)  [unwired: 9 in, 1 out]
                        n804 = Equal?(x=w1872, y="") -> (x = y?=w1873:bool)
                        n805 = case shown="True" w1873 {
                          tunnel: "Profile ID\n\nEnter the profile ID" ("prompt") -> [_ w1891]
                          tunnel: [w1888 w1890] -> w1878
                          tunnel: w1872 -> [w1888 w1889]
                          frame False {
                          }
                          frame True {
                            n806 = call "prompt_string.vi"("prompt_IN"=w1891, "Enter value"=w1889) -> ("String"=w1890:string)  [unwired: 9 in]
                            n807 = global write "Kpro Globals.vi" "Profile ID"(w1890) -> ()
                          }
                        }
                        n808 = Bundle By Name(cluster=w1877, "Profile ID"=w1878) -> (w1879:T10)
                        n809 = local write "Groundwater Header"(w1879) -> ()
                      }
                    }
                  }
                  frame #2 {
                    n810 = flat-sequence {
                      tunnel: [w1915] -> w1897
                      tunnel: w1893 -> [w1923]
                      tunnel: w1895 -> [w1921]
                      tunnel: w1894 -> [w1920]
                      tunnel: [w1919] -> w1892
                      frame #0 {
                        w1912 = "_KPRO.csv"
                        n811 = local read "Input Variables and Slopes"() -> (w1928:T16)
                        n812 = local read "Temporary Data Files Directory"() -> (w1922:path)
                        n813 = Unbundle By Name(w1928) -> ("Up Hole Pressure Slope"=w1931:dbl, "String Pot Slope"=w1930:dbl, "Flow Slope"=w1929:dbl)
                        n814 = call "FILE_DIALOG 2016.vi"("flow_slope_IN"=w1929, "pressure_slope_IN"=w1931, "string_pot_slope_IN"=w1930, "Descriptions"=w1920, "error in (no error)"=w1923, "start path"=w1922, "Array in"=w1921) -> ("path"=w1907:path, "exists"=w1918:bool, "flow_slope_OUT"=w1926:dbl, "pressure_slope_OUT"=w1925:dbl, "string_pot_slope_OUT"=w1927:dbl, "error out"=w1914:errorcluster)  [unwired: 5 in, 2 out]
                        n815 = global write "Kpro Globals.vi" "Flow Slope"(w1926) -> ()
                        n816 = Bundle By Name(cluster=w1928, "String Pot Slope"=w1927, "Flow Slope"=w1926, "Up Hole Pressure Slope"=w1925) -> (w1916:T16)
                        n817 = global write "Kpro Globals.vi" "Pressure \nSlope"(w1925) -> ()
                        n818 = global write "Kpro Globals.vi" "String Pot \nSlope"(w1927) -> ()
                        n819 = Path To String(path=w1907) -> (string=w1909:string)
                        n820 = call-poly "Strip Path Extension__ogtk.vi"("path"=w1907) -> ("root"=w1908:string, "extension"=w1906:string)
                        n821 = Match Pattern(string=w1909, regular expression=w1912) -> (offset past match=w1911:i32)  [unwired: 1 in, 3 out]
                        n822 = String Length(string=w1906) -> (length=w1905:i32)
                        n823 = Equal?(x=w1911, y=-1) -> (x = y?=w1903:bool)
                        n824 = Equal To 0?(x=w1905) -> (x = 0?=w1904:bool)
                        n825 = local write "Input Variables and Slopes"(w1916) -> ()
                        n826 = Or(x=w1903, y=w1904) -> (x .or. y?=w1902:bool)
                        n827 = case shown="False" w1902 {
                          tunnel: [w1932 w1938] -> w1917
                          tunnel: w1908 -> [_ w1936]
                          tunnel: w1912 -> [_ w1937]
                          tunnel: w1907 -> [w1932 _]
                          tunnel: [w1932 w1933] -> w1898
                          frame False {
                          }
                          frame True {
                            n828 = Concatenate Strings(w1936, ".csv" ("string")) -> (w1934:string)
                            n829 = Concatenate Strings(w1936, w1937) -> (w1939:string)
                            n830 = String To Path(string=w1934) -> (path=w1933:path)
                            n831 = String To Path(string=w1939) -> (path=w1938:path)
                          }
                        }
                        "Output File Path" <- w1898
                        "KPRO Output File Path" <- w1917
                        n832 = call <vilib>:"Check if File or Folder Exists.vi"("path"=w1917) -> ("file or folder exists?"=w1899:bool, "dup path"=w1901:path)  [unwired: 8 in, 1 out]
                        n833 = And(x=w1899, y=w1918) -> (x .and. y?=w1900:bool)
                        n834 = case shown="True" w1900 {
                          selector: w1900 -> [_ w1942]
                          tunnel: w1901 -> [_ w1956]
                          tunnel: w1916 -> [w1941 w1951]
                          tunnel: [w1941 w1950] -> w1915
                          tunnel: w1914 -> [w1940 w1943]
                          tunnel: [w1940 w1943] -> w1913
                          frame False {
                          }
                          frame True {
                            n835 = local read "Culmulative Graph Cluster"() -> (w1955:T19)
                            n836 = local read "Depth Cluster"() -> (w1947:T17)
                            n837 = call "Get_KPRO_data_from_file 2016.vi"("Output File KPRO Test"=w1956) -> ("Last_height_of_box"=w1948:dbl, "Last_depth_to_water"=w1949:dbl, "Last_depth"=w1945:dbl, "Output_array"=w1944:sgl[][])  [unwired: 7 in]
                            "Cumulative_data_from_file" <- w1944
                            n838 = Bundle By Name(cluster=w1951, "Depth to Water Table"=w1949, "Height of Sample Box"=w1948) -> (w1950:T16)
                            n839 = Bundle By Name(cluster=w1947, "Absolute Depth In"=w1945, "Current Absolute Depth"=w1945) -> (w1946:T17)
                            n840 = local write "Depth Cluster"(w1946) -> ()
                            n841 = call "Array to Plot 2016.vi"("Input Cumulative Array"=w1944) -> ("Cumulative - Depth vs.Drive Rate"=w1952:cluster{dbl[], dbl[]}, "Cumulative - Depth vs. Ik"=w1953:cluster{dbl[], dbl[]})  [unwired: 3 in, 4 out]
                            n842 = Bundle By Name(cluster=w1955, "Cumulative - Depth vs. Ik"=w1953, "Cumulative - Depth vs. Drive Rate"=w1952) -> (w1954:T19)
                            n843 = local write "Culmulative Graph Cluster"(w1954) -> ()
                            n844 = local write "Input Variables and Slopes"(w1950) -> ()
                            "Cumulative_data_ready" <- w1942
                          }
                        }
                        n845 = global read "Global_SIM_switch.vi" "enable_kpro_file"() -> (w1924:bool)
                        n846 = case shown="True" w1924 {
                          tunnel: w1917 -> [_ w1964]
                          tunnel: w1913 -> [w1957 w1961]
                          tunnel: [w1957 w1960] -> w1919
                          frame False {
                          }
                          frame True {
                            n847 = call-poly <vilib>:"Write Delimited Spreadsheet.vi"("file path (dialog if empty)"=w1964, "1D data"="KPRO test report header", "append to file? (new file:F)"=FALSE, "error in (no error)"=w1961, "transpose? (no:F)"=FALSE, "delimiter (\\t)"="," ("delimiter (\\t)")) -> ("error out"=w1960:errorcluster)  [unwired: 8 in, 1 out]
                          }
                        }
                      }
                    }
                    n848 = local write "Initialization"(2 ("Initialization")) -> ()
                  }
                  frame #3 {
                    # "Take offset and put\n into Pressure VI."
                    n849 = local read "Groundwater Header"() -> (w1969:T10)
                    n850 = local write "Initialization"(3 ("Initialization")) -> ()
                    n851 = local read "Input Variables and Slopes"() -> (w1967:T16)
                    n852 = Unbundle By Name(w1969) -> ("Atmospheric Pressure"=w1965:string)
                    n853 = Equal?(x=w1965, y="") -> (x = y?=w1966:bool)
                    n854 = case shown="False" w1966 {
                      tunnel: "ATMOSPHERIC PRESSURE READING\n\nHold Kpro effluent facing up and level with the pressure transducer.\nTurn on Kpro water, turn off when water flows with no air bubbles.\n\nPress OK when the reading equilibrates." ("message") -> [_ w2003]
                      tunnel: [w1994 w2002] -> w1985
                      tunnel: [w1993 w1995] -> w1981
                      tunnel: w1978 -> [_ w2001]
                      tunnel: w1977 -> [w1991 w2000]
                      tunnel: [w1992 w1999] -> w1976
                      tunnel: [w1988 w1997] -> w1971
                      tunnel: [w1991 w1996] -> w1970
                      tunnel: w1967 -> [w1993 w1995]
                      tunnel: w1965 -> [w1989 _]
                      frame False {
                        n855 = local read "Sensor Voltage Cluster"() -> (w1994:T9)
                        n856 = Unbundle By Name(w1993) -> ("Up Hole Pressure Slope"=w1992:dbl)
                        n857 = Scan From String(input string=w1989, default 1=35.0 ("default value 1")) -> (output 1=w1988:dbl)  [unwired: 3 in, 3 out]
                      }
                      frame True {
                        n858 = local read "Sensor Voltage Cluster"() -> (w2002:T9)
                        n859 = Unbundle By Name(w1995) -> ("Up Hole Pressure Slope"=w1999:dbl)
                        n860 = global read "Kpro Globals.vi" "Pressure Offset"() -> (w1998:dbl)
                        n861 = call "Up Hole PRESSURE_CAL 2016.vi"("Pressure Offset"=w1998, "Descriptions"=w2001, "Array in"=w2000, "Pressure \nSlope"=w1999, "Sensor Cluster"=w2002, "Prompt_IN"=w2003) -> ("PRESSURE\nFt of water"=w1997:dbl, "Array out"=w1996:refnum<k24>[])  [unwired: 4 in]
                      }
                    }
                    n862 = local read "Corrected Pressure Cluster"() -> (w1984:T20)
                    n863 = global write "Kpro Globals.vi" "Atmospheric Pressure"(w1971) -> ()
                    n864 = Bundle By Name(cluster=w1981, "Atmospheric Pressure"=w1971) -> (w1980:T16)
                    n865 = Format Into String(w1971) -> (resulting string=w1972:string)  [unwired: 3 in, 1 out]
                    n866 = call "up hole Pressure 2016.vi"("Sensor Cluster"=w1985, "Pressure Offset"=w1971, "Array in"=w1970, "Pressure \nSlope"=w1976, "Descriptions"=w1978, "Zero Pressure\n(F = leave as is)"=TRUE) -> ("Array out"=w1979:refnum<k24>[], "Uphole Pressure"=w1982:dbl, "Sensor Cluster 2"=w1974:T9)  [unwired: 7 in]
                    n867 = Bundle By Name(cluster=w1969, "Atmospheric Pressure"=w1972) -> (w1973:T10)
                    n868 = Bundle By Name(cluster=w1984, "Up hole Corrected Pressure"=w1982) -> (w1983:T20)
                    n869 = local write "Sensor Voltage Cluster"(w1974) -> ()
                    n870 = local write "Input Variables and Slopes"(w1980) -> ()
                    n871 = local write "Groundwater Header"(w1973) -> ()
                    n872 = local write "Corrected Pressure Cluster"(w1983) -> ()
                  }
                  frame #4 {
                    n873 = disable-structure shown="Disabled" {
                      disable-tunnel: w2005 -> [w2009 _]
                      disable-tunnel: w2004 -> [w2008 _]
                      frame Disabled {
                        w2017 = 0.0  # Offset
                        (unwired) FALSE
                        # "Take offset and put\n into Pressure VI."
                        n874 = local write "Initialization"(4 ("Initialization")) -> ()
                        n875 = local read "Input Variables and Slopes"() -> (w2016:T16)
                        n876 = local read "Input Variables and Slopes"() -> (w2023:T16)
                        n877 = local read "Input Variables and Slopes"() -> (w2015:T16)
                        n878 = local read "Input Variables and Slopes"() -> (w2014:T16)
                        n879 = local read "Sensor Voltage Cluster"() -> (w2019:T9)
                        n880 = Unbundle By Name(w2016) -> ()  [unwired: 2 out]
                        n881 = Unbundle By Name(w2019) -> ()  [unwired: 1 out]
                        n882 = Unbundle By Name(w2023) -> ("Up Hole Pressure Slope"=w2010:dbl, "Flow Slope"=w2018:dbl)
                        n883 = Unbundle By Name(w2015) -> ()  [unwired: 2 out]
                        n884 = Unbundle By Name(w2014) -> ()  [unwired: 2 out]
                        n885 = call "Up Hole PRESSURE_CAL 2016.vi"("Descriptions"=w2008, "Array in"=w2009, "Pressure \nSlope"=w2010, "Sensor Cluster"=w2019, "Prompt_IN"="ZERO PRESSURE TRANSDUCER\n\nHold Kpro effluent in a grad cylinder with 800mL (1 ft) of water.\nHold grad cylinder with its bottom level with the pressure transducer.\n\nPress OK when the reading equilibrates. " ("message")) -> ("PRESSURE\nFt of water"=w2024:dbl)  [unwired: 5 in, 1 out]
                        n886 = call "Flow 2016.vi"("Descriptions"=w2008, "Array in"=w2009, "Flow Slope"=w2018, "Offset"=w2017) -> ("Flow (ml/min)"=w2011:dbl)  [unwired: 4 in, 2 out]
                        n887 = local read item#-1() -> (w2013)
                        n888 = Subtract(x=w2024, y=1.0) -> (x-y=w2027:dbl)
                        n889 = Bundle By Name(cluster=w2013, "Flow"=w2011) -> (w2012:cluster{})
                        n890 = call "up hole Pressure 2016.vi"("Sensor Cluster"=w2019, "Pressure Offset"=w2027, "Array in"=w2009, "Pressure \nSlope"=w2010, "Descriptions"=w2008, "Zero Pressure\n(F = leave as is)"=TRUE) -> ("Uphole Pressure"=w2020:dbl, "Sensor Cluster 2"=w2006:T9)  [unwired: 7 in, 1 out]
                        n891 = local write "Sensor Voltage Cluster"(w2006) -> ()
                        n892 = local write item#-1(w2012) -> ()
                        n893 = local read "Corrected Pressure Cluster"() -> (w2022:T20)
                        n894 = Bundle By Name(cluster=w2022, "Up hole Corrected Pressure"=w2020) -> (w2021:T20)
                        n895 = local write "Corrected Pressure Cluster"(w2021) -> ()
                      }
                      frame Enabled {
                      }
                    }
                  }
                  frame #5 {
                    n896 = local write "Initialization"(5 ("Initialization")) -> ()
                    n897 = flat-sequence {
                      tunnel: w2031 -> [w2040]
                      tunnel: w2030 -> [w2039]
                      frame #0 {
                        n898 = local read "Input Variables and Slopes"() -> (w2038:T16)
                        n899 = Unbundle By Name(w2038) -> ("Up Hole Pressure Slope"=w2037:dbl)
                        n900 = local read "Sensor Voltage Cluster"() -> (w2043:T9)
                        n901 = global read "Kpro Globals.vi" "Pressure Offset"() -> (w2036:dbl)
                        n902 = call "Up Hole PRESSURE_CAL 2016.vi"("Pressure Offset"=w2036, "Descriptions"=w2039, "Array in"=w2040, "Pressure \nSlope"=w2037, "Sensor Cluster"=w2043, "Prompt_IN"="CHECK RESERVOIR PRESSURE\n\nTurn on Kpro. Unplug Kpro Out quick connect from sample box.\nReservoir pressure should be 69.2 +/- 5%(65.7 - 72.7).\n\nPress OK when the reading equilibrates within range." ("message")) -> ("PRESSURE\nFt of water"=w2033:dbl)  [unwired: 4 in, 1 out]
                        n903 = local read "Groundwater Header"() -> (w2035:T10)
                        n904 = Format Into String(w2033) -> (resulting string=w2032:string)  [unwired: 3 in, 1 out]
                        n905 = global write "Kpro Globals.vi" "Reservoir Pressure"(w2033) -> ()
                        n906 = Bundle By Name(cluster=w2038, "Reservoir Pressure"=w2033) -> (w2041:T16)
                        n907 = Bundle By Name(cluster=w2035, "KPRO N2 Pressure"=w2032) -> (w2034:T10)
                        n908 = local write "Input Variables and Slopes"(w2041) -> ()
                        n909 = local write "Groundwater Header"(w2034) -> ()
                      }
                    }
                  }
                  frame #6 {
                    n910 = local write "Initialization"(6 ("Initialization")) -> ()
                    n911 = flat-sequence {
                      frame #0 {
                        n912 = local read "Input Depths \nand Parameters Cluster"() -> (w2049:T15)
                        n913 = Unbundle By Name(w2049) -> ("Start Depth"=w2046:sgl)
                        n914 = call "prompt_and_enter_value 2016.vi"("prompt_IN"="ENTER START DEPTH", "Enter value"=w2046) -> ("Numeric"=w2051:dbl)  [unwired: 9 in]
                        n915 = Absolute Value(x=w2051) -> (abs(x)=w2050:dbl)
                        n916 = Negate(x=w2050) -> (-x=w2047:dbl)
                        n917 = Bundle By Name(cluster=w2049, "Start Depth"=w2047) -> (w2048:T15)
                        n918 = local write "Input Depths \nand Parameters Cluster"(w2048) -> ()
                      }
                    }
                  }
                  frame #7 {
                    n919 = local write "Initialization"(7 ("Initialization")) -> ()
                    n920 = local read "Input Variables and Slopes"() -> (w2057:T16)
                    n921 = Unbundle By Name(w2057) -> ("Height of Sample Box"=w2055:dbl)
                    n922 = call "prompt_and_enter_value 2016.vi"("prompt_IN"="HEIGHT FROM GROUND SURFACE TO SAMPLE BOX\n\nMeasure the vertical distance between the ground surface and the pressure transducer." ("prompt"), "Enter value"=w2055) -> ("Numeric"=w2054:dbl)  [unwired: 9 in]
                    n923 = Bundle By Name(cluster=w2057, "Height of Sample Box"=w2054) -> (w2056:T16)
                    n924 = global write "Kpro Globals.vi" "height_of_box"(w2054) -> ()
                    n925 = local write "Input Variables and Slopes"(w2056) -> ()
                  }
                  frame #8 {
                    n926 = local write "Initialization"(8 ("Initialization")) -> ()
                    n927 = flat-sequence {
                      frame #0 {
                        n928 = local read "Input Variables and Slopes"() -> (w2062:T16)
                        n929 = Unbundle By Name(w2062) -> ("Depth to Water Table"=w2063:dbl)
                        n930 = call "prompt_and_enter_value 2016.vi"("prompt_IN"="DEPTH TO WATER TABLE\n\nEnter the depth to the water table." ("prompt"), "Enter value"=w2063) -> ("Numeric"=w2065:dbl)  [unwired: 9 in]
                        n931 = Absolute Value(x=w2065) -> (abs(x)=w2064:dbl)
                        n932 = Negate(x=w2064) -> (-x=w2061:dbl)
                        n933 = global write "Kpro Globals.vi" "Depth to Water Table"(w2061) -> ()
                        n934 = Bundle By Name(cluster=w2062, "Depth to Water Table"=w2061) -> (w2060:T16)
                        n935 = local write "Input Variables and Slopes"(w2060) -> ()
                      }
                    }
                  }
                  frame #9 {
                    n936 = local write "Initialization"(9 ("Initialization")) -> ()
                    n937 = local read "Input Variables and Slopes"() -> (w2071:T16)
                    n938 = Unbundle By Name(w2071) -> ("Up Hole Pressure Slope"=w2069:dbl)
                    n939 = stacked-sequence {
                      tunnel: [_ w2091] -> w2072
                      tunnel: w2069 -> [w2081 w2090]
                      tunnel: w2068 -> [w2076 w2089]
                      tunnel: w2070 -> [w2075 w2085]
                      tunnel: w2069 -> [_ w2088]
                      tunnel: w2068 -> [_ w2086]
                      frame #0 {
                        # "Set to raw pressure mode"
                        n940 = local read "Sensor Voltage Cluster"() -> (w2080:T9)
                        n941 = local read "Corrected Pressure Cluster"() -> (w2078:T20)
                        n942 = call "up hole Pressure 2016.vi"("Sensor Cluster"=w2080, "Pressure Offset"=0.0, "Array in"=w2075, "Pressure \nSlope"=w2081, "Descriptions"=w2076, "Zero Pressure\n(F = leave as is)"=TRUE) -> ("Uphole Pressure"=w2079:dbl)  [unwired: 7 in, 2 out]
                        n943 = Bundle By Name(cluster=w2078, "Up hole Corrected Pressure"=w2079) -> (w2077:T20)
                        n944 = local write "Corrected Pressure Cluster"(w2077) -> ()
                      }
                      frame #1 {
                        # "adjust for 1 foot head"
                        # "Take offset and put\n into Pressure VI."
                        n945 = local read "Sensor Voltage Cluster"() -> (w2092:T9)
                        n946 = global read "Kpro Globals.vi" "Pressure Offset"() -> (w2087:dbl)
                        n947 = call "Up Hole PRESSURE_CAL 2016.vi"("Pressure Offset"=w2087, "Descriptions"=w2086, "Array in"=w2085, "Pressure \nSlope"=w2088, "Sensor Cluster"=w2092, "Prompt_IN"="ZERO TO GROUND SURFACE\n\nFill a grad cylinder to 750mL.\nPlace it on the ground at the profile location.\nImmerse the Kpro effluent and turn on Kpro flow.\nTurn off after water is flowing with no bubbles\nand the water has reached 800mL (1 foot).\n\nPress OK when the reading equilibrates." ("message")) -> ("PRESSURE\nFt of water"=w2093:dbl)  [unwired: 4 in, 1 out]
                        n948 = Decrement(x=w2093) -> (x-1=w2084:dbl)
                        n949 = call "up hole Pressure 2016.vi"("Sensor Cluster"=w2092, "Pressure Offset"=w2084, "Array in"=w2085, "Pressure \nSlope"=w2090, "Descriptions"=w2089, "Zero Pressure\n(F = leave as is)"=TRUE) -> ("Uphole Pressure"=w2091:dbl)  [unwired: 7 in, 2 out]
                      }
                    }
                    n950 = local read "Corrected Pressure Cluster"() -> (w2074:T20)
                    n951 = Bundle By Name(cluster=w2074, "Up hole Corrected Pressure"=w2072) -> (w2073:T20)
                    n952 = local write "Corrected Pressure Cluster"(w2073) -> ()
                  }
                  frame #10 {
                    n953 = local write "Initialization"(10 ("Initialization")) -> ()
                    n954 = local read "Cumulative_data_ready"() -> (w2101:bool)
                    n955 = case shown="True" w2101 {
                      tunnel: w2100 -> [w2102 _]
                      tunnel: [w2102 w2103] -> w2099
                      frame False {
                      }
                      frame True {
                        n956 = local write "Cumulative_data_ready"(FALSE ("Get_KPRO_data")) -> ()
                        n957 = local read "Cumulative_data_from_file"() -> (w2103:sgl[][])
                      }
                    }
                    "Zero Pressure\nIndicator" <- FALSE ("Zero Pressure\nIndicator")
                  }
                }
              }
              frame Disabled {
              }
            }
            n958 = flat-sequence {
              tunnel: "Read String Pot" -> [_]
              tunnel: [w2143] -> w1813
              tunnel: w1820 -> [w2127]
              tunnel: w1816 -> [w2128]
              frame #0 {
                w2133 = 0.0
                w2134 = TRUE
                # "Initialize Incrementer if using hand incrementer,\nDon't use Debug,\nPut use string pot into shift register first pass to avoid allowing\na change in which method is the source of the depth reading."
                n959 = global write "Global_SIM_switch.vi" "enable_kpro_file"("enable_kpro_file") -> ()
                n960 = global write "Global_SIM_switch.vi" "Simulate AD6B"("Simulate AD6B") -> ()
                n961 = global write "Global_SIM_switch.vi" "enable_slug_file"("enable_slug_file") -> ()
                n962 = local read "Input Variables and Slopes"() -> (w2141:T16)
                n963 = global write "Global_SIM_switch.vi" "enable_IKMGS_file"("enable_IKMGS_file") -> ()
                n964 = Unbundle By Name(w2141) -> ("String Pot Slope"=w2140:dbl, "Up Hole Pressure Slope"=w2136:dbl)  [unwired: 1 out]
                n965 = local read "Sensor Voltage Cluster"() -> (w2135:T9)
                n966 = local read "Descriptions"() -> (w2126:string[])
                n967 = local read "Sensor Voltage Cluster"() -> (w2142:T9)
                n968 = call "In-Line-Pressure 2016.vi"("Zero Pressure\n(F = leave as is)"=w2134, "In-Line Pressure Slope"=w2136, "Sensor Voltages Cluster"=w2135, "In-Line Pressure Offset"=w2133) -> ("Pressure"=w2137:dbl)  [unwired: 7 in]
                n969 = call "up hole Pressure 2016.vi"("Sensor Cluster"=w2135, "Pressure Offset"=w2133, "Array in"=w2128, "Pressure \nSlope"=w2136, "Descriptions"=w2126, "Zero Pressure\n(F = leave as is)"=w2134) -> ("Array out"=w2125:refnum<k24>[], "Uphole Pressure"=w2122:dbl)  [unwired: 7 in, 1 out]
                n970 = Bundle By Name(cluster="Corrected Pressure Cluster", "Up hole Corrected Pressure"=w2122, "Down hole Corrected Pressure"=w2137) -> (w2138:T20)
                n971 = call "depth read from string pot 2016.vi"("Descriptions"=w2126, "error in (no error)"=w2127, "String Pot \nSlope"=w2140, "Array in"=w2125, "Sensor Cluster In"=w2142) -> ("Depth"=w2144:dbl)  [unwired: 11 in, 3 out]
                n972 = local read "Sample Sheet Data Row Cluster 2"() -> (w2124:T1)
                n973 = local write "Corrected Pressure Cluster"(w2138) -> ()
                n974 = flat-sequence {
                  tunnel: w2144 -> [w2146]
                  tunnel: [w2145] -> w2143
                  frame #0 {
                    w2147 = 15  # Filter Size
                    # "Functional Global in \nBoxcar Integrator\nInitialize filter array to \ncurrent string pot value"
                    n975 = call "Boxcar filter2016.vi"("Initialize"=TRUE, "Filter Size"=w2147, "Filter Input"=w2146) -> ("Filter Output"=w2145:dbl)
                  }
                }
                n976 = Bundle By Name(cluster=w2124, "Head\nPressure"=w2122) -> (w2123:T1)
                n977 = local write "Sample Sheet Data Row Cluster 2"(w2123) -> ()
              }
            }
            n978 = flat-sequence {
              tunnel: [w2109] -> w1821
              tunnel: [w2108] -> w1814
              tunnel: w1813 -> [w2106]
              tunnel: [w2106] -> w1810
              frame #0 {
                n979 = local read "Input Depths \nand Parameters Cluster"() -> (w2107:T15)
                n980 = Unbundle By Name(w2107) -> ("Start Depth"=w2110:sgl)
                n981 = Less Or Equal To 0?(x=w2110) -> (x <= 0?=w2112:bool)
                n982 = Negate(x=w2110) -> (-x=w2111:sgl)
                n983 = Select(t=w2110, s=w2112, f=w2111) -> (s? t:f=w2108:sgl)
                n984 = Bundle By Name(cluster=w2107, "Abs Start Depth"=w2108, "Current Depth"=w2106) -> (w2109:T15)
                n985 = local write "Input Depths \nand Parameters Cluster"(w2109) -> ()
              }
            }
            n986 = flat-sequence {
              tunnel: [w2119] -> w1823
              frame #0 {
                n987 = Tick Count (ms)() -> (millisecond timer value=w2121:u32)
                n988 = Divide(x=w2121, y=u32 1000) -> (x/y=w2119:dbl)
              }
            }
            n989 = flat-sequence {
              tunnel: [w2113] -> w1822
              tunnel: w1823 -> [w2117]
              tunnel: [w2115] -> _
              tunnel: w1814 -> [w2115]
              tunnel: w1810 -> [w2114]
              frame #0 {
                n990 = local read "Depth Cluster"() -> (w2116:T17)
                n991 = Bundle By Name(cluster=w2116, "Absolute Depth In"=w2115, "Previous Relative Depth"=w2114, "Current Relative Depth"=w2114, "First Relative Depth"=w2114, "Current Absolute Depth"=w2115, "Last Filed Depth"=0.0, "Current Measurement Time"=w2117, "Previous Measurement Time"=w2117, "First Absolute Depth"=w2115) -> (w2113:T17)
                n992 = local write "Depth Cluster"(w2113) -> ()
              }
            }
          }
          frame "Acq. DAQ data" {
            n993 = flat-sequence {
              tunnel: w2193 -> [w2210]
              tunnel: w2192 -> [w2209]
              tunnel: [w2206] -> w2191
              frame #0 {
                n994 = local read "Descriptions"() -> (w2207:string[])
                n995 = local read "Sensor  Real Measurements"() -> (w2205:T6)
                n996 = local read "Input Variables and Slopes"() -> (w2203:T16)
                n997 = call "Measure DAQ Voltages.vi"("error in (no error)"=w2209, "Descriptions"=w2207, "Array in"=w2210) -> ("Raw Voltages"=→"Raw Voltages":dbl[], "Array out"=w2206:refnum<k24>[], "Sensor Cluster"=w2202:T9)  [unwired: 6 in]
                "Sensor Voltage Cluster" <- w2202
                n998 = call "convert sensor voltage to real measurements.vi"("Input Variables and Slopes"=w2203, "Sensor  Real Measurements in"=w2205, "Sensor Cluster"=w2202) -> ("Sensor  Real Measurements out"=w2204:T9)  [unwired: 8 in]
                n999 = local write "Sensor  Real Measurements"(w2204) -> ()
              }
            }
          }
          frame "Exit" {
            n1000 = flat-sequence {
              tunnel: [w2236] -> _
              tunnel: [w2243] -> w2213
              tunnel: w2216 -> [w2238]
              tunnel: w2215 -> [w2236]
              tunnel: [w2235] -> w2214
              frame #0 {
                w2242 = "Groundwater Profile Log" ("Worksheet Name in")
                n1001 = local read "Worksheet Names"() -> (w2240:string[])
                n1002 = local write "Current Sample Sheet"(w2242) -> ()
                n1003 = call "find and open select worksheet.vi"("Worksheet Names"=w2240, "error in (no error)"=w2236, "milliseconds to wait"=u32 100, "Worksheet Name in"=w2242, "NI_report in"=w2238) -> ("error out"=w2239:errorcluster, "NI_report out"=w2237:refnum<class "NI_report.lvclass">)  [unwired: 4 in, 1 out]
                n1004 = call "groundwater log header.vi"("Worksheet Names"=w2240, "Groundwater Header"="Groundwater Header", "error in (no error)"=w2239, "NI_report in"=w2237) -> ("error out"=w2235:errorcluster, "NI_report out"=w2243:refnum<class "NI_report.lvclass">)  [unwired: 6 in]
              }
            }
            n1005 = case shown="No Error" w2224 {
              tunnel: w2220 -> [w2267 _]
              tunnel: w2224 -> [w2266 w2278]
              tunnel: [w2265 w2278] -> w2222
              frame No Error {
                n1006 = for {
                  shift-right: [w2269] -> w2265
                  shift-left: w2266 -> [w2270]
                  tunnel: w2267 -> [w2268] mode=indexing
                  n1007 = while {
                    shift-right: [w2277] -> w2272
                    shift-left: w2270 -> [w2275]
                    shift-right: [w2276] -> w2271
                    shift-left: w2268 -> [w2274]
                    stop <- w2273 stop-if-true
                    n1008 = call <vilib>:"ULx Is Task Done.vi"("task in"=w2274, "error in"=w2275) -> ("task out"=w2276:refnum<k24>, "task done?"=w2273:bool, "error out"=w2277:errorcluster)  [unwired: 11 in]
                  }
                  n1009 = call <vilib>:"ULx Clear Task.vi"("task in"=w2271, "error in"=w2272) -> ("error out"=w2269:errorcluster)  [unwired: 13 in]
                }
              }
              frame Error {
              }
            }
            n1010 = flat-sequence {
              tunnel: [w2284] -> w2231
              tunnel: [w2283] -> w2232
              tunnel: w2214 -> [w2281]
              tunnel: w2213 -> [w2280]
              frame #0 {
                n1011 = local read "Excel report file path"() -> (w2279:path)
                n1012 = call-dynamic "Save Report to File.vi"("report in"=w2280, "report file path"=w2279, "prompt to replace? (F)"=FALSE, "error in (no error)"=w2281) -> ("report out"=w2284:refnum<class "NI_report.lvclass">, "error out"=w2283:errorcluster)  [unwired: 10 in]
              }
            }
            n1013 = call "Wait (ms)__ogtk.vi"("error in (no error)"=w2232, "milliseconds to wait"=u32 5) -> ("error out"=w2233:errorcluster)  [unwired: 8 in, 1 out]
            n1014 = flat-sequence {
              tunnel: w2233 -> [w2253]
              tunnel: w2231 -> [w2251]
              tunnel: [w2249] -> w2225
              frame #0 {
                (unwired) FALSE ("Write Ini")
                n1015 = call-dynamic "Dispose Report.vi"("report in"=w2251, "save changes? (F)"=FALSE, "error in (no error)"=w2253) -> ("error out"=w2248:errorcluster)  [unwired: 12 in]
                n1016 = case shown="False" "Save Configuration File?" {
                  tunnel: [errorcluster {"status"=FALSE, "code"=0, "source"=""} ("error IO") w2262] -> w2250
                  frame False {
                  }
                  frame True {
                    n1017 = local read "Config File Path"() -> (w2261:path)
                    n1018 = call <vilib>:"Open Config Data.vi"("create file if necessary (T)"=TRUE ("Read Ini"), "configuration file path"=w2261) -> ("error out"=w2259:errorcluster, "refnum"=w2256:T21)  [unwired: 7 in, 1 out]
                    n1019 = control-ref of="This VI"() -> (w2255:refnum<vi>)
                    n1020 = call "Write Panel to INI__ogtk.vi"("error in (no error)"=w2259, "VI ref"=w2255, "refnum"=w2256) -> ("error out"=w2258:errorcluster, "refnum out"=w2257:T21)  [unwired: 7 in]
                    n1021 = call <vilib>:"Clear Errors.vi"("error in (no error)"=w2258) -> ("error out"=w2264:errorcluster)  [unwired: 5 in, 1 out]
                    n1022 = call <vilib>:"Close Config Data.vi"("error in (no error)"=w2264, "refnum"=w2257) -> ("error out"=w2263:errorcluster)  [unwired: 8 in, 1 out]
                    n1023 = Merge Errors(w2263, w2258) -> (w2262:errorcluster)
                  }
                }
                n1024 = Merge Errors(w2250, w2248) -> (w2249:errorcluster)
              }
            }
            n1025 = flat-sequence {
              tunnel: [TRUE ("aborted?")] -> w2223
              tunnel: [w2245] -> w2221
              tunnel: w2222 -> [w2245]
              frame #0 {
              }
            }
          }
        }
        "Stop 2" <- w425
        "consumer loop" <- w407
      }
    }
  }
  n1026 = Get Date/Time In Seconds() -> (seconds since 1Jan1904=w8:timestamp)
  n1027 = To Double Precision Float(number=w8) -> (double precision float=w7:dbl)
  n1028 = Merge Errors(w19, w18) -> (→"error out":errorcluster)
